vi "MC_8_28_12a_JW.vi"() -> ()   [LabVIEW 2011]
uses:
  <vilib>/Utility/file.llb/Read From Spreadsheet File (string).vi
  <vilib>/Utility/inputDevices.llb/keyboardAcquire.vi
  <vilib>/Utility/file.llb/Write To Spreadsheet File (DBL).vi
  <vilib>/Utility/file.llb/Write To Spreadsheet File (string).vi
  <vilib>/regexp/Match Regular Expression.xnode
panel:
  out "Vg Column":dbl[](array[numeric])
  out "Data Length":dbl
  in  "default (0 dbl) 6":ext format="%.2e"
  in  "default (0 dbl) 5":ext format="%.2e"
  in  "default (0 dbl) 4":ext format="%.2e"
  in  "default (0 dbl) 3":ext format="%.2e"
  in  "default (0 dbl)":ext format="%.2e"
  out "X Axis Display Type":string
  out "Opj X Axis":string
  in  "Room Temp":dbl=294.0
  out "No Image 2":path=path "\\\\acad1\\physics/Jurchescu-group/JW-PD/Image Not Found.png"
  out "Save1 Array":string[][](array[string])
  out "Lin Vd":dbl
  out "Lin-Vg Array-Used":dbl[](array[numeric])
  out "Lin Id-Used":dbl[](array[numeric])
  out "Rec: Comments":string
  out "Folder Index":dbl caption="Length"
  out "Current \nRecord":string[](array[string])
  out "Transformer \nHeaders":string[](array[string])
  out "Current Device ID":string
  out "Column":string
  out "Row":string
  out "Rec: Concentration":dbl
  out "Rec: Solvent":string
  out "Rec: Method":string
  in  "?":T1(tab)
  in  "Transport File":path
  out "Transport Folder":path
  out "Rec: Material":string
  out "Accel (RPM/s):":dbl
  in  "Transfer File":path
  out "Transfer Folder":path
  in  "Image Folder":path
  out "Image File":path=path "D:/UserData/Desktop/Jeremy/WFU/Research/Programs/VI mods/Image Not Found.png"
  in  "Manual Comments":bool
  in  "Comments:":string
  out "Calc: On/Off":dbl caption="On/Off-Sat" format="%#.2e"
  out "Calc: Off I-Sat":dbl caption="Off I-Sat" format="%#.2e"
  in  "Manuel-Dielectric":bool
  in  "Manuel-Length":bool
  out "Calc: VT-Lin":dbl
  out "New: VT-Lin":dbl
  out "Rec: VT-Lin":dbl caption="VT-Lin" format="%#_3g"
  out "Calc: Trap Density-STS":dbl format="%#.2e"
  out "New: Trap Density-STS":dbl format="%#.2e"
  out "Rec: Trap Density-STS":dbl caption="N-Sat (STS)" format="%#.2e"
  out "Calc: Trap Density-VT":dbl format="%#.2e"
  out "New: Trap Density-VT":dbl format="%#.2e"
  out "Rec: Trap Density-VT":dbl caption="N-Sat (VT)" format="%#.2e"
  out "Calc: Mobility-Lin":dbl format="%#.2e"
  out "New: Mobility-Lin":dbl format="%#_4e"
  out "Rec: Mobility-Lin":dbl caption="Mobility-Lin" format="%#_3e"
  out "Calc: Mobility-Sat":dbl format="%#.2e"
  out "Rec: Length":dbl caption="Length" format="%#_3g"
  out "Rec: Width":dbl caption="Width" format="%#_4g"
  out "Rec: Dielectric (d)":dbl caption="Dielectric (d)" format="%#_3g"
  in  "Cancel Button":bool
  in  "Up Button":bool
  in  "Down Button":bool
  out "Data Name:":string
  in  "Save Changes?":bool
  in  "New: Dielectric":dbl
  in  "New: Length":dbl
  in  "New: Width":dbl
  out "New: Mobility-Sat":dbl format="%#.2e"
  in  "Blank Button":bool
  in  "Zoom":i16(slide)=-3 scale=-5.0..5.0
  out "Image Out 2":T2(plugin-control)
  out "Image Out":T2(plugin-control)
  in  "Magnification":u16(ring) items=["5x", "10x", "20x", "50x", "80x"]
  out "Total Width":dbl
  out "Distances":dbl[](array[numeric])
  in  "Undo Button":bool
  in  "Remove Button":bool
  out "Rec: Mobility-Sat":dbl caption="Mobility-Sat" format="%#.2e"
  in  "Export":bool
  out "Calc: VT-Sat":dbl format="%#.2g"
  out "New: VT-Sat":dbl format="%#.2g"
  in  "Manual-Width":bool caption="Manual"
  out "Calc: STS":dbl format="%#.2g"
  out "New: STS":dbl format="%#.2g"
  out "Rec: VT-Sat":dbl caption="VT-Sat" format="%#.2g"
  out "Rec: STS":dbl caption="STS-Sat" format="%#.2g"
  out "Rec: On/Off":dbl caption="On/Off-Sat" format="%#.2e"
  in  "Save Changes? 2":bool
  in  "Save Changes? 3":bool
  out "Rec: Temp":dbl caption="Sample Temp" format="%.1f"
  in  "New: Temp":dbl format="%.1f"
  out "Rec: Off I-Sat":dbl caption="Off I-Sat" format="%#.2e"
  in  "Independant Variable":string(combo)="Length (um):"
  in  "Transfer Plots":T3(tab)=enum."Saturation"
  in  "Lin-Trans Slider":dbl(slide) step=1.0 scale=-22.0..89.0 scale format="%#_1p"
  out "Sqrt-Lin":cluster{dbl[], dbl[]}[](graph)
  in  "Next Sqrt Lin":bool
  in  "Previous Sqrt Lin":bool
  in  "Sat-Trans Slider":dbl(slide) step=1.0 scale=-40.0..40.0 scale format="%#_1p"
  out "Sqrt-Sat":cluster{dbl[], dbl[]}[](graph)
  in  "Previous Sqrt Sat":bool
  in  "Next Sqrt Sat":bool
  out "Raw- Lin":cluster{dbl[], dbl[]}[](graph)
  out "Raw- Sat":cluster{dbl[], dbl[]}[](graph)
  in  "Log Plots":enum32{"Linear", "Saturation", "Transport"}(tab)=enum."Saturation"
  in  "Lin-Log Slider":dbl(slide) step=1.0 scale=-1.0..82.0 scale format="%#_1p"
  in  "Previous Log Lin":bool
  in  "Next Log Lin":bool
  out "Log-Lin":cluster{dbl[], dbl[]}[](graph)
  in  "Sat-Log Slider":dbl(slide) step=1.0 scale=-1.0..82.0 scale format="%#_1p"
  in  "Previous Log Sat":bool
  in  "Next Log Sat":bool
  out "Sat-Log":cluster{dbl[], dbl[]}[](graph)
  out "Transport":cluster{dbl[], dbl[]}[](graph)
  in  "Manual-Temp":bool caption="Manual"
  out "Date Created":string caption="Fabricated"
  out "Date Recorded":string="Date Recorded" caption="Measured"
  out "Image Name":string
  out "Index":string
  in  "Num Pts":dbl=5.0
  in  "NumPoints Log":dbl=5.0 caption="Num Pts"
  in  "Ring":u16(ring) items=["Extra Small", "Small", "Medium", "Large", "Extra Large"]
  in  "Transport Line Color":u32(colorbox)
  in  "Origin Project File":path=path "\\\\acad1\\physics/Jurchescu-group/JW-PD/Group Library/Origin Project Files/DeviceData_8_10_12a_JW.opj"
  in  "No Image File":path=path "\\\\acad1\\physics/Jurchescu-group/JW-PD/Mega Awesome/Image Not Found.png"
  in  "Ramp (s):":dbl=3.0
  in  "Fabricator:":string="NaN"
  in  "Sample #:":dbl=1.0
  in  "Wait Time (s):":dbl=nan
  in  "RPM:":dbl=nan
  in  "Time (s):":dbl=nan
  in  "Room Temp (F):":dbl=nan
  in  "Relative Humidity (%):":dbl=nan
  in  "Solution Temp (C):":dbl=nan
  in  "# Drops*:":dbl=inf
  in  "Surface Treatment:":string="NaN"
  in  "Treatment Concentration (mM):":dbl=nan
  out "String":string
  out "Index 2":dbl
  out "Sat Id-Log-Used":dbl[](array[numeric])
  out "Vg Array-Log-Used":dbl[](array[numeric])
  out "ROI Descriptor out":T4 {"Contours"."Type" items=["No Selection", "Point", "Line", "Rectangle", "Oval", "Polygon", "Freehand Region", "Annulus", "Unused2", "Unused3", "Broken Line", "Freehand Line", "Rotated Rectangle"]}
  out "ROI Descriptor":T4 {"Contours"."Type" items=["No Selection", "Point", "Line", "Rectangle", "Oval", "Polygon", "Freehand Region", "Annulus", "Unused2", "Unused3", "Broken Line", "Freehand Line", "Rotated Rectangle"]}
  out "Numeric 3":dbl
  out "Array 6":dbl[][](array[numeric])
  out "Cluster":T5
  out "Array 5":dbl[](array[numeric])
  out "Array 4":dbl[](array[numeric])
  out "Array 3":dbl[](array[numeric])
  out "Numeric 2":dbl
  out "Numeric":dbl
  out "Sat Id-Used":dbl[](array[numeric])
  out "Sat Vg Array-Used":dbl[](array[numeric])
  out "MobVi Index":dbl
  in  "Row Start":dbl=20.0
  # "Data Locations"
  # "Transfer Location"
  # "Image Location"
  # "Recorded"
  # "Calculated"
  # "Re-Calculated"
  # "Manual"
  # "Used points display at y=0"
  # "Slider\nDoesn't\nWork"
  # "Slider\nDoesn't\nWork"
  # "No new points displayed"
  # "Sample Properties"
  # "*     Inf = Full coverage\n   NaN = Unknown or Not Applicable"
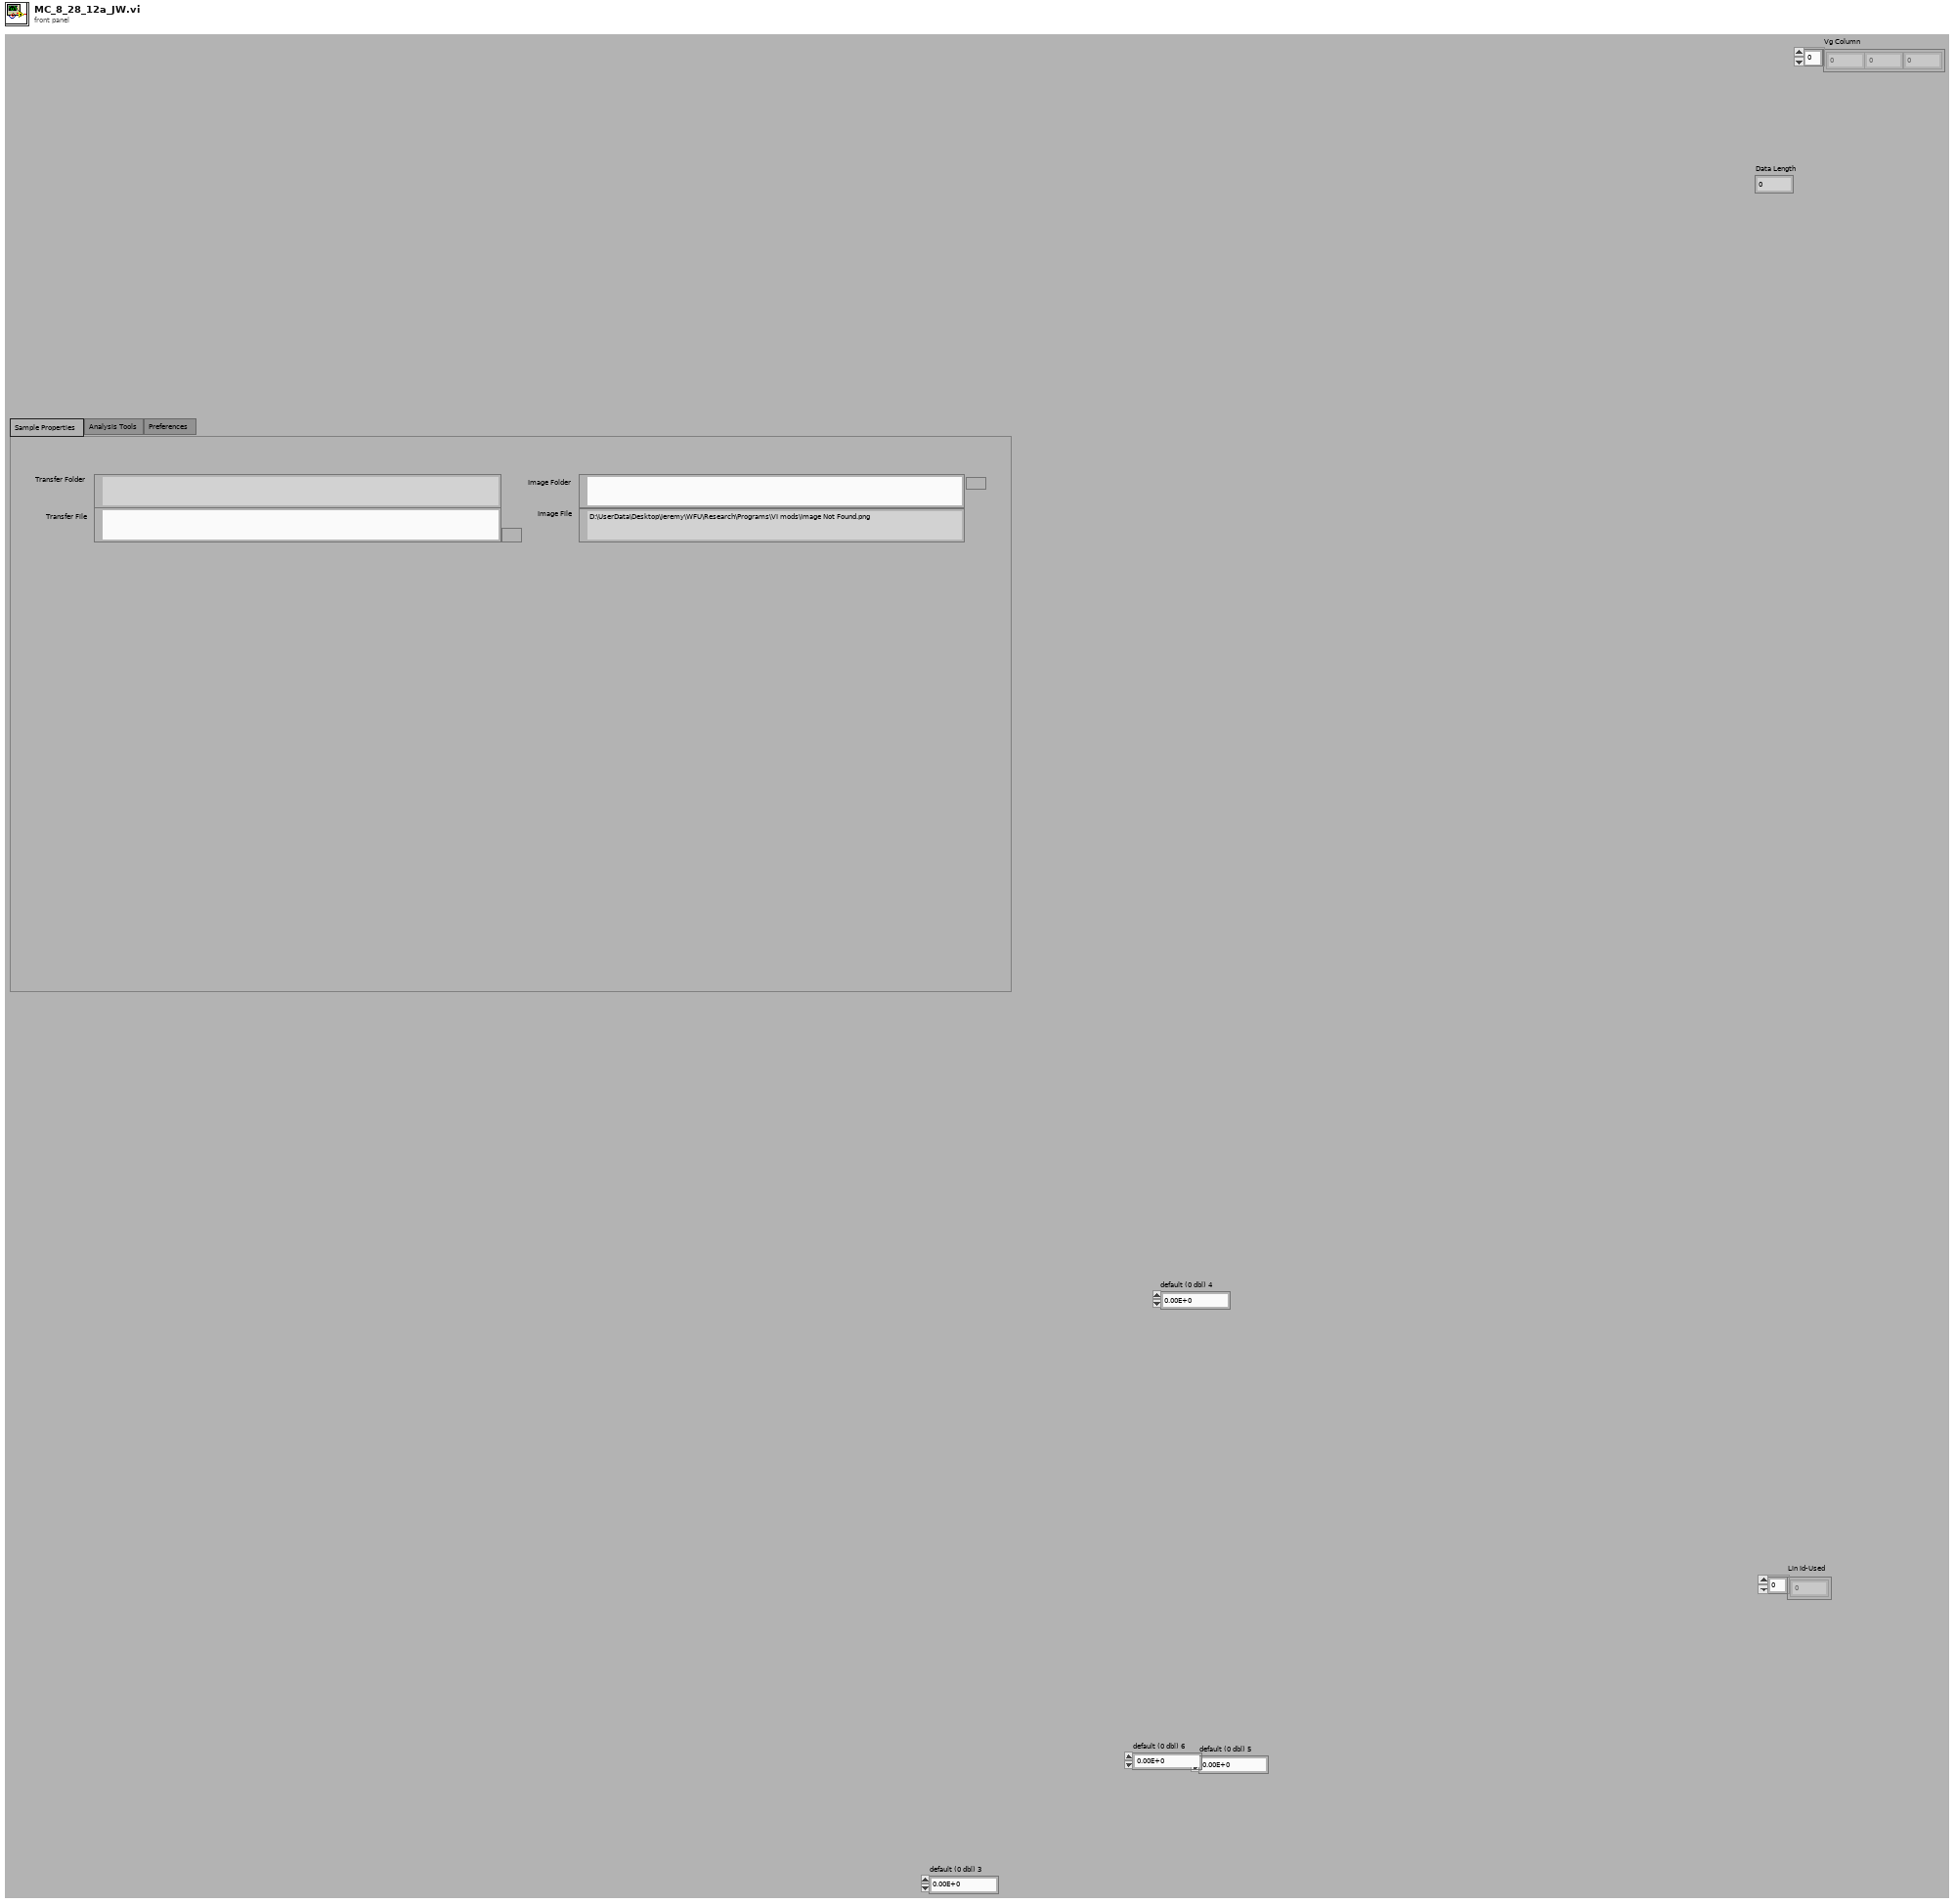
[diagram p1: front panel]
types:
  T1 = enum32{"Sample Properties", "Analysis Tools", "Preferences", "Current Database"}
  T2 = typedef "IMAQ Image.ctl" = refnum<image>
  T3 = enum32{"Linear", "Saturation", "Raw-Linear", "Raw-Saturation"}
  T4 = typedef "ROI Descriptor" = cluster{"Global Rectangle":i32[], "Contours":cluster{"ID":enum32{"External", "Internal"}, "Type":u32, "Coordinates":i32[]}[]}
  T5 = cluster{"Numeric":dbl, "Numeric 2":dbl, "Numeric 3":dbl, "Numeric 4":dbl}
  T6 = cluster{"Mobility-Sat":dbl, "Moblitity-Lin":dbl, "On/Off":dbl, "Off Current":dbl, "Vt-Sat":dbl, "STS":dbl, "Trap Density-VT":dbl, "Trap Density-STS":dbl}
  T7 = cluster{"Date Recorded":string, "Index":string, "Length":dbl, "Width":dbl, "Sample Temp":dbl}
  T8 = cluster{"Date Created":string, "Material":string, "Solvent":string, "Concentration":dbl, "Method":string, "Dielectric (nm)":dbl, "Treatment":string, "Comments":string}
  T9 = cluster{"Sat Vg Used":dbl[], "Sat Log(Id) Used":dbl[], "Lin Vg Used":dbl[], "Lin Log(Id) Used":dbl[], "STS Index-Sat":dbl, "STS Index-Lin":dbl}
  T10 = cluster{"Sat Vg Used":dbl[], "Sat Sqrt(Id) Used ":dbl[], "Lin Vg Used":dbl[], "Lin Sqrt(Id) Used":dbl[], "Index-Lin":dbl, "Index-Sat":dbl}
  T11 = cluster{"Raw Sat":cluster{dbl[], dbl[]}[], "Sqrt Sat":cluster{dbl[], dbl[]}[], "Log Sat":cluster{dbl[], dbl[]}[], "Raw Lin":cluster{dbl[], dbl[]}[], "Sqrt Lin":cluster{dbl[], dbl[]}[], "Log Lin":cluster{dbl[], dbl[]}[]}
  T12 = cluster{"Mobility-Sat":dbl, "Vt-Sat":dbl, "Mobility-Lin":dbl, "Vt-Lin":dbl, "Off I-Sat":dbl, "On/Off I-Sat":dbl}
  T13 = cluster{"[0]":cluster{dbl[], dbl[]}, "[1]":cluster{dbl[], dbl[]}, "[2]":cluster{dbl[], dbl[]}, "[3]":cluster{dbl[], dbl[]}, "[4]":cluster{dbl[], dbl[]}, "[5]":cluster{dbl[], dbl[]}, "[6]":cluster{dbl[], dbl[]}, "[7]":cluster{dbl[], dbl[]}, "[8]":cluster{dbl[], dbl[]}}
  T14 = cluster{"Global Rectangle":i32[], "Contours":cluster{"Contour Type":u32, "ROI Type":u32, "Points":i32[]}[]}
  T15 = typedef "LVBoundsTypeDef.ctl" = cluster{"Width":u32, "Height":u32}
  T16 = enum16{"0", "1", "2", "3", "4", "5", "6", "7", "8", "9", "A", "B", "C", "D", "E", "F", "G", "H", "I", "J", "K", "L", "M", "N", "O", "P", "Q", "R", "S", "T", "U", "V", "W", "X", "Y", "Z", "F1", "F2", "F3", "F4", "F5", "F6", "F7", "F8", "F9", "F10", "F11", "F12", "F13", "F14", "F15", "ADD", "BACK", "BACKSLASH", "CAPITAL", "COMMA", "DECIMAL", "DELETE", "DIVIDE", "DOWN", "END", "EQUALS", "ESCAPE", "GRAVE (`)", "HOME", "INSERT", "LBRACKET", "LCONTROL", "LEFT", "L ALT", "LSHIFT", "LWIN", "MINUS", "MULTIPLY", "NEXT", "NUMLOCK", "NUMPAD_0", "NUMPAD_1", "NUMPAD_2", "NUMPAD_3", "NUMPAD_4", "NUMPAD_5", "NUMPAD_6", "NUMPAD_7", "NUMPAD_8", "NUMPAD_9", "PAUSE", "PERIOD", "PRIOR (PG UP)", "RBRACKET", "RCONTROL", "RETURN", "RIGHT", "R ALT", "RSHIFT", "RWIN", "SCROLL", "SEMICOLON", "SLASH", "SPACE", "SUBTRACT", "TAB", "UP", "ENTER (num pad)", "' (quote)"}[]
  T17 = enum16{"0", "1", "2", "3", "4", "5", "6", "7", "8", "9", "A", "B", "C", "D", "E", "F", "G", "H", "I", "J", "K", "L", "M", "N", "O", "P", "Q", "R", "S", "T", "U", "V", "W", "X", "Y", "Z", "F1", "F2", "F3", "F4", "F5", "F6", "F7", "F8", "F9", "F10", "F11", "F12", "F13", "F14", "F15", "ADD", "BACK", "BACKSLASH", "CAPITAL", "COMMA", "DECIMAL", "DELETE", "DIVIDE", "DOWN", "END", "EQUALS", "ESCAPE", "GRAVE (`)", "HOME", "INSERT", "LBRACKET", "LCONTROL", "LEFT", "L ALT", "LSHIFT", "LWIN", "MINUS", "MULTIPLY", "NEXT", "NUMLOCK", "NUMPAD_0", "NUMPAD_1", "NUMPAD_2", "NUMPAD_3", "NUMPAD_4", "NUMPAD_5", "NUMPAD_6", "NUMPAD_7", "NUMPAD_8", "NUMPAD_9", "PAUSE", "PERIOD", "PRIOR (PG UP)", "RBRACKET", "RCONTROL", "RETURN", "RIGHT", "R ALT", "RSHIFT", "RWIN", "SCROLL", "SEMICOLON", "SLASH", "SPACE", "SUBTRACT", "TAB", "UP", "ENTER (num pad)", "' (quote)"}
  T18 = cluster{"Contour Type":u32, "ROI Type":u32, "Points":i32[]}[]
  T19 = cluster{i32[], cluster{"Contour Type":u32, "ROI Type":u32, "Points":i32[]}[]}
  T20 = cluster{"Independant  Variable Indicator":string, "Parameter String Indicator":string}
  T21 = cluster{string, sgl, bool, bool, bool, bool, bool, bool, i32}
  T22 = cluster{i32, cluster{string, sgl, bool, bool, bool, bool, bool, bool, i32}, i32, i32}
  T23 = cluster{"Contour Type":u32, "ROI Type":u32, "Points":i32[]}
  T24 = cluster{"Points[0]":i32, "Points[1]":i32, "Points[2]":i32, "Points[3]":i32, "Points[4]":i32, "Points[5]":i32, "Points[6]":i32, "Points[7]":i32, "Points[8]":i32}
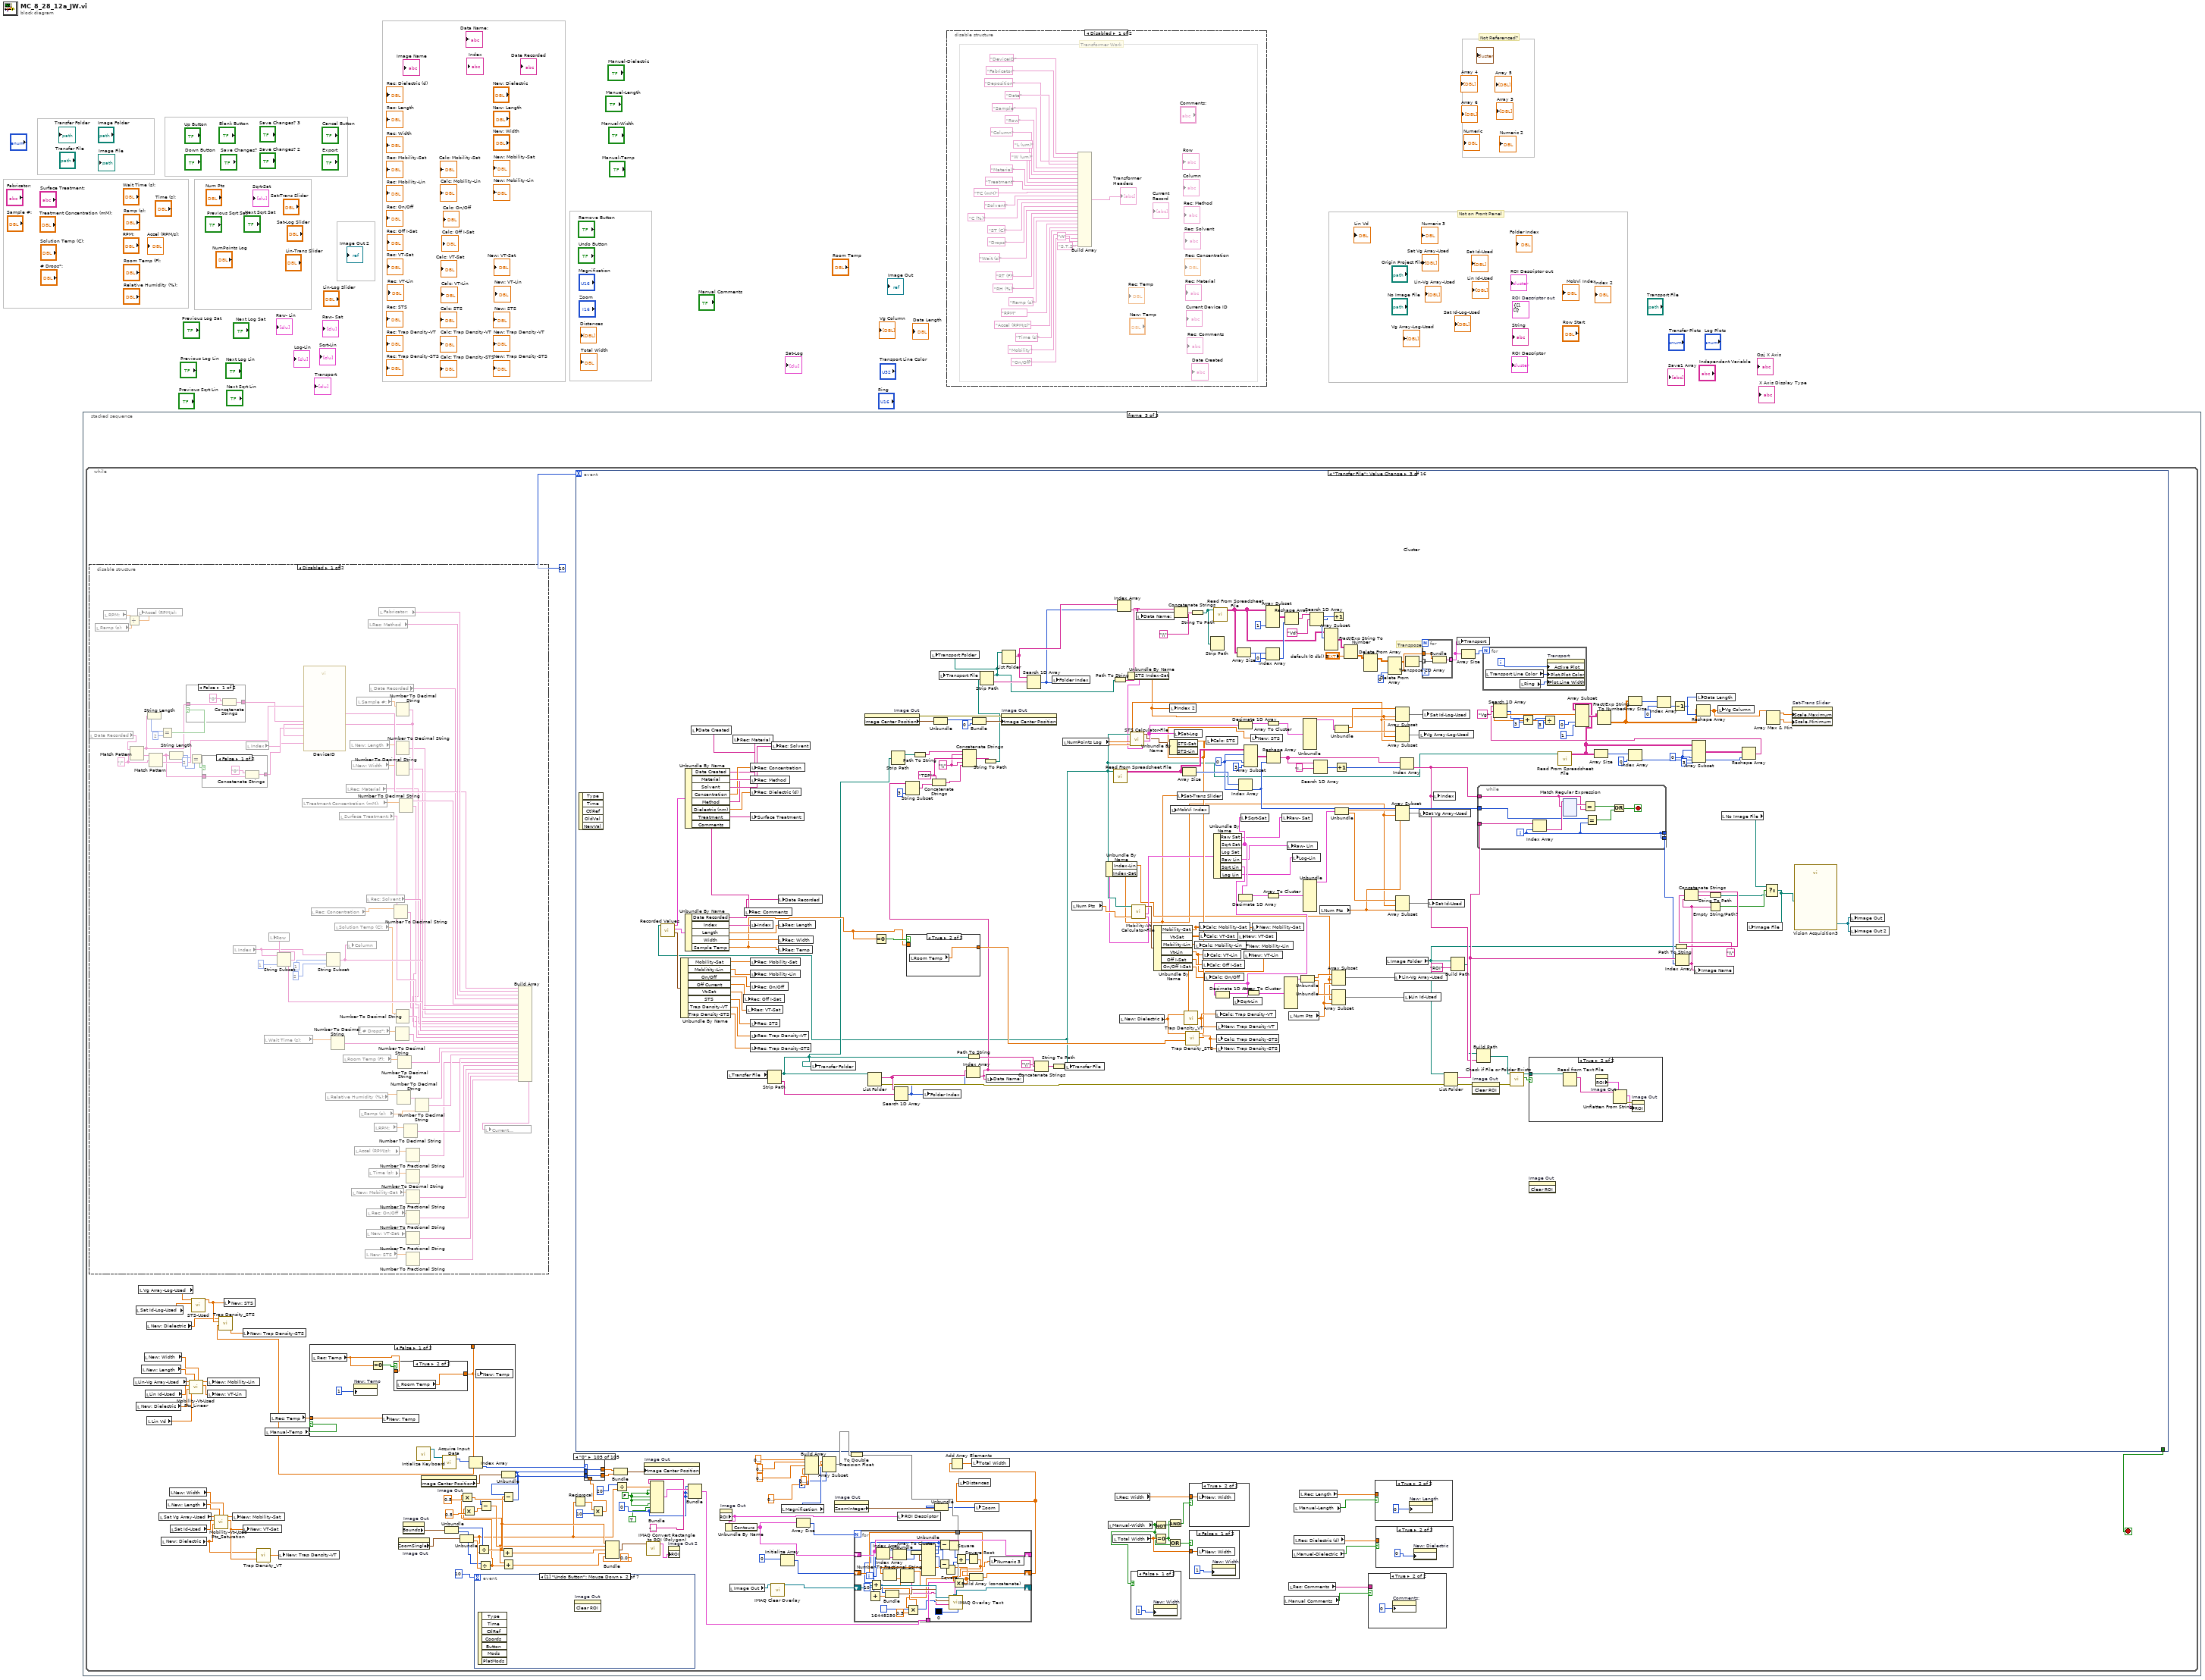
[diagram p0: block diagram]
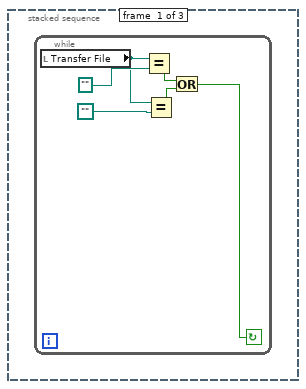
[diagram p3: hidden frame]
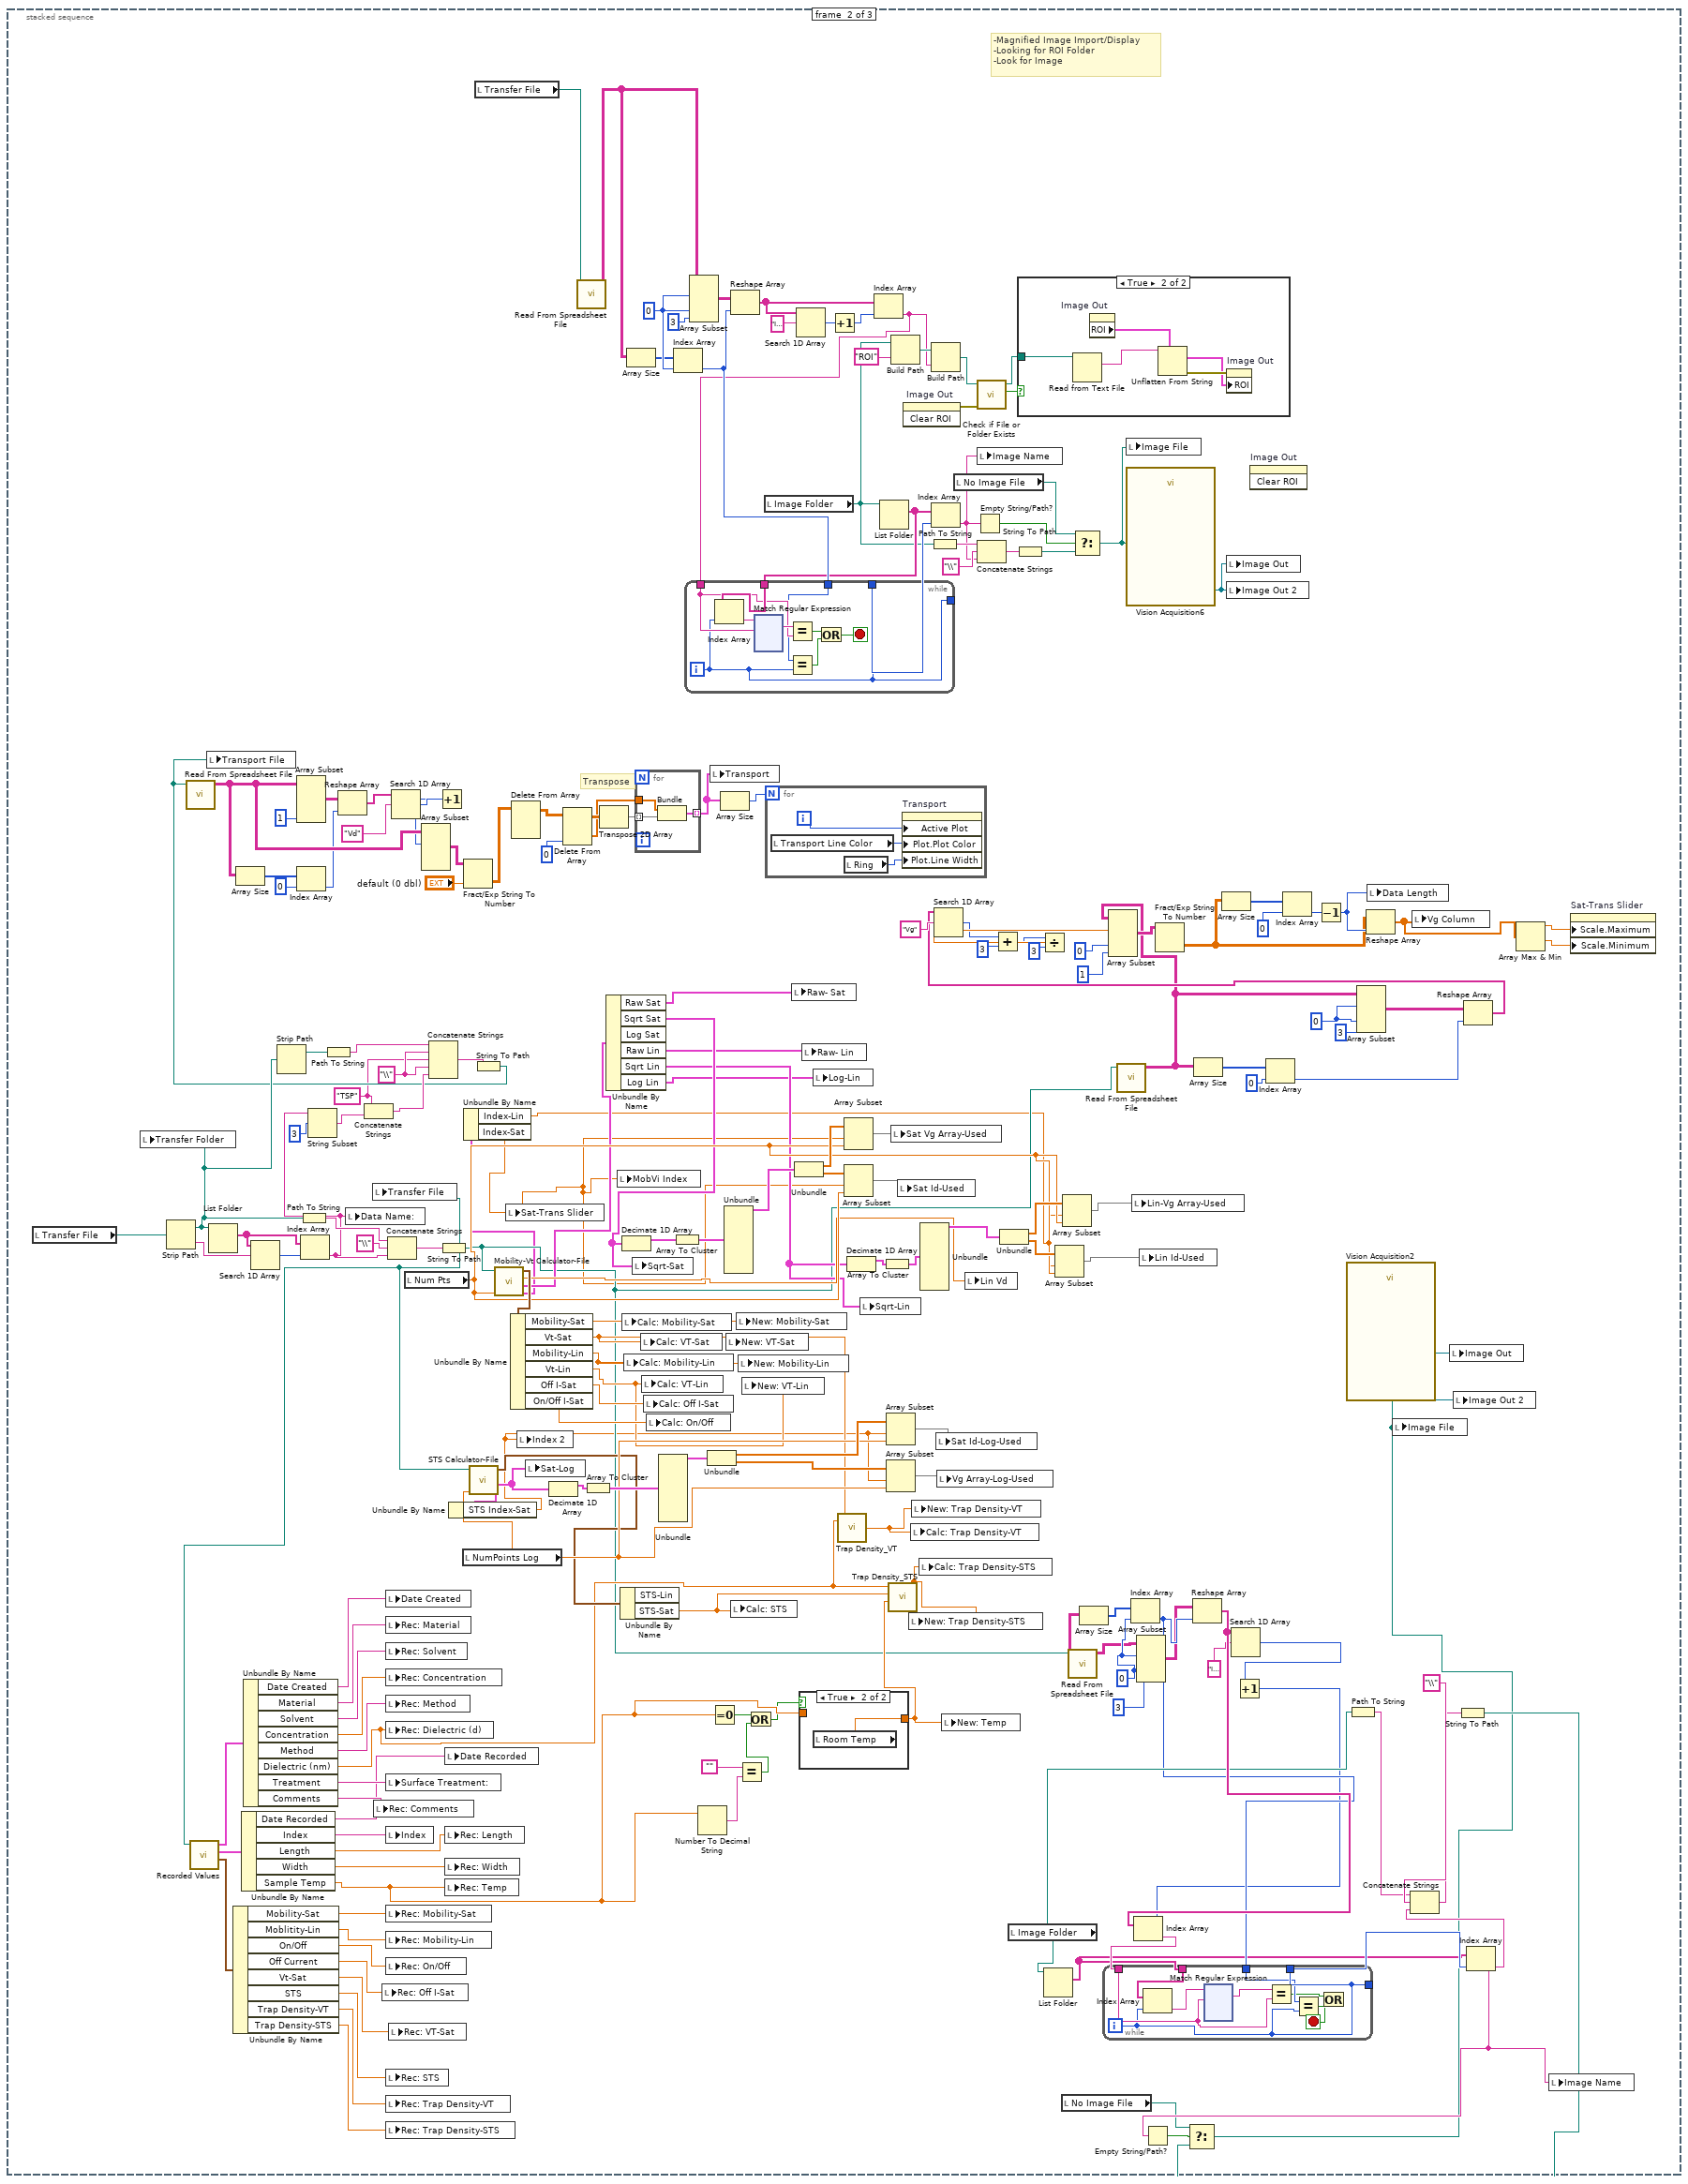
[diagram p4: hidden frame]
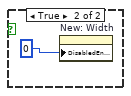
[diagram p10: hidden frame]
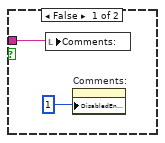
[diagram p11: hidden frame]
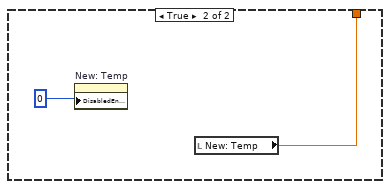
[diagram p13: hidden frame]
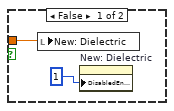
[diagram p14: hidden frame]
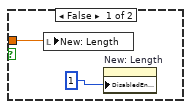
[diagram p15: hidden frame]
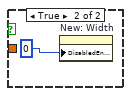
[diagram p17: hidden frame]
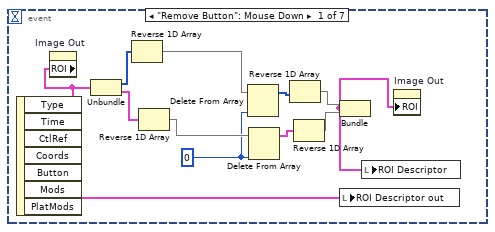
[diagram p18: hidden frame]
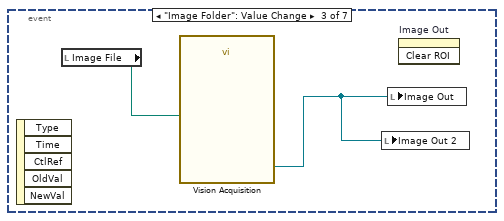
[diagram p19: hidden frame]
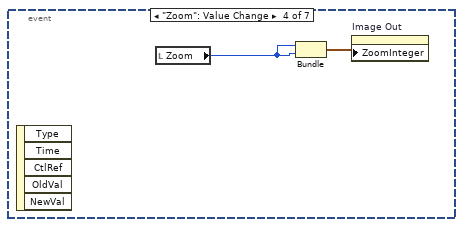
[diagram p20: hidden frame]
diagram:
  (unwired) T4 {"Global Rectangle"=[], "Contours"=[]}  # ROI Descriptor out
  # "Not Referenced?"
  # "Not on Front Panel"
  n1 = stacked-sequence {
    frame #0 {
      n2 = while {
        stop <- w1 continue-if-true
        n3 = local read "Transfer File"() -> (w3:path)
        n4 = Equal?(x=w3, y=path "") -> (x = y?=w5:bool)
        n5 = Equal?(x=w3, y=path "") -> (x = y?=w4:bool)
        n6 = Or(x=w5, y=w4) -> (x .or. y?=w1:bool)
      }
    }
    frame #1 {
      w34 = 0
      w40 = "\\"
      w39 = "TSP"
      w166 = 0
      w189 = 0
      # "Transpose"
      # "-Magnified Image Import/Display\n-Looking for ROI Folder\n-Look for Image"
      n7 = local read "Transfer File"() -> (w170:path)
      n8 = Strip Path(path=w170) -> (stripped path=w49:path, name=w157:string)
      n9 = local write "Transfer Folder"(w49) -> ()
      n10 = List Folder(path=w49) -> (filenames=w161:string[])  [unwired: 3 in, 3 out]
      n11 = Search 1D Array(1D array=w161, element=w157) -> (index of element=w160:i32)  [unwired: 1 in]
      n12 = Strip Path(path=w49) -> (stripped path=w45:path)  [unwired: 1 out]
      n13 = Path To String(path=w49) -> (string=w156:string)
      n14 = Index Array(array=w161, index=w160) -> (element=w48:string)
      n15 = String Subset(string=w48, offset (0)=3) -> (substring=w46:string)  [unwired: 1 in]
      n16 = Path To String(path=w45) -> (string=w41:string)
      n17 = local write "Data Name:"(w48) -> ()
      n18 = Concatenate Strings(w39, w46) -> (w44:string)
      n19 = Concatenate Strings(w156, "\\", w48) -> (w158:string)
      n20 = local read "Num Pts"() -> (w97:dbl)
      n21 = Concatenate Strings(w41, w40, w39, w40, w44) -> (w43:string)
      n22 = String To Path(string=w158) -> (path=w12:path)
      n23 = call "Recorded Values.vi"("Path"=w12) -> ("Recorded Char"=w125:T6, "Recorded Prop"=w124:T7, "Fabrication Prop"=w126:T8)  [unwired: 8 in]
      n24 = Unbundle By Name(w125) -> ("Mobility-Sat"=w113:dbl, "Moblitity-Lin"=w112:dbl, "On/Off"=w111:dbl, "Off Current"=w110:dbl, "Vt-Sat"=w79:dbl, "STS"=w109:dbl, "Trap Density-VT"=w108:dbl, "Trap Density-STS"=w107:dbl)
      n25 = Unbundle By Name(w124) -> ("Date Recorded"=w117:string, "Index"=w116:string, "Length"=w115:dbl, "Width"=w114:dbl, "Sample Temp"=w85:dbl)
      n26 = Unbundle By Name(w126) -> ("Date Created"=w106:string, "Material"=w123:string, "Solvent"=w122:string, "Concentration"=w121:dbl, "Method"=w120:string, "Dielectric (nm)"=w89:dbl, "Treatment"=w119:string, "Comments"=w118:string)
      n27 = local write "Transfer File"(w12) -> ()
      n28 = local write "Rec: Comments"(w118) -> ()
      n29 = local write "Rec: Off I-Sat"(w110) -> ()
      n30 = local write "Date Created"(w106) -> ()
      n31 = local write "Rec: Material"(w123) -> ()
      n32 = local write "Rec: Solvent"(w122) -> ()
      n33 = local write "Rec: Concentration"(w121) -> ()
      n34 = local write "Rec: Method"(w120) -> ()
      n35 = local write "Rec: Dielectric (d)"(w89) -> ()
      n36 = local write "Surface Treatment:"(w119) -> ()
      n37 = local write "Index"(w116) -> ()
      n38 = local write "Rec: Mobility-Sat"(w113) -> ()
      n39 = local write "Rec: Mobility-Lin"(w112) -> ()
      n40 = local write "Rec: On/Off"(w111) -> ()
      n41 = local write "Rec: STS"(w109) -> ()
      n42 = local write "Rec: Trap Density-VT"(w108) -> ()
      n43 = local write "Rec: Trap Density-STS"(w107) -> ()
      n44 = local write "Rec: VT-Sat"(w79) -> ()
      n45 = local write "Date Recorded"(w117) -> ()
      n46 = local write "Rec: Length"(w115) -> ()
      n47 = local write "Rec: Width"(w114) -> ()
      n48 = local write "Rec: Temp"(w85) -> ()
      n49 = local read "NumPoints Log"() -> (w104:dbl)
      n50 = call "STS Calculator-File.vi"("NumPts"=w104, "Path"=w12) -> ("Used Points"=w8:T9, "XY Graph-Sat"=w38:cluster{dbl[], dbl[]}[], "Ouput"=w103:cluster{"STS-Sat":dbl, "STS-Lin":dbl})  [unwired: 6 in, 1 out]
      n51 = Unbundle By Name(w8) -> ("STS Index-Sat"=w7:dbl)
      n52 = String To Path(string=w43) -> (path=w42:path)
      n53 = call-poly <vilib>:"Read From Spreadsheet File.vi"("file path (dialog if empty)"=w42) -> ("all rows"=w63:string[][])  [unwired: 6 in, 4 out]
      n54 = local write "Transport File"(w42) -> ()
      n55 = Array Size(array=w63) -> (size(s)=w69:i32[])
      n56 = Array Subset(array=w63, length (col)=1) -> (w65:string[][])  [unwired: 3 in]
      n57 = Index Array(array=w69, index=0) -> (element=w58:i32)
      n58 = Reshape Array(w65, w58) -> (w64:string[])
      n59 = Search 1D Array(1D array=w64, element="Vd") -> (index of element=w62:i32)  [unwired: 1 in]
      n60 = Increment(x=w62) -> (x+1=w61:i32)
      n61 = Array Subset(array=w63, index (row)=w61) -> (w59:string[][])  [unwired: 3 in]
      n62 = Fract/Exp String To Number(string=w59, default (0 dbl)="default (0 dbl)") -> (number=w51:ext[][])  [unwired: 2 in, 1 out]
      n63 = local read "Transfer File"() -> (w184:path)
      n64 = call "Mobility-Vt Calculator-File.vi"("NumPts"=w97, "Path"=w12) -> ("Used Points"=w11:T10, "Graph Cluster"=w70:T11, "Lin Vd"=w94:dbl, "Output"=w105:T12)  [unwired: 6 in]
      n65 = Unbundle By Name(w11) -> ("Index-Lin"=w9:dbl, "Index-Sat"=w10:dbl)
      n66 = local write "Sat-Trans Slider"(w10) -> ()
      n67 = Unbundle By Name(w105) -> ("Mobility-Sat"=w88:dbl, "Vt-Sat"=w87:dbl, "Mobility-Lin"=w78:dbl, "Vt-Lin"=w76:dbl, "Off I-Sat"=w93:dbl, "On/Off I-Sat"=w77:dbl)
      n68 = Delete From Array(array=w51) -> (array with subset deleted=w50:ext[][])  [unwired: 3 in, 1 out]
      n69 = local write "Index 2"(w7) -> ()
      n70 = local write "Sat-Log"(w38) -> ()
      n71 = Decimate 1D Array(w38) -> (w148:cluster{dbl[], dbl[]}[])  [unwired: 1 out]
      n72 = Delete From Array(array=w50, index (col)=0 ("Deaktivierter Index (Spalte)")) -> (deleted portion=w55:ext[], array with subset deleted=w56:ext[][])  [unwired: 2 in]
      n73 = call-poly <vilib>:"Read From Spreadsheet File.vi"("file path (dialog if empty)"=w184) -> ("all rows"=w187:string[][])  [unwired: 6 in, 4 out]
      n74 = Array To Cluster(array=w148) -> (cluster=w150:T13)
      n75 = Transpose 2D Array(2D array=w56) -> (transposed array=w57:ext[][])
      n76 = Unbundle By Name(w70) -> ("Raw Sat"=w73:cluster{dbl[], dbl[]}[], "Sqrt Sat"=w75:cluster{dbl[], dbl[]}[], "Raw Lin"=w72:cluster{dbl[], dbl[]}[], "Sqrt Lin"=w74:cluster{dbl[], dbl[]}[], "Log Lin"=w71:cluster{dbl[], dbl[]}[])  [unwired: 1 out]
      n77 = local write "MobVi Index"(w10) -> ()
      n78 = Unbundle By Name(w103) -> ("STS-Sat"=w92:dbl)  [unwired: 1 out]
      n79 = Decimate 1D Array(w75) -> (w183:cluster{dbl[], dbl[]}[])  [unwired: 1 out]
      n80 = local write "Calc: Mobility-Sat"(w88) -> ()
      n81 = local write "Calc: Mobility-Lin"(w78) -> ()
      n82 = Array Size(array=w187) -> (size(s)=w188:i32[])
      n83 = local write "Sqrt-Sat"(w75) -> ()
      n84 = for {
        tunnel: w55 -> [w205]
        tunnel: w57 -> [w206] mode=indexing
        tunnel: [w204] -> w53 mode=indexing
        n85 = Bundle(w205, w206) -> (w204:cluster{ext[], ext[]})  [unwired: 1 in]
      }
      n86 = local write "Calc: VT-Sat"(w87) -> ()
      n87 = local write "Calc: VT-Lin"(w76) -> ()
      n88 = local write "Calc: Off I-Sat"(w93) -> ()
      n89 = local write "Calc: On/Off"(w77) -> ()
      n90 = Unbundle(w150) -> ("[0]"=w149:cluster{dbl[], dbl[]})  [unwired: 8 out]
      n91 = Array To Cluster(array=w183) -> (cluster=w181:T13)
      n92 = Index Array(array=w188, index=w189) -> (element=w195:i32)
      n93 = Array Subset(array=w187, index (row)=w189, index (col)=w189, length (col)=3) -> (w186:string[][])  [unwired: 1 in]
      n94 = Number To Decimal String(number=w85) -> (decimal integer string=w83:string)  [unwired: 1 in]
      n95 = Unbundle(w149) -> (w146:dbl[], w145:dbl[])
      n96 = local write "Transport"(w53) -> ()
      n97 = Equal To 0?(x=w85) -> (x = 0?=w84:bool)
      n98 = Array Size(array=w53) -> (size(s)=w52:i32)
      n99 = Unbundle(w181) -> ("[0]"=w182:cluster{dbl[], dbl[]})  [unwired: 8 out]
      n100 = local write "New: VT-Sat"(w87) -> ()
      n101 = Reshape Array(w186, w195) -> (w200:string[])
      n102 = local write "Calc: STS"(w92) -> ()
      n103 = local write "New: Mobility-Sat"(w88) -> ()
      n104 = Equal?(x="", y=w83) -> (x = y?=w81:bool)
      n105 = local write "New: Mobility-Lin"(w78) -> ()
      n106 = local write "New: VT-Lin"(w76) -> ()
      n107 = Or(x=w84, y=w81) -> (x .or. y?=w80:bool)
      n108 = local read "Image Folder"() -> (w127:path)
      n109 = for {
        N: w52 -> [_]
        i -> [w203]
        n110 = local read "Transport Line Color"() -> (w202:u32)
        n111 = local read "Ring"() -> (w201:u16)
        n112 = property on="Transport" class="XYGraph (strict)"("Active Plot"=w203, "Plot.Plot Color"=w202, "Plot.Line Width"=w201) -> ()  [unwired: 2 in, 2 out]
      }
      n113 = local write "Raw- Sat"(w73) -> ()
      n114 = Unbundle(w182) -> (w147:dbl[], w151:dbl[])
      n115 = Search 1D Array(1D array=w200, element="Index:") -> (index of element=w192:i32)  [unwired: 1 in]
      n116 = case shown="True" w80 {
        tunnel: [w207 w208] -> w91
        tunnel: w85 -> [w207 _]
        frame False {
        }
        frame True {
          n117 = local read "Room Temp"() -> (w208:dbl)
        }
      }
      n118 = local write "Raw- Lin"(w72) -> ()
      n119 = local write "Log-Lin"(w71) -> ()
      n120 = Increment(x=w192) -> (x+1=w191:i32)
      n121 = call "Trap Density_VT.vi"("VT"=w87, "Dielectric"=w89) -> ("Trap Density-VT"=w86:dbl)
      n122 = Array Subset(array=w147, index=w10, length=w97) -> (w154:dbl[])
      n123 = Array Subset(array=w151, index=w10, length=w97) -> (w155:dbl[])
      n124 = Decimate 1D Array(w74) -> (w102:cluster{dbl[], dbl[]}[])  [unwired: 1 out]
      n125 = local write "Sqrt-Lin"(w74) -> ()
      n126 = Index Array(array=w200, index=w191) -> (element=w128:string)
      n127 = List Folder(path=w127) -> (filenames=w193:string[])  [unwired: 3 in, 3 out]
      n128 = while {
        tunnel: w193 -> [w341]
        tunnel: w128 -> [w339]
        tunnel: [w338] -> _
        tunnel: [w338] -> w194
        tunnel: w195 -> [w337]
        i -> [w338]
        stop <- w334 stop-if-true
        n129 = Index Array(array=w341, index=w338) -> (element=w342:string)
        n130 = xnode "Match Regular Expression"("input string"=w342, "regular expression"=w339) -> ("whole match"=w340:string)  [unwired: 4 in, 4 out]
        n131 = Equal?(x=w340, y=w339) -> (x = y?=w336:bool)
        n132 = Equal?(x=w337, y=w338) -> (x = y?=w335:bool)
        n133 = Or(x=w336, y=w335) -> (x .or. y?=w334:bool)
      }
      n134 = Array To Cluster(array=w102) -> (cluster=w101:T13)
      n135 = Array Subset(array=w146, index=w7, length=w104) -> (w153:dbl[])
      n136 = Array Subset(array=w145, index=w7, length=w104) -> (w152:dbl[])
      n137 = call "Trap Density_STS.vi"("Temp (T) [K]"=w91, "S.T.S. (S)"=w92, "Dielectric"=w89) -> ("Trap Density (N)"=w90:dbl)  [unwired: 8 in]
      n138 = Build Path(base path=w127, name or relative path="ROI") -> (appended path=w130:path)
      n139 = local write "Sat Vg Array-Used"(w154) -> ()
      n140 = local write "Sat Id-Used"(w155) -> ()
      n141 = invoke on="Image Out" class="ImageControl" method="Clear ROI"() -> (error out=w134:errorcluster)  [unwired: 3 in, 2 out]
      n142 = local write "New: Trap Density-STS"(w90) -> ()
      n143 = local write "Calc: Trap Density-VT"(w86) -> ()
      n144 = local write "New: Trap Density-VT"(w86) -> ()
      n145 = local write "Calc: Trap Density-STS"(w90) -> ()
      n146 = Unbundle(w101) -> ("[0]"=w100:cluster{dbl[], dbl[]})  [unwired: 8 out]
      n147 = Path To String(path=w127) -> (string=w197:string)
      n148 = Build Path(base path=w130, name or relative path=w128) -> (appended path=w129:path)
      n149 = Index Array(array=w193, index=w194) -> (element=w144:string)
      n150 = local write "Sat Id-Log-Used"(w153) -> ()
      n151 = local write "Vg Array-Log-Used"(w152) -> ()
      n152 = local write "New: Temp"(w91) -> ()
      n153 = local read "No Image File"() -> (w135:path)
      n154 = local write "Lin Vd"(w94) -> ()
      n155 = Empty String/Path?(string/path=w144) -> (empty?=w143:bool)
      n156 = call <vilib>:"Check if File or Folder Exists.vi"("error in (no error)"=w134, "path"=w129) -> ("file or folder exists?"=w132:bool, "dup path"=w133:path)  [unwired: 7 in, 1 out]
      n157 = local write "Image Name"(w144) -> ()
      n158 = Concatenate Strings(w197, "\\", w144) -> (w198:string)
      n159 = Unbundle(w100) -> (w99:dbl[], w98:dbl[])
      n160 = local read "Image Folder"() -> (w176:path)
      n161 = String To Path(string=w198) -> (path=w142:path)
      n162 = case shown="True" w132 {
        tunnel: w133 -> [_ w209]
        frame False {
        }
        frame True {
          n163 = Read from Text File(file (use dialog)=w209) -> (text=w213:string)  [unwired: 3 in, 3 out]
          n164 = property on="Image Out" class="ImageControl"() -> ("ROI"=w210:T14)  [unwired: 2 in, 2 out]
          n165 = Unflatten From String(type=w210, binary string=w213) -> (value=w211:T14, error out=w212:errorcluster)  [unwired: 3 in, 1 out]
          n166 = property on="Image Out" class="ImageControl"(error in=w212, "ROI"=w211) -> ()  [unwired: 1 in, 2 out]
        }
      }
      n167 = List Folder(path=w176) -> (filenames=w172:string[])  [unwired: 3 in, 3 out]
      n168 = Array Subset(array=w98, index=w9, length=w97) -> (w95:dbl[])
      n169 = local read "No Image File"() -> (w136:path)
      n170 = Array Subset(array=w99, index=w9, length=w97) -> (w96:dbl[])
      n171 = call-poly <vilib>:"Read From Spreadsheet File.vi"("file path (dialog if empty)"=w12) -> ("all rows"=w164:string[][])  [unwired: 6 in, 4 out]
      n172 = Select(t=w135, s=w143, f=w142) -> (s? t:f=w141:path)
      n173 = Array Size(array=w164) -> (size(s)=w165:i32[])
      n174 = call-poly <vilib>:"Read From Spreadsheet File.vi"("file path (dialog if empty)"=w12) -> ("all rows"=w16:string[][])  [unwired: 6 in, 4 out]
      n175 = local write "Image File"(w141) -> ()
      n176 = call "Vision Acquisition6"("Image Path"=w141) -> ("Image Out"=w196:T2)  [unwired: 25 in, 1 out]
      n177 = Index Array(array=w165, index=w166) -> (element=w175:i32)
      n178 = local write "Lin-Vg Array-Used"(w96) -> ()
      n179 = Array Subset(array=w164, index (row)=w166, index (col)=w166, length (col)=3) -> (w163:string[][])  [unwired: 1 in]
      n180 = local write "Lin Id-Used"(w95) -> ()
      n181 = Reshape Array(w163, w175) -> (w180:string[])
      n182 = Array Size(array=w16) -> (size(s)=w35:i32[])
      n183 = local write "Image Out"(w196) -> ()
      n184 = local write "Image Out 2"(w196) -> ()
      n185 = Search 1D Array(1D array=w180, element="Index:") -> (index of element=w169:i32)  [unwired: 1 in]
      n186 = Increment(x=w169) -> (x+1=w168:i32)
      n187 = Index Array(array=w180, index=w168) -> (element=w173:string)
      n188 = while {
        tunnel: w172 -> [w221]
        tunnel: w173 -> [w219]
        tunnel: [w218] -> _
        tunnel: [w218] -> w174
        tunnel: w175 -> [w217]
        i -> [w218]
        stop <- w214 stop-if-true
        n189 = Index Array(array=w221, index=w218) -> (element=w222:string)
        n190 = xnode "Match Regular Expression"("input string"=w222, "regular expression"=w219) -> ("whole match"=w220:string)  [unwired: 4 in, 4 out]
        n191 = Equal?(x=w220, y=w219) -> (x = y?=w216:bool)
        n192 = Equal?(x=w217, y=w218) -> (x = y?=w215:bool)
        n193 = Or(x=w216, y=w215) -> (x .or. y?=w214:bool)
      }
      n194 = invoke on="Image Out" class="ImageControl" method="Clear ROI"() -> ()  [unwired: 3 in, 3 out]
      n195 = Index Array(array=w35, index=0) -> (element=w33:i32)
      n196 = Path To String(path=w176) -> (string=w177:string)
      n197 = Array Subset(array=w16, index (row)=w34, index (col)=w34, length (col)=3) -> (w36:string[][])  [unwired: 1 in]
      n198 = Reshape Array(w36, w33) -> (w18:string[])
      n199 = Search 1D Array(1D array=w18, element="Vg") -> (index of element=w22:i32)  [unwired: 1 in]
      n200 = Add(x=w22, y=3) -> (x+y=w20:i32)
      n201 = Divide(x=w20, y=3) -> (x/y=w27:dbl)
      n202 = Array Subset(array=w16, index (row)=w27, index (col)=0, length (col)=1) -> (w26:string[][])  [unwired: 1 in]
      n203 = Fract/Exp String To Number(string=w26) -> (number=w30:dbl[][])  [unwired: 3 in, 1 out]
      n204 = Array Size(array=w30) -> (size(s)=w17:i32[])
      n205 = Index Array(array=w17, index=0) -> (element=w28:i32)
      n206 = Decrement(x=w28) -> (x-1=w31:i32)
      n207 = Reshape Array(w30, w31) -> (w15:dbl[])
      n208 = local write "Data Length"(w31) -> ()
      n209 = local write "Vg Column"(w15) -> ()
      n210 = Index Array(array=w172, index=w174) -> (element=w139:string)
      n211 = Empty String/Path?(string/path=w139) -> (empty?=w140:bool)
      n212 = Concatenate Strings(w177, "\\", w139) -> (w178:string)
      n213 = String To Path(string=w178) -> (path=w138:path)
      n214 = Select(t=w136, s=w140, f=w138) -> (s? t:f=w137:path)
      n215 = call "Vision Acquisition2"("Image Path"=w137) -> ("Image Out"=w171:T2)  [unwired: 25 in, 1 out]
      n216 = local write "Image File"(w137) -> ()
      n217 = local write "Image Out"(w171) -> ()
      n218 = local write "Image Out 2"(w171) -> ()
      n219 = Array Max & Min(array=w15) -> (max value=w14:dbl, min value=w13:dbl)  [unwired: 2 out]
      n220 = local write "Image Name"(w139) -> ()
      n221 = property on="Sat-Trans Slider" class="Slide (strict)"("Scale.Maximum"=w14, "Scale.Minimum"=w13) -> ()  [unwired: 2 in, 2 out]
    }
    frame #2 {
      n222 = while {
        stop <- w553 stop-if-true
        w503 = FALSE
        w501 = 0
        n223 = disable-structure shown="Disabled" {
          frame Disabled {
            w587 = "/"
            n224 = local read "Date Recorded"() -> (w590:string)
            n225 = local read "Ramp (s):"() -> (w557:dbl)
            n226 = local read "RPM:"() -> (w558:dbl)
            n227 = Divide(x=w558, y=w557) -> (x/y=w556:dbl)
            n228 = Match Pattern(string=w590, regular expression=w587) -> (before substring=w581:string, after substring=w588:string)  [unwired: 1 in, 2 out]
            n229 = local write "Accel (RPM/s):"(w556) -> ()
            n230 = String Length(string=w581) -> (length=w584:i32)
            n231 = Match Pattern(string=w588, regular expression=w587) -> (before substring=w575:string, after substring=w586:string)  [unwired: 1 in, 2 out]
            n232 = Equal?(x=w584, y=2) -> (x = y?=w582:bool)
            n233 = String Length(string=w575) -> (length=w577:i32)
            n234 = case shown="False" w582 {
              tunnel: w581 -> [w627 w629]
              tunnel: [w626 w629] -> w580
              frame False {
                n235 = Concatenate Strings("0", w627) -> (w626:string)
              }
              frame True {
              }
            }
            n236 = Equal?(x=w577, y=2) -> (x = y?=w579:bool)
            n237 = case shown="False" w579 {
              tunnel: w575 -> [w623 w625]
              tunnel: [w622 w625] -> w576
              frame False {
                n238 = Concatenate Strings("0", w623) -> (w622:string)
              }
              frame True {
              }
            }
            n239 = local read "Index"() -> (w560:string)
            n240 = local read "Index"() -> (w574:string)
            n241 = local read "Wait Time (s):"() -> (w620:dbl)
            n242 = String Subset(string=w560, length (rest)=1) -> (substring=w615:string)  [unwired: 1 in]
            n243 = local write "Row"(w615) -> ()
            n244 = local read "Treatment Concentration (mM):"() -> (w568:dbl)
            n245 = local read "Rec: Concentration"() -> (w555:dbl)
            n246 = local read "Relative Humidity (%):"() -> (w565:dbl)
            n247 = String Subset(string=w560, offset (0)=1, length (rest)=2) -> (substring=w616:string)
            n248 = Number To Decimal String(number=w620) -> (decimal integer string=w621:string)  [unwired: 1 in]
            n249 = local read "Solution Temp (C):"() -> (w609:dbl)
            n250 = local read "Surface Treatment:"() -> (w567:string)
            n251 = local read "Room Temp (F):"() -> (w613:dbl)
            n252 = local read "Rec: Material"() -> (w563:string)
            n253 = local write "Column"(w616) -> ()
            n254 = local read "New: Length"() -> (w573:dbl)
            n255 = local read "New: Width"() -> (w572:dbl)
            n256 = local read "New: Mobility-Sat"() -> (w602:dbl)
            n257 = local read "Accel (RPM/s):"() -> (w600:dbl)
            n258 = local read "Sample #:"() -> (w592:dbl)
            n259 = local read "# Drops*:"() -> (w610:dbl)
            n260 = local read "Ramp (s):"() -> (w618:dbl)
            n261 = local read "New: STS"() -> (w594:dbl)
            n262 = local read "Rec: Solvent"() -> (w569:string)
            n263 = local read "New: VT-Sat"() -> (w596:dbl)
            n264 = local read "Rec: On/Off"() -> (w598:dbl)
            n265 = local read "Rec: Method"() -> (w593:string)
            n266 = local read "Time (s):"() -> (w605:dbl)
            n267 = local read "Date Recorded"() -> (w589:string)
            n268 = local read "RPM:"() -> (w606:dbl)
            n269 = local read "Fabricator:"() -> (w614:string)
            n270 = Number To Decimal String(number=w555) -> (decimal integer string=w554:string)  [unwired: 1 in]
            n271 = Number To Decimal String(number=w610) -> (decimal integer string=w611:string)  [unwired: 1 in]
            n272 = Number To Decimal String(number=w592) -> (decimal integer string=w585:string)  [unwired: 1 in]
            n273 = call "DeviceID"("Sample"=w585, "Year"=w586, "Month"=w580, "Day"=w576, "Index"=w574) -> ("Result"=w591:string)  [unwired: 9 in, 1 out]
            n274 = Number To Decimal String(number=w573) -> (decimal integer string=w571:string)  [unwired: 1 in]
            n275 = Number To Decimal String(number=w572) -> (decimal integer string=w570:string)  [unwired: 1 in]
            n276 = Number To Decimal String(number=w609) -> (decimal integer string=w608:string)  [unwired: 1 in]
            n277 = Number To Decimal String(number=w565) -> (decimal integer string=w564:string)  [unwired: 1 in]
            n278 = Number To Decimal String(number=w613) -> (decimal integer string=w612:string)  [unwired: 1 in]
            n279 = Number To Decimal String(number=w568) -> (decimal integer string=w566:string)  [unwired: 1 in]
            n280 = Number To Decimal String(number=w606) -> (decimal integer string=w607:string)  [unwired: 1 in]
            n281 = Number To Fractional String(number=w600) -> (F-format string=w601:string)  [unwired: 3 in]
            n282 = Number To Decimal String(number=w605) -> (decimal integer string=w604:string)  [unwired: 1 in]
            n283 = Number To Fractional String(number=w602) -> (F-format string=w603:string)  [unwired: 3 in]
            n284 = Number To Fractional String(number=w598) -> (F-format string=w599:string)  [unwired: 3 in]
            n285 = Number To Fractional String(number=w596) -> (F-format string=w597:string)  [unwired: 3 in]
            n286 = Number To Fractional String(number=w594) -> (F-format string=w595:string)  [unwired: 3 in]
            n287 = Number To Decimal String(number=w618) -> (decimal integer string=w619:string)  [unwired: 1 in]
            n288 = Build Array(w591, w614, w593, w589, w585, w615, w616, w571, w570, w563, w567, w566, w569, w554, w608, w611, w621, w612, w564, w619, w607, w601, w604, w603, w599, w597, w595) -> (w617:string[])
            n289 = local write "Current \nRecord"(w617) -> ()
          }
          frame Enabled {
          }
        }
        n290 = local read "Lin-Vg Array-Used"() -> (w471:dbl[])
        n291 = local read "Sat Id-Log-Used"() -> (w475:dbl[])
        n292 = local read "New: Dielectric"() -> (w468:dbl)
        n293 = local read "Vg Array-Log-Used"() -> (w474:dbl[])
        n294 = local read "New: Length"() -> (w470:dbl)
        n295 = local read "New: Width"() -> (w467:dbl)
        n296 = local read "Lin Id-Used"() -> (w472:dbl[])
        n297 = local read "New: Dielectric"() -> (w464:dbl)
        n298 = local read "Lin Vd"() -> (w466:dbl)
        n299 = local read "Sat Vg Array-Used"() -> (w477:dbl[])
        n300 = local read "New: Dielectric"() -> (w462:dbl)
        n301 = local read "New: Length"() -> (w478:dbl)
        n302 = local read "New: Width"() -> (w480:dbl)
        n303 = local read "Sat Id-Used"() -> (w476:dbl[])
        n304 = call "Mobility-Vt-Used Pts_Linear.vi"("Width"=w467, "Length"=w470, "Vd"=w466, "Dielectric (d)"=w468, "Id Used"=w472, "Vg Used"=w471) -> ("Vt"=w473:dbl, "Mobility"=w469:dbl)  [unwired: 3 in, 1 out]
        n305 = call "STS-Used.vi"("Id Used"=w475, "Vg-Used"=w474) -> ("STS"=w465:dbl)  [unwired: 9 in]
        n306 = local write "New: Mobility-Lin"(w469) -> ()
        n307 = local write "New: VT-Lin"(w473) -> ()
        n308 = call "Mobility-Vt-Used Pts_Saturation.vi"("Width"=w480, "Length"=w478, "Dielectric (d)"=w462, "Sat Id Used"=w476, "Vg Used"=w477) -> ("Vt"=w463:dbl, "Mobility"=w479:dbl)  [unwired: 4 in, 1 out]
        n309 = local write "New: STS"(w465) -> ()
        n310 = local write "New: Mobility-Sat"(w479) -> ()
        n311 = local write "New: VT-Sat"(w463) -> ()
        n312 = call "Trap Density_VT.vi"("VT"=w463, "Dielectric"=w462) -> ("Trap Density-VT"=w461:dbl)
        n313 = local read "Manual-Temp"() -> (w458:bool)
        n314 = local read "Rec: Temp"() -> (w459:dbl)
        n315 = local write "New: Trap Density-VT"(w461) -> ()
        n316 = case shown="False" w458 {
          tunnel: w459 -> [w639 _]
          tunnel: [w636 w643] -> w457
          frame False {
            n317 = local read "Rec: Temp"() -> (w637:dbl)
            n318 = property on="New: Temp" class="DigNum (strict)"("DisabledEnum"=1) -> ()  [unwired: 2 in, 2 out]
            n319 = Equal To 0?(x=w637) -> (x = 0?=w638:bool)
            n320 = local write "New: Temp"(w639) -> ()
            n321 = case shown="True" w638 {
              tunnel: [w640 w641] -> w636
              tunnel: w637 -> [w640 _]
              frame False {
              }
              frame True {
                n322 = local read "Room Temp"() -> (w641:dbl)
              }
            }
            n323 = local write "New: Temp"(w636) -> ()
          }
          frame True {
            n324 = property on="New: Temp" class="DigNum (strict)"("DisabledEnum"=0) -> ()  [unwired: 2 in, 2 out]
            n325 = local read "New: Temp"() -> (w643:dbl)
          }
        }
        n326 = call "Trap Density_STS.vi"("Temp (T) [K]"=w457, "S.T.S. (S)"=w465, "Dielectric"=w464) -> ("Trap Density (N)"=w460:dbl)  [unwired: 8 in]
        n327 = local write "New: Trap Density-STS"(w460) -> ()
        n328 = property on="Image Out" class="ImageControl"() -> ("ZoomSingle"=w521:cluster{"X":sgl, "Y":sgl})  [unwired: 2 in, 2 out]
        n329 = property on="Image Out" class="ImageControl"() -> ("Bounds"=w522:T15)  [unwired: 2 in, 2 out]
        n330 = call <vilib>:"Intialize Keyboard.vi"() -> ("device ID"=w533:refnum<k1>)  [unwired: 10 in, 1 out]
        n331 = property on="Image Out" class="ImageControl"() -> ("Image Center Position"=w528:cluster{"X":u32, "Y":u32})  [unwired: 2 in, 2 out]
        n332 = call-poly <vilib>:"Acquire Input Data.vi"("device ID"=w533) -> ("keys pressed"=w532:T16)  [unwired: 16 in, 2 out]
        n333 = Unbundle(w522) -> ("Width"=w519:u32, "Height"=w518:u32)
        n334 = Unbundle(w521) -> ("X"=w496:sgl, "Y"=w520:sgl)
        n335 = Index Array(array=w532) -> (element=w536:T17)  [unwired: 1 in]
        n336 = event shown="[1] \"Undo Button\": Mouse Down" {
          selector: _ -> [_ _ _ _ _ _ _]
          dyn-events: _ -> [_ _ _ _ _ _ _]
          timeout: 10 -> [_ _ _ _ _ _ _]
          event "Remove Button": Mouse Down {
            w656 = 0
            n337 = event-data() -> ()  [unwired: 1 in, 7 out]
            n338 = property on="Image Out" class="ImageControl"() -> ("ROI"=w654:T14)  [unwired: 2 in, 2 out]
            n339 = Unbundle(w654) -> ("Global Rectangle"=w657:i32[], "Contours"=w659:T18)
            n340 = Reverse 1D Array(array=w657) -> (reversed array=w658:i32[])
            n341 = Reverse 1D Array(array=w659) -> (reversed array=w660:T18)
            n342 = Delete From Array(array=w658, index=w656) -> (array with subset deleted=w661:i32[])  [unwired: 1 in, 1 out]
            n343 = Delete From Array(array=w660, index=w656) -> (array with subset deleted=w662:T18)  [unwired: 1 in, 1 out]
            n344 = Reverse 1D Array(array=w661) -> (reversed array=w663:i32[])
            n345 = Reverse 1D Array(array=w662) -> (reversed array=w664:T18)
            n346 = Bundle(w663, w664) -> (w655:T19)  [unwired: 1 in]
            n347 = local write "ROI Descriptor out"(w654) -> ()
            n348 = local write "ROI Descriptor"(w655) -> ()
            n349 = property on="Image Out" class="ImageControl"("ROI"=w655) -> ()  [unwired: 2 in, 2 out]
          }
          event "Undo Button": Mouse Down {
            n350 = event-data() -> ()  [unwired: 1 in, 7 out]
            n351 = invoke on="Image Out" class="ImageControl" method="Clear ROI"() -> ()  [unwired: 3 in, 3 out]
          }
          event "Image Folder": Value Change {
            n352 = event-data() -> ()  [unwired: 1 in, 5 out]
            n353 = local read "Image File"() -> (w666:path)
            n354 = call "Vision Acquisition"("Image Path"=w666) -> ("Image Out"=w665:T2)  [unwired: 25 in, 1 out]
            n355 = local write "Image Out 2"(w665) -> ()
            n356 = local write "Image Out"(w665) -> ()
            n357 = invoke on="Image Out" class="ImageControl" method="Clear ROI"() -> ()  [unwired: 3 in, 3 out]
          }
          event "Zoom": Value Change {
            n358 = event-data() -> ()  [unwired: 1 in, 5 out]
            n359 = local read "Zoom"() -> (w667:i16)
            n360 = Bundle("Zoom"=w667, "Zoom"=w667) -> (w668:cluster{"Zoom":i16, "Zoom":i16})  [unwired: 1 in]
            n361 = property on="Image Out" class="ImageControl"("ZoomInteger"=w668) -> ()  [unwired: 2 in, 2 out]
          }
          event Timeout {
            n362 = event-data() -> ()  [unwired: 1 in, 2 out]
          }
          event "Image Out": Mouse Enter {
            (unwired) 6
            n363 = event-data() -> ()  [unwired: 1 in, 3 out]
            n364 = call "Simulate_Keyboard.vi"("Action"=0, "Virtual Key"=162) -> ()  [unwired: 7 in, 1 out]
          }
          event "Image Out": Mouse Leave {
            n365 = event-data() -> ()  [unwired: 1 in, 3 out]
            n366 = flat-sequence {
              frame #0 {
                n367 = Wait (ms)(milliseconds to wait=10) -> ()  [unwired: 1 out]
              }
              frame #1 {
                (unwired) 6
                n368 = call "Simulate_Keyboard.vi"("Action"=2, "Virtual Key"=162) -> ()  [unwired: 7 in, 1 out]
              }
            }
          }
        }
        n369 = Divide(x=w519, y=w496) -> (x/y=w509:sgl)
        n370 = Multiply(x=w509, y=0.5) -> (x*y=w515:dbl)
        n371 = Divide(x=w518, y=w520) -> (x/y=w508:sgl)
        n372 = Multiply(x=w508, y=0.5) -> (x*y=w514:dbl)
        n373 = Unbundle(w528) -> ("X"=w510:u32, "Y"=w511:u32)
        n374 = Subtract(x=w511, y=w514) -> (x-y=w512:dbl)
        n375 = Subtract(x=w510, y=w515) -> (x-y=w513:dbl)
        n376 = Add(x=w513, y=w509) -> (x+y=w527:dbl)
        n377 = Add(x=w512, y=w508) -> (x+y=w526:dbl)
        n378 = Reciprocal(x=w496) -> (1/x=w495:sgl)
        n379 = event shown="[2] \" Transfer File\": Value Change" {
          selector: _ -> [_ _ _ _ _ _ _ _ _ _ _ _ _ _ _ _]
          dyn-events: _ -> [_ _ _ _ _ _ _ _ _ _ _ _ _ _ _ _]
          timeout: 10 -> [_ _ _ _ _ _ _ _ _ _ _ _ _ _ _ _]
          tunnel: [_ _ _ _ _ _ _ _ _ _ _ _ _ TRUE _ TRUE] -> w553
          event Timeout {
            n380 = event-data() -> ()  [unwired: 1 in, 2 out]
          }
          event "Down Button": Mouse Down {
            w958 = "\\"
            w959 = "TSP"
            w1076 = 0
            # "Transpose"
            n381 = event-data() -> ()  [unwired: 1 in, 7 out]
            n382 = local read "Transfer File"() -> (w1080:path)
            n383 = Strip Path(path=w1080) -> (stripped path=w949:path, name=w1088:string)
            n384 = local write "Transfer Folder"(w949) -> ()
            n385 = property on="Image Out" class="ImageControl"() -> (error out=w1033:errorcluster, "Image Center Position"=w1037:cluster{"X":u32, "Y":u32})  [unwired: 2 in, 1 out]
            n386 = Strip Path(path=w949) -> (stripped path=w954:path)  [unwired: 1 out]
            n387 = List Folder(path=w949) -> (filenames=w1085:string[], error out=w1030:errorcluster)  [unwired: 3 in, 2 out]
            n388 = Path To String(path=w954) -> (string=w957:string)
            n389 = invoke on="Image Out" class="ImageControl" method="Clear ROI"() -> ()  [unwired: 3 in, 3 out]
            n390 = local read "Folder Index"() -> (w1032:dbl)
            n391 = Array Size(array=w1085) -> (size(s)=w1081:i32)
            n392 = Search 1D Array(1D array=w1085, element=w1088) -> (index of element=w1082:i32)  [unwired: 1 in]
            n393 = Unbundle(w1037) -> ("X"=w1035:u32)  [unwired: 1 out]
            n394 = Decrement(x=w1081) -> (x-1=w1083:i32)
            n395 = Equal?(x=w1082, y=w1083) -> (x = y?=w1084:bool)
            n396 = local read "Folder Index"() -> (w972:dbl)
            n397 = case shown="False" w1084 {
              tunnel: w1032 -> [w1252 _]
              tunnel: [w1251 0] -> w1031
              tunnel: w1030 -> [w1250 w1253]
              tunnel: [w1250 w1253] -> w1029
              frame False {
                n398 = Increment(x=w1252) -> (x+1=w1251:dbl)
              }
              frame True {
              }
            }
            n399 = local write "Folder Index"(w1031) -> ()
            n400 = Bundle("X"=w1035, 0) -> (w1036:cluster{"X":u32, i32})  [unwired: 1 in]
            n401 = property on="Image Out" class="ImageControl"(error in=w1033, "Image Center Position"=w1036) -> ()  [unwired: 1 in, 2 out]
            n402 = Path To String(path=w949) -> (string=w1089:string)
            n403 = Index Array(array=w1085, index=w1031) -> (element=w950:string)
            n404 = String Subset(string=w950, offset (0)=3) -> (substring=w953:string)  [unwired: 1 in]
            n405 = Concatenate Strings(w959, w953) -> (w955:string)
            n406 = Concatenate Strings(w957, w958, w959, w958, w955) -> (w956:string)
            n407 = String To Path(string=w956) -> (path=w951:path)
            n408 = local write "Transport File"(w951) -> ()
            n409 = Strip Path(path=w951) -> (stripped path=w971:path, name=w962:string)
            n410 = local write "Transport Folder"(w971) -> ()
            n411 = List Folder(path=w971) -> (filenames=w966:string[], error out=w974:errorcluster)  [unwired: 3 in, 2 out]
            n412 = Array Size(array=w966) -> (size(s)=w970:i32)
            n413 = Search 1D Array(1D array=w966, element=w962) -> (index of element=w969:i32)  [unwired: 1 in]
            n414 = Decrement(x=w970) -> (x-1=w968:i32)
            n415 = Equal?(x=w969, y=w968) -> (x = y?=w967:bool)
            n416 = case shown="False" w967 {
              tunnel: w972 -> [w1114 _]
              tunnel: [w1113 0] -> w973
              tunnel: w974 -> [w1112 w1115]
              tunnel: [w1112 w1115] -> _
              frame False {
                n417 = Increment(x=w1114) -> (x+1=w1113:dbl)
              }
              frame True {
              }
            }
            n418 = local write "Folder Index"(w973) -> ()
            n419 = local write "Data Name:"(w950) -> ()
            n420 = Path To String(path=w971) -> (string=w961:string)
            n421 = Index Array(array=w966, index=w973) -> (element=w965:string)
            n422 = local write "Data Name:"(w965) -> ()
            n423 = Concatenate Strings(w1089, "\\", w950) -> (w1087:string)
            n424 = Concatenate Strings(w961, "\\", w965) -> (w963:string)
            n425 = String To Path(string=w1087) -> (path=w1007:path)
            n426 = call "Recorded Values.vi"("Path"=w1007) -> ("Recorded Char"=w1091:T6, "Recorded Prop"=w1092:T7, "Fabrication Prop"=w1090:T8)  [unwired: 8 in]
            n427 = Unbundle By Name(w1091) -> ("Mobility-Sat"=w1104:dbl, "Moblitity-Lin"=w1105:dbl, "On/Off"=w1106:dbl, "Off Current"=w1107:dbl, "Vt-Sat"=w1002:dbl, "STS"=w1108:dbl, "Trap Density-VT"=w1109:dbl, "Trap Density-STS"=w1110:dbl)
            n428 = Unbundle By Name(w1090) -> ("Date Created"=w1111:string, "Material"=w1093:string, "Solvent"=w1094:string, "Concentration"=w1095:dbl, "Method"=w1096:string, "Dielectric (nm)"=w1097:dbl, "Treatment"=w1098:string, "Comments"=w1099:string)
            n429 = Unbundle By Name(w1092) -> ("Date Recorded"=w1100:string, "Index"=w1101:string, "Length"=w1102:dbl, "Width"=w1103:dbl, "Sample Temp"=w1004:dbl)
            n430 = local write "Date Created"(w1111) -> ()
            n431 = local write "Rec: Off I-Sat"(w1107) -> ()
            n432 = local write "Rec: Comments"(w1099) -> ()
            n433 = local write "Rec: Material"(w1093) -> ()
            n434 = local write "Rec: VT-Sat"(w1002) -> ()
            n435 = local write "Rec: Concentration"(w1095) -> ()
            n436 = local write "Rec: Method"(w1096) -> ()
            n437 = local write "Rec: Dielectric (d)"(w1097) -> ()
            n438 = local write "Surface Treatment:"(w1098) -> ()
            n439 = local write "Index"(w1101) -> ()
            n440 = local write "Rec: Mobility-Sat"(w1104) -> ()
            n441 = local write "Rec: Mobility-Lin"(w1105) -> ()
            n442 = local write "Rec: On/Off"(w1106) -> ()
            n443 = local write "Rec: STS"(w1108) -> ()
            n444 = local write "Rec: Trap Density-VT"(w1109) -> ()
            n445 = local write "Rec: Trap Density-STS"(w1110) -> ()
            n446 = local write "Rec: Solvent"(w1094) -> ()
            n447 = local write "Date Recorded"(w1100) -> ()
            n448 = local write "Rec: Length"(w1102) -> ()
            n449 = local write "Rec: Width"(w1103) -> ()
            n450 = local write "Rec: Temp"(w1004) -> ()
            n451 = Equal To 0?(x=w1004) -> (x = 0?=w1005:bool)
            n452 = case shown="True" w1005 {
              tunnel: [w1123 w1124] -> w1003
              tunnel: w1004 -> [w1123 _]
              frame False {
              }
              frame True {
                n453 = local read "Room Temp"() -> (w1124:dbl)
              }
            }
            n454 = String To Path(string=w963) -> (path=w960:path)
            n455 = local read "NumPoints Log"() -> (w1026:dbl)
            n456 = local write "Transfer File"(w1007) -> ()
            n457 = local read "Num Pts"() -> (w1028:dbl)
            n458 = Strip Path(path=w960) -> ()  [unwired: 2 out]
            n459 = call-poly <vilib>:"Read From Spreadsheet File.vi"("file path (dialog if empty)"=w960) -> ("all rows"=w988:string[][])  [unwired: 6 in, 4 out]
            n460 = Array Size(array=w988) -> (size(s)=w994:i32[])
            n461 = call-poly <vilib>:"Read From Spreadsheet File.vi"("file path (dialog if empty)"=w1007) -> ("all rows"=w932:string[][])  [unwired: 6 in, 4 out]
            n462 = call "Mobility-Vt Calculator-File.vi"("NumPts"=w1028, "Path"=w1007) -> ("Used Points"=w928:T10, "Graph Cluster"=w1000:T11, "Output"=w1027:T12)  [unwired: 6 in, 1 out]
            n463 = Unbundle By Name(w928) -> ("Index-Lin"=w926:dbl, "Index-Sat"=w927:dbl)
            n464 = local read "New: Dielectric"() -> (w1012:dbl)
            n465 = call "STS Calculator-File.vi"("NumPts"=w1026, "Path"=w1007) -> ("Used Points"=w925:T9, "XY Graph-Sat"=w1025:cluster{dbl[], dbl[]}[], "Ouput"=w1024:cluster{"STS-Sat":dbl, "STS-Lin":dbl})  [unwired: 6 in, 1 out]
            n466 = Unbundle By Name(w925) -> ("STS Index-Sat"=w924:dbl)
            n467 = local write "Index 2"(w924) -> ()
            n468 = Array Subset(array=w988, length (col)=1) -> (w990:string[][])  [unwired: 3 in]
            n469 = Index Array(array=w994, index=0) -> (element=w983:i32)
            n470 = local write "Sat-Trans Slider"(w927) -> ()
            n471 = Array Size(array=w932) -> (size(s)=w1077:i32[])
            n472 = Unbundle By Name(w1027) -> ("Mobility-Sat"=w1023:dbl, "Vt-Sat"=w1011:dbl, "Mobility-Lin"=w1022:dbl, "Vt-Lin"=w1021:dbl, "Off I-Sat"=w1008:dbl, "On/Off I-Sat"=w1001:dbl)
            n473 = Unbundle By Name(w1024) -> ("STS-Sat"=w1006:dbl)  [unwired: 1 out]
            n474 = Reshape Array(w990, w983) -> (w989:string[])
            n475 = local write "MobVi Index"(w927) -> ()
            n476 = local write "Sat-Log"(w1025) -> ()
            n477 = Search 1D Array(1D array=w989, element="Vd") -> (index of element=w987:i32)  [unwired: 1 in]
            n478 = Unbundle By Name(w1000) -> ("Raw Sat"=w997:cluster{dbl[], dbl[]}[], "Sqrt Sat"=w999:cluster{dbl[], dbl[]}[], "Raw Lin"=w996:cluster{dbl[], dbl[]}[], "Sqrt Lin"=w998:cluster{dbl[], dbl[]}[], "Log Lin"=w995:cluster{dbl[], dbl[]}[])  [unwired: 1 out]
            n479 = local write "Sqrt-Sat"(w999) -> ()
            n480 = call "Trap Density_VT.vi"("VT"=w1011, "Dielectric"=w1012) -> ("Trap Density-VT"=w1010:dbl)
            n481 = Index Array(array=w1077, index=0) -> (element=w1061:i32)
            n482 = call "Trap Density_STS.vi"("Temp (T) [K]"=w1003, "S.T.S. (S)"=w1006, "Dielectric"=w1012) -> ("Trap Density (N)"=w1009:dbl)  [unwired: 8 in]
            n483 = local write "New: STS"(w1006) -> ()
            n484 = local write "Calc: STS"(w1006) -> ()
            n485 = Increment(x=w987) -> (x+1=w986:i32)
            n486 = Array Subset(array=w988, index (row)=w986) -> (w984:string[][])  [unwired: 3 in]
            n487 = Fract/Exp String To Number(string=w984, default (0 dbl)="default (0 dbl) 3") -> (number=w976:ext[][])  [unwired: 2 in, 1 out]
            n488 = local write "Calc: Mobility-Sat"(w1023) -> ()
            n489 = local write "Calc: Off I-Sat"(w1021) -> ()
            n490 = local write "Calc: Mobility-Lin"(w1022) -> ()
            n491 = Decimate 1D Array(w1025) -> (w1056:cluster{dbl[], dbl[]}[])  [unwired: 1 out]
            n492 = Decimate 1D Array(w999) -> (w1064:cluster{dbl[], dbl[]}[])  [unwired: 1 out]
            n493 = local write "Calc: Off I-Sat"(w1008) -> ()
            n494 = local write "Calc: On/Off"(w1001) -> ()
            n495 = Decimate 1D Array(w998) -> (w1020:cluster{dbl[], dbl[]}[])  [unwired: 1 out]
            n496 = local write "Calc: VT-Sat"(w1011) -> ()
            n497 = Array Subset(array=w932, index (row)=w1076, index (col)=w1076, length (col)=3) -> (w1078:string[][])  [unwired: 1 in]
            n498 = Delete From Array(array=w976) -> (array with subset deleted=w975:ext[][])  [unwired: 3 in, 1 out]
            n499 = local write "Calc: Trap Density-VT"(w1010) -> ()
            n500 = local write "Calc: Trap Density-STS"(w1009) -> ()
            n501 = local write "New: Trap Density-STS"(w1009) -> ()
            n502 = local write "New: Trap Density-VT"(w1010) -> ()
            n503 = Array To Cluster(array=w1056) -> (cluster=w1054:T13)
            n504 = Array To Cluster(array=w1064) -> (cluster=w1066:T13)
            n505 = local write "Raw- Sat"(w997) -> ()
            n506 = local write "Sqrt-Lin"(w998) -> ()
            n507 = Delete From Array(array=w975, index (col)=0 ("Deaktivierter Index (Spalte)")) -> (deleted portion=w980:ext[], array with subset deleted=w981:ext[][])  [unwired: 2 in]
            n508 = local write "Raw- Lin"(w996) -> ()
            n509 = local write "New: VT-Lin"(w1021) -> ()
            n510 = local write "Log-Lin"(w995) -> ()
            n511 = local write "New: VT-Sat"(w1011) -> ()
            n512 = local write "New: Mobility-Sat"(w1023) -> ()
            n513 = Transpose 2D Array(2D array=w981) -> (transposed array=w982:ext[][])
            n514 = local write "New: Mobility-Lin"(w1022) -> ()
            n515 = Reshape Array(w1078, w1061) -> (w934:string[])
            n516 = Search 1D Array(1D array=w934, element="Vg") -> (index of element=w938:i32)  [unwired: 1 in]
            n517 = Add(x=w938, y=3) -> (x+y=w936:i32)
            n518 = Divide(x=w936, y=3) -> (x/y=w943:dbl)
            n519 = Array Subset(array=w932, index (row)=w943, index (col)=0, length (col)=1) -> (w942:string[][])  [unwired: 1 in]
            n520 = Fract/Exp String To Number(string=w942) -> (number=w946:dbl[][])  [unwired: 3 in, 1 out]
            n521 = Array Size(array=w946) -> (size(s)=w933:i32[])
            n522 = Index Array(array=w933, index=0) -> (element=w944:i32)
            n523 = Decrement(x=w944) -> (x-1=w947:i32)
            n524 = Reshape Array(w946, w947) -> (w931:dbl[])
            n525 = local write "Data Length"(w947) -> ()
            n526 = local write "Vg Column"(w931) -> ()
            n527 = Array To Cluster(array=w1020) -> (cluster=w1019:T13)
            n528 = for {
              tunnel: w980 -> [w1121]
              tunnel: w982 -> [w1122] mode=indexing
              tunnel: [w1120] -> w978 mode=indexing
              n529 = Bundle(w1121, w1122) -> (w1120:cluster{ext[], ext[]})  [unwired: 1 in]
            }
            n530 = Array Max & Min(array=w931) -> (max value=w930:dbl, min value=w929:dbl)  [unwired: 2 out]
            n531 = Unbundle(w1054) -> ("[0]"=w1055:cluster{dbl[], dbl[]})  [unwired: 8 out]
            n532 = Unbundle(w1066) -> ("[0]"=w1065:cluster{dbl[], dbl[]})  [unwired: 8 out]
            n533 = Unbundle(w1019) -> ("[0]"=w1016:cluster{dbl[], dbl[]})  [unwired: 8 out]
            n534 = Search 1D Array(1D array=w934, element="Index:") -> (index of element=w1073:i32)  [unwired: 1 in]
            n535 = local write "Transport"(w978) -> ()
            n536 = property on="Sat-Trans Slider" class="Slide (strict)"("Scale.Maximum"=w930, "Scale.Minimum"=w929) -> ()  [unwired: 2 in, 2 out]
            n537 = Array Size(array=w978) -> (size(s)=w977:i32)
            n538 = local read "Num Pts"() -> (w1015:dbl)
            n539 = Unbundle(w1016) -> (w1018:dbl[], w1017:dbl[])
            n540 = for {
              N: w977 -> [_]
              i -> [w1119]
              n541 = local read "Transport Line Color"() -> (w1118:u32)
              n542 = local read "Ring"() -> (w1117:u16)
              n543 = property on="Transport" class="XYGraph (strict)"("Active Plot"=w1119, "Plot.Plot Color"=w1118, "Plot.Line Width"=w1117) -> ()  [unwired: 2 in, 2 out]
            }
            n544 = Increment(x=w1073) -> (x+1=w1074:i32)
            n545 = Unbundle(w1055) -> (w1053:dbl[], w1052:dbl[])
            n546 = Unbundle(w1065) -> (w1058:dbl[], w1057:dbl[])
            n547 = Array Subset(array=w1018, index=w926, length=w1015) -> (w1014:dbl[])
            n548 = Array Subset(array=w1017, index=w926, length=w1015) -> (w1013:dbl[])
            n549 = Array Subset(array=w1053, index=w924, length=w1026) -> (w1060:dbl[])
            n550 = Array Subset(array=w1052, index=w924, length=w1026) -> (w1059:dbl[])
            n551 = Array Subset(array=w1058, index=w927, length=w1028) -> (w1063:dbl[])
            n552 = Array Subset(array=w1057, index=w927, length=w1028) -> (w1062:dbl[])
            n553 = Index Array(array=w934, index=w1074) -> (element=w1041:string)
            n554 = local write "Lin-Vg Array-Used"(w1014) -> ()
            n555 = local write "Sat Vg Array-Used"(w1063) -> ()
            n556 = local write "Vg Array-Log-Used"(w1059) -> ()
            n557 = local write "Lin Id-Used"(w1013) -> ()
            n558 = local read "Image Folder"() -> (w1039:path)
            n559 = local write "Sat Id-Used"(w1062) -> ()
            n560 = local write "Sat Id-Log-Used"(w1060) -> ()
            n561 = List Folder(path=w1039, error in=w1029) -> (filenames=w1072:string[], error out=w1042:errorcluster)  [unwired: 2 in, 2 out]
            n562 = while {
              tunnel: w1072 -> [w1137]
              tunnel: w1041 -> [w1135]
              tunnel: [w1134] -> _
              tunnel: [w1134] -> w1071
              tunnel: w1061 -> [w1133]
              i -> [w1134]
              stop <- w1130 stop-if-true
              n563 = Index Array(array=w1137, index=w1134) -> (element=w1138:string)
              n564 = xnode "Match Regular Expression"("input string"=w1138, "regular expression"=w1135) -> ("whole match"=w1136:string)  [unwired: 4 in, 4 out]
              n565 = Equal?(x=w1136, y=w1135) -> (x = y?=w1132:bool)
              n566 = Equal?(x=w1133, y=w1134) -> (x = y?=w1131:bool)
              n567 = Or(x=w1132, y=w1131) -> (x .or. y?=w1130:bool)
            }
            n568 = Build Path(base path=w1039, name or relative path="ROI") -> (appended path=w1038:path)
            n569 = Path To String(path=w1039) -> (string=w1069:string)
            n570 = Index Array(array=w1072, index=w1071) -> (element=w1050:string)
            n571 = invoke on="Image Out" class="ImageControl" method="Clear ROI"(error in=w1042) -> (error out=w1045:errorcluster)  [unwired: 2 in, 2 out]
            n572 = local write "Image Name"(w1050) -> ()
            n573 = Build Path(base path=w1038, name or relative path=w1041) -> (appended path=w1046:path)
            n574 = call <vilib>:"Check if File or Folder Exists.vi"("error in (no error)"=w1045, "path"=w1046) -> ("file or folder exists?"=w1043:bool, "dup path"=w1044:path)  [unwired: 7 in, 1 out]
            n575 = Concatenate Strings(w1069, "\\", w1050) -> (w1068:string)
            n576 = case shown="False" w1043 {
              tunnel: w1044 -> [_ w1125]
              frame False {
              }
              frame True {
                n577 = Read from Text File(file (use dialog)=w1125) -> (text=w1129:string)  [unwired: 3 in, 3 out]
                n578 = property on="Image Out" class="ImageControl"() -> ("ROI"=w1126:T14)  [unwired: 2 in, 2 out]
                n579 = Unflatten From String(type=w1126, binary string=w1129) -> (value=w1127:T14, error out=w1128:errorcluster)  [unwired: 3 in, 1 out]
                n580 = property on="Image Out" class="ImageControl"(error in=w1128, "ROI"=w1127) -> ()  [unwired: 1 in, 2 out]
              }
            }
            n581 = String To Path(string=w1068) -> (path=w1049:path)
            n582 = Empty String/Path?(string/path=w1050) -> (empty?=w1051:bool)
            n583 = local read "No Image File"() -> (w1047:path)
            n584 = Select(t=w1047, s=w1051, f=w1049) -> (s? t:f=w1048:path)
            n585 = local write "Image File"(w1048) -> ()
            n586 = call "Vision Acquisition4"("Image Path"=w1048) -> ("Image Out"=w1070:T2)  [unwired: 25 in, 1 out]
            n587 = local write "Image Out"(w1070) -> ()
            n588 = local write "Image Out 2"(w1070) -> ()
          }
          event "Transfer File": Value Change {
            w1282 = 0
            w1296 = "\\"
            w1297 = "TSP"
            w1429 = 0
            # "Transpose"
            n589 = event-data() -> ()  [unwired: 1 in, 5 out]
            n590 = local read "Transfer File"() -> (w1425:path)
            n591 = Strip Path(path=w1425) -> (stripped path=w1287:path, name=w1437:string)
            n592 = local write "Transfer Folder"(w1287) -> ()
            n593 = property on="Image Out" class="ImageControl"() -> (error out=w1383:errorcluster, "Image Center Position"=w1387:cluster{"X":u32, "Y":u32})  [unwired: 2 in, 1 out]
            n594 = List Folder(path=w1287) -> (filenames=w1434:string[], error out=w1393:errorcluster)  [unwired: 3 in, 2 out]
            n595 = Strip Path(path=w1287) -> (stripped path=w1292:path)  [unwired: 1 out]
            n596 = Search 1D Array(1D array=w1434, element=w1437) -> (index of element=w1382:i32)  [unwired: 1 in]
            n597 = Path To String(path=w1292) -> (string=w1295:string)
            n598 = local write "Folder Index"(w1382) -> ()
            n599 = Unbundle(w1387) -> ("X"=w1385:u32)  [unwired: 1 out]
            n600 = Path To String(path=w1287) -> (string=w1438:string)
            n601 = Index Array(array=w1434, index=w1382) -> (element=w1288:string)
            n602 = String Subset(string=w1288, offset (0)=3) -> (substring=w1291:string)  [unwired: 1 in]
            n603 = Concatenate Strings(w1297, w1291) -> (w1293:string)
            n604 = Concatenate Strings(w1295, w1296, w1297, w1296, w1293) -> (w1294:string)
            n605 = Bundle("X"=w1385, 0) -> (w1386:cluster{"X":u32, i32})  [unwired: 1 in]
            n606 = String To Path(string=w1294) -> (path=w1289:path)
            n607 = local write "Transport File"(w1289) -> ()
            n608 = Strip Path(path=w1289) -> (stripped path=w1318:path, name=w1323:string)
            n609 = local write "Transport Folder"(w1318) -> ()
            n610 = local write "Data Name:"(w1288) -> ()
            n611 = property on="Image Out" class="ImageControl"(error in=w1383, "Image Center Position"=w1386) -> ()  [unwired: 1 in, 2 out]
            n612 = List Folder(path=w1318) -> (filenames=w1319:string[])  [unwired: 3 in, 3 out]
            n613 = Search 1D Array(1D array=w1319, element=w1323) -> (index of element=w1286:i32)  [unwired: 1 in]
            n614 = Concatenate Strings(w1438, "\\", w1288) -> (w1436:string)
            n615 = String To Path(string=w1436) -> (path=w1260:path)
            n616 = call "Recorded Values.vi"("Path"=w1260) -> ("Recorded Char"=w1380:T6, "Recorded Prop"=w1379:T7, "Fabrication Prop"=w1381:T8)  [unwired: 8 in]
            n617 = Unbundle By Name(w1380) -> ("Mobility-Sat"=w1367:dbl, "Moblitity-Lin"=w1366:dbl, "On/Off"=w1365:dbl, "Off Current"=w1364:dbl, "Vt-Sat"=w1334:dbl, "STS"=w1363:dbl, "Trap Density-VT"=w1362:dbl, "Trap Density-STS"=w1361:dbl)
            n618 = Unbundle By Name(w1381) -> ("Date Created"=w1360:string, "Material"=w1378:string, "Solvent"=w1377:string, "Concentration"=w1376:dbl, "Method"=w1375:string, "Dielectric (nm)"=w1374:dbl, "Treatment"=w1373:string, "Comments"=w1372:string)
            n619 = Unbundle By Name(w1379) -> ("Date Recorded"=w1371:string, "Index"=w1370:string, "Length"=w1369:dbl, "Width"=w1368:dbl, "Sample Temp"=w1336:dbl)
            n620 = local write "Date Created"(w1360) -> ()
            n621 = local write "Rec: Material"(w1378) -> ()
            n622 = local write "Rec: Off I-Sat"(w1364) -> ()
            n623 = local write "Rec: Comments"(w1372) -> ()
            n624 = local write "Rec: VT-Sat"(w1334) -> ()
            n625 = local write "Rec: Concentration"(w1376) -> ()
            n626 = local write "Rec: Method"(w1375) -> ()
            n627 = local write "Rec: Dielectric (d)"(w1374) -> ()
            n628 = local write "Surface Treatment:"(w1373) -> ()
            n629 = local write "Index"(w1370) -> ()
            n630 = local write "Rec: Mobility-Sat"(w1367) -> ()
            n631 = local write "Rec: Mobility-Lin"(w1366) -> ()
            n632 = local write "Rec: On/Off"(w1365) -> ()
            n633 = local write "Rec: STS"(w1363) -> ()
            n634 = local write "Rec: Trap Density-VT"(w1362) -> ()
            n635 = local write "Rec: Trap Density-STS"(w1361) -> ()
            n636 = local write "Rec: Solvent"(w1377) -> ()
            n637 = local write "Date Recorded"(w1371) -> ()
            n638 = local write "Rec: Length"(w1369) -> ()
            n639 = local write "Rec: Width"(w1368) -> ()
            n640 = local write "Rec: Temp"(w1336) -> ()
            n641 = Equal To 0?(x=w1336) -> (x = 0?=w1337:bool)
            n642 = case shown="True" w1337 {
              tunnel: [w1445 w1446] -> w1335
              tunnel: w1336 -> [w1445 _]
              frame False {
              }
              frame True {
                n643 = local read "Room Temp"() -> (w1446:dbl)
              }
            }
            n644 = local write "Folder Index"(w1286) -> ()
            n645 = local read "NumPoints Log"() -> (w1357:dbl)
            n646 = local write "Transfer File"(w1260) -> ()
            n647 = local read "Num Pts"() -> (w1358:dbl)
            n648 = Path To String(path=w1318) -> (string=w1324:string)
            n649 = call-poly <vilib>:"Read From Spreadsheet File.vi"("file path (dialog if empty)"=w1260) -> ("all rows"=w1431:string[][])  [unwired: 6 in, 4 out]
            n650 = Index Array(array=w1319, index=w1286) -> (element=w1320:string)
            n651 = local read "New: Dielectric"() -> (w1343:dbl)
            n652 = call "STS Calculator-File.vi"("NumPts"=w1357, "Path"=w1260) -> ("Used Points"=w1256:T9, "XY Graph-Sat"=w1356:cluster{dbl[], dbl[]}[], "Ouput"=w1355:cluster{"STS-Sat":dbl, "STS-Lin":dbl})  [unwired: 6 in, 1 out]
            n653 = Unbundle By Name(w1256) -> ("STS Index-Sat"=w1255:dbl)
            n654 = call "Mobility-Vt Calculator-File.vi"("NumPts"=w1358, "Path"=w1260) -> ("Used Points"=w1259:T10, "Graph Cluster"=w1331:T11, "Output"=w1359:T12)  [unwired: 6 in, 1 out]
            n655 = Unbundle By Name(w1259) -> ("Index-Lin"=w1258:dbl, "Index-Sat"=w1257:dbl)
            n656 = local write "Data Name:"(w1320) -> ()
            n657 = Unbundle By Name(w1359) -> ("Mobility-Sat"=w1345:dbl, "Vt-Sat"=w1339:dbl, "Mobility-Lin"=w1344:dbl, "Vt-Lin"=w1332:dbl, "Off I-Sat"=w1338:dbl, "On/Off I-Sat"=w1333:dbl)
            n658 = local write "Index 2"(w1255) -> ()
            n659 = Unbundle By Name(w1355) -> ("STS-Sat"=w1340:dbl)  [unwired: 1 out]
            n660 = local write "MobVi Index"(w1257) -> ()
            n661 = local write "Sat-Log"(w1356) -> ()
            n662 = Concatenate Strings(w1324, "\\", w1320) -> (w1322:string)
            n663 = local write "Sat-Trans Slider"(w1257) -> ()
            n664 = Array Size(array=w1431) -> (size(s)=w1430:i32[])
            n665 = call "Trap Density_VT.vi"("VT"=w1339, "Dielectric"=w1343) -> ("Trap Density-VT"=w1342:dbl)
            n666 = call "Trap Density_STS.vi"("Temp (T) [K]"=w1335, "S.T.S. (S)"=w1340, "Dielectric"=w1343) -> ("Trap Density (N)"=w1341:dbl)  [unwired: 8 in]
            n667 = String To Path(string=w1322) -> (path=w1325:path)
            n668 = local write "Calc: Mobility-Lin"(w1344) -> ()
            n669 = local write "Calc: Mobility-Sat"(w1345) -> ()
            n670 = local write "Calc: VT-Sat"(w1339) -> ()
            n671 = local write "Calc: Off I-Sat"(w1338) -> ()
            n672 = local write "Calc: VT-Lin"(w1332) -> ()
            n673 = local write "Calc: On/Off"(w1333) -> ()
            n674 = local write "Calc: STS"(w1340) -> ()
            n675 = Strip Path(path=w1325) -> ()  [unwired: 2 out]
            n676 = Unbundle By Name(w1331) -> ("Raw Sat"=w1328:cluster{dbl[], dbl[]}[], "Sqrt Sat"=w1329:cluster{dbl[], dbl[]}[], "Raw Lin"=w1327:cluster{dbl[], dbl[]}[], "Sqrt Lin"=w1330:cluster{dbl[], dbl[]}[], "Log Lin"=w1326:cluster{dbl[], dbl[]}[])  [unwired: 1 out]
            n677 = call-poly <vilib>:"Read From Spreadsheet File.vi"("file path (dialog if empty)"=w1325) -> ("all rows"=w1304:string[][])  [unwired: 6 in, 4 out]
            n678 = Decimate 1D Array(w1330) -> (w1354:cluster{dbl[], dbl[]}[])  [unwired: 1 out]
            n679 = local write "Calc: Trap Density-VT"(w1342) -> ()
            n680 = local write "Calc: Trap Density-STS"(w1341) -> ()
            n681 = local write "New: Trap Density-STS"(w1341) -> ()
            n682 = local write "New: Trap Density-VT"(w1342) -> ()
            n683 = local write "Sqrt-Lin"(w1330) -> ()
            n684 = Array Size(array=w1304) -> (size(s)=w1298:i32[])
            n685 = local write "New: VT-Sat"(w1339) -> ()
            n686 = Decimate 1D Array(w1356) -> (w1408:cluster{dbl[], dbl[]}[])  [unwired: 1 out]
            n687 = Index Array(array=w1430, index=w1429) -> (element=w1412:i32)
            n688 = Decimate 1D Array(w1329) -> (w1415:cluster{dbl[], dbl[]}[])  [unwired: 1 out]
            n689 = local write "Sqrt-Sat"(w1329) -> ()
            n690 = local write "New: Mobility-Lin"(w1344) -> ()
            n691 = Array Subset(array=w1431, index (row)=w1429, index (col)=w1429, length (col)=3) -> (w1432:string[][])  [unwired: 1 in]
            n692 = local write "New: VT-Lin"(w1332) -> ()
            n693 = Array To Cluster(array=w1354) -> (cluster=w1353:T13)
            n694 = local write "New: STS"(w1340) -> ()
            n695 = local write "New: Mobility-Sat"(w1345) -> ()
            n696 = Array Subset(array=w1304, length (col)=1) -> (w1302:string[][])  [unwired: 3 in]
            n697 = Index Array(array=w1298, index=0) -> (element=w1309:i32)
            n698 = Array To Cluster(array=w1408) -> (cluster=w1406:T13)
            n699 = Array To Cluster(array=w1415) -> (cluster=w1417:T13)
            n700 = Reshape Array(w1432, w1412) -> (w1418:string[])
            n701 = local write "Raw- Sat"(w1328) -> ()
            n702 = Unbundle(w1353) -> ("[0]"=w1352:cluster{dbl[], dbl[]})  [unwired: 8 out]
            n703 = Reshape Array(w1302, w1309) -> (w1303:string[])
            n704 = local write "Raw- Lin"(w1327) -> ()
            n705 = local read "Num Pts"() -> (w1349:dbl)
            n706 = local write "Log-Lin"(w1326) -> ()
            n707 = Unbundle(w1352) -> (w1351:dbl[], w1350:dbl[])
            n708 = Unbundle(w1406) -> ("[0]"=w1407:cluster{dbl[], dbl[]})  [unwired: 8 out]
            n709 = Unbundle(w1417) -> ("[0]"=w1416:cluster{dbl[], dbl[]})  [unwired: 8 out]
            n710 = Search 1D Array(1D array=w1303, element="Vd") -> (index of element=w1305:i32)  [unwired: 1 in]
            n711 = Search 1D Array(1D array=w1418, element="Index:") -> (index of element=w1426:i32)  [unwired: 1 in]
            n712 = local read "Num Pts"() -> (w1346:dbl)
            n713 = Increment(x=w1305) -> (x+1=w1306:i32)
            n714 = Array Subset(array=w1304, index (row)=w1306) -> (w1308:string[][])  [unwired: 3 in]
            n715 = Array Subset(array=w1351, index=w1258, length=w1349) -> (w1348:dbl[])
            n716 = Array Subset(array=w1350, index=w1258, length=w1349) -> (w1347:dbl[])
            n717 = Increment(x=w1426) -> (x+1=w1427:i32)
            n718 = Unbundle(w1407) -> (w1404:dbl[], w1403:dbl[])
            n719 = Unbundle(w1416) -> (w1405:dbl[], w1409:dbl[])
            n720 = Fract/Exp String To Number(string=w1308, default (0 dbl)="default (0 dbl) 5") -> (number=w1316:ext[][])  [unwired: 2 in, 1 out]
            n721 = Delete From Array(array=w1316) -> (array with subset deleted=w1317:ext[][])  [unwired: 3 in, 1 out]
            n722 = local read "Image Folder"() -> (w1389:path)
            n723 = Delete From Array(array=w1317, index (col)=0 ("Deaktivierter Index (Spalte)")) -> (deleted portion=w1312:ext[], array with subset deleted=w1311:ext[][])  [unwired: 2 in]
            n724 = local write "Lin-Vg Array-Used"(w1348) -> ()
            n725 = Array Subset(array=w1404, index=w1255, length=w1357) -> (w1411:dbl[])
            n726 = Array Subset(array=w1403, index=w1255, length=w1357) -> (w1410:dbl[])
            n727 = Array Subset(array=w1405, index=w1257, length=w1346) -> (w1414:dbl[])
            n728 = Array Subset(array=w1409, index=w1257, length=w1346) -> (w1413:dbl[])
            n729 = Index Array(array=w1418, index=w1427) -> (element=w1391:string)
            n730 = local write "Lin Id-Used"(w1347) -> ()
            n731 = Transpose 2D Array(2D array=w1311) -> (transposed array=w1310:ext[][])
            n732 = local write "Sat Vg Array-Used"(w1414) -> ()
            n733 = local write "Vg Array-Log-Used"(w1410) -> ()
            n734 = for {
              tunnel: w1312 -> [w1443]
              tunnel: w1310 -> [w1444] mode=indexing
              tunnel: [w1442] -> w1314 mode=indexing
              n735 = Bundle(w1443, w1444) -> (w1442:cluster{ext[], ext[]})  [unwired: 1 in]
            }
            n736 = local write "Sat Id-Log-Used"(w1411) -> ()
            n737 = local write "Sat Id-Used"(w1413) -> ()
            n738 = local write "Index"(w1391) -> ()
            n739 = List Folder(path=w1389, error in=w1393) -> (filenames=w1423:string[], error out=w1392:errorcluster)  [unwired: 2 in, 2 out]
            n740 = Build Path(base path=w1389, name or relative path="ROI") -> (appended path=w1388:path)
            n741 = local write "Transport"(w1314) -> ()
            n742 = Array Size(array=w1314) -> (size(s)=w1315:i32)
            n743 = invoke on="Image Out" class="ImageControl" method="Clear ROI"(error in=w1392) -> (error out=w1396:errorcluster)  [unwired: 2 in, 2 out]
            n744 = Build Path(base path=w1388, name or relative path=w1391) -> (appended path=w1397:path)
            n745 = while {
              tunnel: w1423 -> [w1459]
              tunnel: w1391 -> [w1457]
              tunnel: [w1456] -> _
              tunnel: [w1456] -> w1422
              tunnel: w1412 -> [w1455]
              i -> [w1456]
              stop <- w1452 stop-if-true
              n746 = Index Array(array=w1459, index=w1456) -> (element=w1460:string)
              n747 = xnode "Match Regular Expression"("input string"=w1460, "regular expression"=w1457) -> ("whole match"=w1458:string)  [unwired: 4 in, 4 out]
              n748 = Equal?(x=w1458, y=w1457) -> (x = y?=w1454:bool)
              n749 = Equal?(x=w1455, y=w1456) -> (x = y?=w1453:bool)
              n750 = Or(x=w1454, y=w1453) -> (x .or. y?=w1452:bool)
            }
            n751 = for {
              N: w1315 -> [_]
              i -> [w1441]
              n752 = local read "Transport Line Color"() -> (w1440:u32)
              n753 = local read "Ring"() -> (w1439:u16)
              n754 = property on="Transport" class="XYGraph (strict)"("Active Plot"=w1441, "Plot.Plot Color"=w1440, "Plot.Line Width"=w1439) -> ()  [unwired: 2 in, 2 out]
            }
            n755 = call <vilib>:"Check if File or Folder Exists.vi"("error in (no error)"=w1396, "path"=w1397) -> ("file or folder exists?"=w1394:bool, "dup path"=w1395:path)  [unwired: 7 in, 1 out]
            n756 = case shown="True" w1394 {
              tunnel: w1395 -> [_ w1447]
              frame False {
              }
              frame True {
                n757 = Read from Text File(file (use dialog)=w1447) -> (text=w1451:string)  [unwired: 3 in, 3 out]
                n758 = property on="Image Out" class="ImageControl"() -> ("ROI"=w1448:T14)  [unwired: 2 in, 2 out]
                n759 = Unflatten From String(type=w1448, binary string=w1451) -> (value=w1449:T14, error out=w1450:errorcluster)  [unwired: 3 in, 1 out]
                n760 = property on="Image Out" class="ImageControl"(error in=w1450, "ROI"=w1449) -> ()  [unwired: 1 in, 2 out]
              }
            }
            n761 = invoke on="Image Out" class="ImageControl" method="Clear ROI"() -> ()  [unwired: 3 in, 3 out]
            n762 = call-poly <vilib>:"Read From Spreadsheet File.vi"("file path (dialog if empty)"=w1260) -> ("all rows"=w1264:string[][])  [unwired: 6 in, 4 out]
            n763 = Array Size(array=w1264) -> (size(s)=w1283:i32[])
            n764 = Index Array(array=w1283, index=0) -> (element=w1281:i32)
            n765 = Path To String(path=w1389) -> (string=w1421:string)
            n766 = Index Array(array=w1423, index=w1422) -> (element=w1401:string)
            n767 = Concatenate Strings(w1421, "\\", w1401) -> (w1420:string)
            n768 = Array Subset(array=w1264, index (row)=w1282, index (col)=w1282, length (col)=3) -> (w1284:string[][])  [unwired: 1 in]
            n769 = local write "Image Name"(w1401) -> ()
            n770 = String To Path(string=w1420) -> (path=w1400:path)
            n771 = Empty String/Path?(string/path=w1401) -> (empty?=w1402:bool)
            n772 = local read "No Image File"() -> (w1398:path)
            n773 = Reshape Array(w1284, w1281) -> (w1266:string[])
            n774 = Search 1D Array(1D array=w1266, element="Vg") -> (index of element=w1270:i32)  [unwired: 1 in]
            n775 = Add(x=w1270, y=3) -> (x+y=w1268:i32)
            n776 = Divide(x=w1268, y=3) -> (x/y=w1275:dbl)
            n777 = Array Subset(array=w1264, index (row)=w1275, index (col)=0, length (col)=1) -> (w1274:string[][])  [unwired: 1 in]
            n778 = Fract/Exp String To Number(string=w1274) -> (number=w1278:dbl[][])  [unwired: 3 in, 1 out]
            n779 = Array Size(array=w1278) -> (size(s)=w1265:i32[])
            n780 = Index Array(array=w1265, index=0) -> (element=w1276:i32)
            n781 = Decrement(x=w1276) -> (x-1=w1279:i32)
            n782 = Reshape Array(w1278, w1279) -> (w1263:dbl[])
            n783 = local write "Data Length"(w1279) -> ()
            n784 = local write "Vg Column"(w1263) -> ()
            n785 = Select(t=w1398, s=w1402, f=w1400) -> (s? t:f=w1399:path)
            n786 = local write "Image File"(w1399) -> ()
            n787 = Array Max & Min(array=w1263) -> (max value=w1262:dbl, min value=w1261:dbl)  [unwired: 2 out]
            n788 = property on="Sat-Trans Slider" class="Slide (strict)"("Scale.Maximum"=w1262, "Scale.Minimum"=w1261) -> ()  [unwired: 2 in, 2 out]
            n789 = call "Vision Acquisition3"("Image Path"=w1399) -> ("Image Out"=w1424:T2)  [unwired: 25 in, 1 out]
            n790 = local write "Image Out"(w1424) -> ()
            n791 = local write "Image Out 2"(w1424) -> ()
          }
          event "Up Button": Mouse Down {
            w1599 = 0
            w1615 = "\\"
            w1616 = "TSP"
            w1754 = 0
            # "Transpose"
            n792 = event-data() -> ()  [unwired: 1 in, 5 out]
            n793 = local read "Transfer File"() -> (w1750:path)
            n794 = Strip Path(path=w1750) -> (stripped path=w1607:path, name=w1764:string)
            n795 = local write "Transfer Folder"(w1607) -> ()
            n796 = List Folder(path=w1607) -> (filenames=w1759:string[], error out=w1717:errorcluster)  [unwired: 3 in, 2 out]
            n797 = Array Size(array=w1759) -> (size(s)=w1705:i32)
            n798 = Search 1D Array(1D array=w1759, element=w1764) -> (index of element=w1760:i32)  [unwired: 1 in]
            n799 = Equal To 0?(x=w1760) -> (x = 0?=w1761:bool)
            n800 = local read "Folder Index"() -> (w1704:dbl)
            n801 = property on="Image Out" class="ImageControl"() -> (error out=w1707:errorcluster, "Image Center Position"=w1711:cluster{"X":u32, "Y":u32})  [unwired: 2 in, 1 out]
            n802 = Strip Path(path=w1607) -> (stripped path=w1611:path)  [unwired: 1 out]
            n803 = Path To String(path=w1611) -> (string=w1614:string)
            n804 = case shown="True" w1761 {
              tunnel: w1704 -> [w1905 _]
              tunnel: [w1904 w1906] -> w1703
              tunnel: w1705 -> [_ w1907]
              frame False {
                n805 = Decrement(x=w1905) -> (x-1=w1904:dbl)
              }
              frame True {
                n806 = Decrement(x=w1907) -> (x-1=w1906:i32)
              }
            }
            n807 = Unbundle(w1711) -> ("X"=w1709:u32)  [unwired: 1 out]
            n808 = local write "Folder Index"(w1703) -> ()
            n809 = local read "Folder Index"() -> (w1639:dbl)
            n810 = Bundle("X"=w1709, 0) -> (w1710:cluster{"X":u32, i32})  [unwired: 1 in]
            n811 = Path To String(path=w1607) -> (string=w1765:string)
            n812 = Index Array(array=w1759, index=w1703) -> (element=w1608:string)
            n813 = String Subset(string=w1608, offset (0)=3) -> (substring=w1610:string)  [unwired: 1 in]
            n814 = Concatenate Strings(w1616, w1610) -> (w1612:string)
            n815 = Concatenate Strings(w1614, w1615, w1616, w1615, w1612) -> (w1613:string)
            n816 = String To Path(string=w1613) -> (path=w1606:path)
            n817 = local write "Transport File"(w1606) -> ()
            n818 = Strip Path(path=w1606) -> (stripped path=w1640:path, name=w1645:string)
            n819 = local write "Transport Folder"(w1640) -> ()
            n820 = List Folder(path=w1640) -> (filenames=w1641:string[], error out=w1637:errorcluster)  [unwired: 3 in, 2 out]
            n821 = Array Size(array=w1641) -> (size(s)=w1603:i32)
            n822 = Search 1D Array(1D array=w1641, element=w1645) -> (index of element=w1605:i32)  [unwired: 1 in]
            n823 = local write "Data Name:"(w1608) -> ()
            n824 = property on="Image Out" class="ImageControl"(error in=w1707, "Image Center Position"=w1710) -> ()  [unwired: 1 in, 2 out]
            n825 = Equal To 0?(x=w1605) -> (x = 0?=w1604:bool)
            n826 = case shown="False" w1604 {
              tunnel: w1639 -> [w1768 _]
              tunnel: [w1767 w1769] -> w1638
              tunnel: w1637 -> [w1766 w1770]
              tunnel: [w1766 w1770] -> _
              tunnel: w1603 -> [_ w1769]
              frame False {
                n827 = Decrement(x=w1768) -> (x-1=w1767:dbl)
              }
              frame True {
              }
            }
            n828 = local write "Folder Index"(w1638) -> ()
            n829 = Concatenate Strings(w1765, "\\", w1608) -> (w1763:string)
            n830 = Path To String(path=w1640) -> (string=w1646:string)
            n831 = Index Array(array=w1641, index=w1638) -> (element=w1642:string)
            n832 = String To Path(string=w1763) -> (path=w1577:path)
            n833 = call "Recorded Values.vi"("Path"=w1577) -> ("Recorded Char"=w1701:T6, "Recorded Prop"=w1700:T7, "Fabrication Prop"=w1702:T8)  [unwired: 8 in]
            n834 = Unbundle By Name(w1701) -> ("Mobility-Sat"=w1688:dbl, "Moblitity-Lin"=w1687:dbl, "On/Off"=w1686:dbl, "Off Current"=w1685:dbl, "Vt-Sat"=w1655:dbl, "STS"=w1684:dbl, "Trap Density-VT"=w1683:dbl, "Trap Density-STS"=w1682:dbl)
            n835 = Unbundle By Name(w1702) -> ("Date Created"=w1681:string, "Material"=w1699:string, "Solvent"=w1698:string, "Concentration"=w1697:dbl, "Method"=w1696:string, "Dielectric (nm)"=w1695:dbl, "Treatment"=w1694:string, "Comments"=w1693:string)
            n836 = Unbundle By Name(w1700) -> ("Date Recorded"=w1692:string, "Index"=w1691:string, "Length"=w1690:dbl, "Width"=w1689:dbl, "Sample Temp"=w1656:dbl)
            n837 = local write "Date Created"(w1681) -> ()
            n838 = local write "Rec: Material"(w1699) -> ()
            n839 = local write "Rec: Off I-Sat"(w1685) -> ()
            n840 = local write "Rec: Comments"(w1693) -> ()
            n841 = local write "Rec: VT-Sat"(w1655) -> ()
            n842 = local write "Rec: Solvent"(w1698) -> ()
            n843 = local write "Rec: Concentration"(w1697) -> ()
            n844 = local write "Rec: Method"(w1696) -> ()
            n845 = local write "Rec: Dielectric (d)"(w1695) -> ()
            n846 = local write "Surface Treatment:"(w1694) -> ()
            n847 = local write "Index"(w1691) -> ()
            n848 = local write "Rec: Mobility-Sat"(w1688) -> ()
            n849 = local write "Rec: Mobility-Lin"(w1687) -> ()
            n850 = local write "Rec: On/Off"(w1686) -> ()
            n851 = local write "Rec: STS"(w1684) -> ()
            n852 = local write "Rec: Trap Density-VT"(w1683) -> ()
            n853 = local write "Rec: Trap Density-STS"(w1682) -> ()
            n854 = local write "Date Recorded"(w1692) -> ()
            n855 = local write "Rec: Length"(w1690) -> ()
            n856 = local write "Rec: Width"(w1689) -> ()
            n857 = local write "Rec: Temp"(w1656) -> ()
            n858 = Equal To 0?(x=w1656) -> (x = 0?=w1658:bool)
            n859 = case shown="False" w1658 {
              tunnel: [w1777 w1778] -> w1657
              tunnel: w1656 -> [w1777 _]
              frame False {
              }
              frame True {
                n860 = local read "Room Temp"() -> (w1778:dbl)
              }
            }
            n861 = local write "Data Name:"(w1642) -> ()
            n862 = local read "NumPoints Log"() -> (w1678:dbl)
            n863 = local write "Transfer File"(w1577) -> ()
            n864 = local read "Num Pts"() -> (w1680:dbl)
            n865 = Concatenate Strings(w1646, "\\", w1642) -> (w1644:string)
            n866 = local read "New: Dielectric"() -> (w1664:dbl)
            n867 = call "Mobility-Vt Calculator-File.vi"("NumPts"=w1680, "Path"=w1577) -> ("Used Points"=w1576:T10, "Graph Cluster"=w1653:T11, "Output"=w1679:T12)  [unwired: 6 in, 1 out]
            n868 = Unbundle By Name(w1576) -> ("Index-Lin"=w1574:dbl, "Index-Sat"=w1575:dbl)
            n869 = call "STS Calculator-File.vi"("NumPts"=w1678, "Path"=w1577) -> ("Used Points"=w1573:T9, "XY Graph-Sat"=w1677:cluster{dbl[], dbl[]}[], "Ouput"=w1676:cluster{"STS-Sat":dbl, "STS-Lin":dbl})  [unwired: 6 in, 1 out]
            n870 = Unbundle By Name(w1573) -> ("STS Index-Sat"=w1572:dbl)
            n871 = call-poly <vilib>:"Read From Spreadsheet File.vi"("file path (dialog if empty)"=w1577) -> ("all rows"=w1756:string[][])  [unwired: 6 in, 4 out]
            n872 = String To Path(string=w1644) -> (path=w1647:path)
            n873 = Unbundle By Name(w1679) -> ("Mobility-Sat"=w1667:dbl, "Vt-Sat"=w1660:dbl, "Mobility-Lin"=w1666:dbl, "Vt-Lin"=w1665:dbl, "Off I-Sat"=w1659:dbl, "On/Off I-Sat"=w1654:dbl)
            n874 = Strip Path(path=w1647) -> ()  [unwired: 2 out]
            n875 = call-poly <vilib>:"Read From Spreadsheet File.vi"("file path (dialog if empty)"=w1647) -> ("all rows"=w1623:string[][])  [unwired: 6 in, 4 out]
            n876 = local write "Sat-Trans Slider"(w1575) -> ()
            n877 = Unbundle By Name(w1676) -> ("STS-Sat"=w1661:dbl)  [unwired: 1 out]
            n878 = local write "Index 2"(w1572) -> ()
            n879 = local write "MobVi Index"(w1575) -> ()
            n880 = local write "Sat-Log"(w1677) -> ()
            n881 = Array Size(array=w1623) -> (size(s)=w1617:i32[])
            n882 = local write "Calc: Mobility-Sat"(w1667) -> ()
            n883 = local write "Calc: VT-Sat"(w1660) -> ()
            n884 = local write "Calc: Mobility-Lin"(w1666) -> ()
            n885 = local write "Calc: Off I-Sat"(w1659) -> ()
            n886 = local write "Calc: On/Off"(w1654) -> ()
            n887 = Array Size(array=w1756) -> (size(s)=w1755:i32[])
            n888 = local write "Calc: VT-Lin"(w1665) -> ()
            n889 = call "Trap Density_VT.vi"("VT"=w1660, "Dielectric"=w1664) -> ("Trap Density-VT"=w1663:dbl)
            n890 = call "Trap Density_STS.vi"("Temp (T) [K]"=w1657, "S.T.S. (S)"=w1661, "Dielectric"=w1664) -> ("Trap Density (N)"=w1662:dbl)  [unwired: 8 in]
            n891 = Unbundle By Name(w1653) -> ("Raw Sat"=w1650:cluster{dbl[], dbl[]}[], "Sqrt Sat"=w1651:cluster{dbl[], dbl[]}[], "Raw Lin"=w1649:cluster{dbl[], dbl[]}[], "Sqrt Lin"=w1652:cluster{dbl[], dbl[]}[], "Log Lin"=w1648:cluster{dbl[], dbl[]}[])  [unwired: 1 out]
            n892 = local write "Sqrt-Sat"(w1651) -> ()
            n893 = local write "Calc: STS"(w1661) -> ()
            n894 = local write "New: STS"(w1661) -> ()
            n895 = Array Subset(array=w1623, length (col)=1) -> (w1621:string[][])  [unwired: 3 in]
            n896 = Index Array(array=w1617, index=0) -> (element=w1628:i32)
            n897 = Decimate 1D Array(w1652) -> (w1675:cluster{dbl[], dbl[]}[])  [unwired: 1 out]
            n898 = local write "Calc: Trap Density-VT"(w1663) -> ()
            n899 = local write "New: VT-Sat"(w1660) -> ()
            n900 = local write "Calc: Trap Density-STS"(w1662) -> ()
            n901 = local write "New: Trap Density-STS"(w1662) -> ()
            n902 = local write "New: Trap Density-VT"(w1663) -> ()
            n903 = Reshape Array(w1621, w1628) -> (w1622:string[])
            n904 = local write "New: VT-Lin"(w1665) -> ()
            n905 = local write "Sqrt-Lin"(w1652) -> ()
            n906 = local write "New: Mobility-Sat"(w1667) -> ()
            n907 = local write "New: Mobility-Lin"(w1666) -> ()
            n908 = Decimate 1D Array(w1677) -> (w1734:cluster{dbl[], dbl[]}[])  [unwired: 1 out]
            n909 = Index Array(array=w1755, index=w1754) -> (element=w1740:i32)
            n910 = Decimate 1D Array(w1651) -> (w1744:cluster{dbl[], dbl[]}[])  [unwired: 1 out]
            n911 = Array To Cluster(array=w1675) -> (cluster=w1674:T13)
            n912 = Array Subset(array=w1756, index (row)=w1754, index (col)=w1754, length (col)=3) -> (w1757:string[][])  [unwired: 1 in]
            n913 = Search 1D Array(1D array=w1622, element="Vd") -> (index of element=w1624:i32)  [unwired: 1 in]
            n914 = local write "Raw- Sat"(w1650) -> ()
            n915 = local write "Raw- Lin"(w1649) -> ()
            n916 = local write "Log-Lin"(w1648) -> ()
            n917 = Array To Cluster(array=w1734) -> (cluster=w1732:T13)
            n918 = Array To Cluster(array=w1744) -> (cluster=w1746:T13)
            n919 = Reshape Array(w1757, w1740) -> (w1747:string[])
            n920 = Increment(x=w1624) -> (x+1=w1625:i32)
            n921 = Array Subset(array=w1623, index (row)=w1625) -> (w1627:string[][])  [unwired: 3 in]
            n922 = Subtract(x=w1740, y=20) -> (x-y=w1739:i32)
            n923 = Unbundle(w1674) -> ("[0]"=w1671:cluster{dbl[], dbl[]})  [unwired: 8 out]
            n924 = Fract/Exp String To Number(string=w1627, default (0 dbl)="default (0 dbl) 6") -> (number=w1635:ext[][])  [unwired: 2 in, 1 out]
            n925 = Delete From Array(array=w1635) -> (array with subset deleted=w1636:ext[][])  [unwired: 3 in, 1 out]
            n926 = property on="Sat-Trans Slider" class="Slide (strict)"("Scale.Maximum"=w1739) -> ()  [unwired: 2 in, 2 out]
            n927 = Delete From Array(array=w1636, index (col)=0 ("Deaktivierter Index (Spalte)")) -> (deleted portion=w1631:ext[], array with subset deleted=w1630:ext[][])  [unwired: 2 in]
            n928 = local read "Num Pts"() -> (w1668:dbl)
            n929 = Unbundle(w1732) -> ("[0]"=w1733:cluster{dbl[], dbl[]})  [unwired: 8 out]
            n930 = Unbundle(w1746) -> ("[0]"=w1745:cluster{dbl[], dbl[]})  [unwired: 8 out]
            n931 = Unbundle(w1671) -> (w1670:dbl[], w1669:dbl[])
            n932 = Search 1D Array(1D array=w1747, element="Index:") -> (index of element=w1751:i32)  [unwired: 1 in]
            n933 = Transpose 2D Array(2D array=w1630) -> (transposed array=w1629:ext[][])
            n934 = Increment(x=w1751) -> (x+1=w1752:i32)
            n935 = Unbundle(w1733) -> (w1731:dbl[], w1730:dbl[])
            n936 = Unbundle(w1745) -> (w1738:dbl[], w1737:dbl[])
            n937 = for {
              tunnel: w1631 -> [w1775]
              tunnel: w1629 -> [w1776] mode=indexing
              tunnel: [w1774] -> w1633 mode=indexing
              n938 = Bundle(w1775, w1776) -> (w1774:cluster{ext[], ext[]})  [unwired: 1 in]
            }
            n939 = Array Subset(array=w1670, index=w1574, length=w1668) -> (w1672:dbl[])
            n940 = Array Subset(array=w1669, index=w1574, length=w1668) -> (w1673:dbl[])
            n941 = local read "Image Folder"() -> (w1706:path)
            n942 = local write "Lin-Vg Array-Used"(w1672) -> ()
            n943 = Array Subset(array=w1731, index=w1572, length=w1678) -> (w1736:dbl[])
            n944 = Array Subset(array=w1730, index=w1572, length=w1678) -> (w1735:dbl[])
            n945 = Array Subset(array=w1738, index=w1575, length=w1680) -> (w1743:dbl[])
            n946 = Array Subset(array=w1737, index=w1575, length=w1680) -> (w1742:dbl[])
            n947 = local write "Lin Id-Used"(w1673) -> ()
            n948 = local write "Transport"(w1633) -> ()
            n949 = Index Array(array=w1747, index=w1752) -> (element=w1713:string)
            n950 = Array Size(array=w1633) -> (size(s)=w1634:i32)
            n951 = for {
              N: w1634 -> [_]
              i -> [w1773]
              n952 = local read "Transport Line Color"() -> (w1772:u32)
              n953 = local read "Ring"() -> (w1771:u16)
              n954 = property on="Transport" class="XYGraph (strict)"("Active Plot"=w1773, "Plot.Plot Color"=w1772, "Plot.Line Width"=w1771) -> ()  [unwired: 2 in, 2 out]
            }
            n955 = local write "Sat Vg Array-Used"(w1743) -> ()
            n956 = local write "Vg Array-Log-Used"(w1735) -> ()
            n957 = local write "Sat Id-Log-Used"(w1736) -> ()
            n958 = local write "Sat Id-Used"(w1742) -> ()
            n959 = local write "Index"(w1713) -> ()
            n960 = List Folder(path=w1706, error in=w1717) -> (filenames=w1749:string[], error out=w1716:errorcluster)  [unwired: 2 in, 2 out]
            n961 = Build Path(base path=w1706, name or relative path="ROI") -> (appended path=w1714:path)
            n962 = invoke on="Image Out" class="ImageControl" method="Clear ROI"(error in=w1716) -> (error out=w1720:errorcluster)  [unwired: 2 in, 2 out]
            n963 = while {
              tunnel: w1749 -> [w1791]
              tunnel: w1713 -> [w1789]
              tunnel: [w1788] -> w1748
              tunnel: w1740 -> [w1787]
              i -> [w1788]
              stop <- w1784 stop-if-true
              n964 = Index Array(array=w1791, index=w1788) -> (element=w1792:string)
              n965 = xnode "Match Regular Expression"("input string"=w1792, "regular expression"=w1789) -> ("whole match"=w1790:string)  [unwired: 4 in, 4 out]
              n966 = Equal?(x=w1790, y=w1789) -> (x = y?=w1786:bool)
              n967 = Equal?(x=w1787, y=w1788) -> (x = y?=w1785:bool)
              n968 = Or(x=w1786, y=w1785) -> (x .or. y?=w1784:bool)
            }
            n969 = Build Path(base path=w1714, name or relative path=w1713) -> (appended path=w1712:path)
            n970 = call <vilib>:"Check if File or Folder Exists.vi"("error in (no error)"=w1720, "path"=w1712) -> ("file or folder exists?"=w1718:bool, "dup path"=w1719:path)  [unwired: 7 in, 1 out]
            n971 = case shown="True" w1718 {
              tunnel: w1719 -> [_ w1779]
              frame False {
              }
              frame True {
                n972 = Read from Text File(file (use dialog)=w1779) -> (text=w1783:string)  [unwired: 3 in, 3 out]
                n973 = property on="Image Out" class="ImageControl"() -> ("ROI"=w1780:T14)  [unwired: 2 in, 2 out]
                n974 = Unflatten From String(type=w1780, binary string=w1783) -> (value=w1781:T14, error out=w1782:errorcluster)  [unwired: 3 in, 1 out]
                n975 = property on="Image Out" class="ImageControl"(error in=w1782, "ROI"=w1781) -> ()  [unwired: 1 in, 2 out]
              }
            }
            n976 = call-poly <vilib>:"Read From Spreadsheet File.vi"("file path (dialog if empty)"=w1577) -> ("all rows"=w1581:string[][])  [unwired: 6 in, 4 out]
            n977 = Array Size(array=w1581) -> (size(s)=w1600:i32[])
            n978 = Index Array(array=w1600, index=0) -> (element=w1598:i32)
            n979 = Index Array(array=w1749, index=w1748) -> (element=w1722:string)
            n980 = local write "Image Name"(w1722) -> ()
            n981 = Array Subset(array=w1581, index (row)=w1599, index (col)=w1599, length (col)=3) -> (w1601:string[][])  [unwired: 1 in]
            n982 = Empty String/Path?(string/path=w1722) -> (empty?=w1729:bool)
            n983 = Build Path(base path=w1706, name or relative path=w1722) -> (appended path=w1721:path)
            n984 = local read "No Image File"() -> (w1728:path)
            n985 = Reshape Array(w1601, w1598) -> (w1583:string[])
            n986 = Search 1D Array(1D array=w1583, element="Vg") -> (index of element=w1587:i32)  [unwired: 1 in]
            n987 = Add(x=w1587, y=3) -> (x+y=w1585:i32)
            n988 = Divide(x=w1585, y=3) -> (x/y=w1592:dbl)
            n989 = Array Subset(array=w1581, index (row)=w1592, index (col)=0, length (col)=1) -> (w1591:string[][])  [unwired: 1 in]
            n990 = Fract/Exp String To Number(string=w1591) -> (number=w1595:dbl[][])  [unwired: 3 in, 1 out]
            n991 = Array Size(array=w1595) -> (size(s)=w1582:i32[])
            n992 = Index Array(array=w1582, index=0) -> (element=w1593:i32)
            n993 = Decrement(x=w1593) -> (x-1=w1596:i32)
            n994 = Reshape Array(w1595, w1596) -> (w1580:dbl[])
            n995 = local write "Data Length"(w1596) -> ()
            n996 = local write "Vg Column"(w1580) -> ()
            n997 = Array Max & Min(array=w1580) -> (max value=w1579:dbl, min value=w1578:dbl)  [unwired: 2 out]
            n998 = Select(t=w1728, s=w1729, f=w1721) -> (s? t:f=w1723:path)
            n999 = call <vilib>:"Get File Extension.vi"("file"=w1723) -> ("lowercase file extension"=w1725:string)  [unwired: 7 in, 3 out]
            n1000 = local write "Image File"(w1723) -> ()
            n1001 = local write "String"(w1725) -> ()
            n1002 = property on="Sat-Trans Slider" class="Slide (strict)"("Scale.Maximum"=w1579, "Scale.Minimum"=w1578) -> ()  [unwired: 2 in, 2 out]
            n1003 = Search 1D Array(1D array=string[] ["bmp", "jpeg", "png", "jpg", "gif"], element=w1725) -> (index of element=w1724:i32)  [unwired: 1 in]
            n1004 = call "Vision Acquisition5"("Image Path"=w1723) -> ("Image Out"=w1727:T2)  [unwired: 25 in, 1 out]
            n1005 = Less Than 0?(x=w1724) -> ()  [unwired: 1 out]
            n1006 = local write "Image Out"(w1727) -> ()
            n1007 = local write "Image Out 2"(w1727) -> ()
          }
          event "Save Changes? 3": Mouse Down {
            n1008 = event-data() -> ()  [unwired: 1 in, 7 out]
            n1009 = local read "Image Folder"() -> (w1908:path)
            n1010 = Build Path(base path=w1908, name or relative path="ROI") -> (appended path=w1915:path)
            n1011 = call <vilib>:"Check if File or Folder Exists.vi"("path"=w1915) -> ("file or folder exists?"=w1917:bool, "dup path"=w1914:path)  [unwired: 8 in, 1 out]
            n1012 = case shown="False" w1917 {
              tunnel: w1914 -> [w1919 w1920]
              tunnel: [w1918 w1920] -> w1909
              frame False {
                n1013 = Create Folder(path (use dialog)=w1919) -> (created path=w1918:path)  [unwired: 2 in, 2 out]
              }
              frame True {
              }
            }
            n1014 = local read "Index"() -> (w1911:string)
            n1015 = property on="Image Out" class="ImageControl"() -> ("ROI"=w1913:T14)  [unwired: 2 in, 2 out]
            n1016 = Build Path(base path=w1909, name or relative path=w1911) -> (appended path=w1910:path)
            n1017 = Flatten To String(anything=w1913) -> (data string=w1912:string)  [unwired: 3 in, 2 out]
            n1018 = Write to Text File(file (use dialog)=w1910, text=w1912) -> ()  [unwired: 2 in, 3 out]
          }
          event "Next Sqrt Sat": Mouse Down {
            n1019 = event-data() -> ()  [unwired: 1 in, 5 out]
            n1020 = local read "Sqrt-Sat"() -> (w1933:cluster{dbl[], dbl[]}[])
            n1021 = Decimate 1D Array(w1933) -> (w1929:cluster{dbl[], dbl[]}[], w1928:cluster{dbl[], dbl[]}[])
            n1022 = Array To Cluster(array=w1929) -> (cluster=w1939:T13)
            n1023 = Unbundle(w1939) -> ("[0]"=w1938:cluster{dbl[], dbl[]})  [unwired: 8 out]
            n1024 = local read "MobVi Index"() -> (w1935:dbl)
            n1025 = local read "Num Pts"() -> (w1934:dbl)
            n1026 = Unbundle(w1938) -> (w1937:dbl[], w1936:dbl[])
            n1027 = Increment(x=w1935) -> (x+1=w1930:dbl)
            n1028 = local read "New: Dielectric"() -> (w1924:dbl)
            n1029 = local read "New: Length"() -> (w1923:dbl)
            n1030 = local read "New: Width"() -> (w1922:dbl)
            n1031 = local write "MobVi Index"(w1930) -> ()
            n1032 = Array Subset(array=w1937, index=w1930, length=w1934) -> (w1926:dbl[])
            n1033 = Array Subset(array=w1936, index=w1930, length=w1934) -> (w1925:dbl[])
            n1034 = local write "Sat Vg Array-Used"(w1926) -> ()
            n1035 = local write "Sat Id-Used"(w1925) -> ()
            n1036 = call "Mobility-Vt-Used Pts_Saturation.vi"("Width"=w1922, "Length"=w1923, "Dielectric (d)"=w1924, "Sat Id Used"=w1925, "Vg Used"=w1926) -> ("Vt"=w1921:dbl, "Mobility"=w1927:dbl)  [unwired: 4 in, 1 out]
            n1037 = Bundle(w1926, w1925) -> (w1932:cluster{dbl[], dbl[]})  [unwired: 1 in]
            n1038 = Build Array (concatenate)(w1929, w1928, w1932) -> (w1931:cluster{dbl[], dbl[]}[])
            n1039 = local write "New: Mobility-Sat"(w1927) -> ()
            n1040 = local write "New: VT-Sat"(w1921) -> ()
            n1041 = local write "Sqrt-Sat"(w1931) -> ()
          }
          event "Next Log Sat": Mouse Down {
            n1042 = event-data() -> ()  [unwired: 1 in, 7 out]
            n1043 = local read "Sat-Log"() -> (w1948:cluster{dbl[], dbl[]}[])
            n1044 = Decimate 1D Array(w1948) -> (w1944:cluster{dbl[], dbl[]}[], w1943:cluster{dbl[], dbl[]}[])
            n1045 = Array To Cluster(array=w1944) -> (cluster=w1954:T13)
            n1046 = local read "Index 2"() -> (w1950:dbl)
            n1047 = local read "NumPoints Log"() -> (w1949:dbl)
            n1048 = Unbundle(w1954) -> ("[0]"=w1953:cluster{dbl[], dbl[]})  [unwired: 8 out]
            n1049 = Unbundle(w1953) -> (w1952:dbl[], w1951:dbl[])
            n1050 = Increment(x=w1950) -> (x+1=w1945:dbl)
            n1051 = local write "Index 2"(w1945) -> ()
            n1052 = Array Subset(array=w1951, index=w1945, length=w1949) -> (w1940:dbl[])
            n1053 = Array Subset(array=w1952, index=w1945, length=w1949) -> (w1941:dbl[])
            n1054 = call "STS-Used.vi"("Id Used"=w1941, "Vg-Used"=w1940) -> ("STS"=w1942:dbl)  [unwired: 9 in]
            n1055 = Bundle(w1941, w1940) -> (w1947:cluster{dbl[], dbl[]})  [unwired: 1 in]
            n1056 = local write "Vg Array-Log-Used"(w1940) -> ()
            n1057 = local write "Sat Id-Log-Used"(w1941) -> ()
            n1058 = local write "New: STS"(w1942) -> ()
            n1059 = Build Array (concatenate)(w1944, w1943, w1947) -> (w1946:cluster{dbl[], dbl[]}[])
            n1060 = local write "Sat-Log"(w1946) -> ()
          }
          event "Previous Log Sat": Mouse Down {
            n1061 = event-data() -> ()  [unwired: 1 in, 7 out]
            n1062 = local read "Sat-Log"() -> (w1964:cluster{dbl[], dbl[]}[])
            n1063 = Decimate 1D Array(w1964) -> (w1961:cluster{dbl[], dbl[]}[], w1960:cluster{dbl[], dbl[]}[])
            n1064 = Array To Cluster(array=w1961) -> (cluster=w1969:T13)
            n1065 = local read "Index 2"() -> (w1957:dbl)
            n1066 = local read "NumPoints Log"() -> (w1965:dbl)
            n1067 = Unbundle(w1969) -> ("[0]"=w1968:cluster{dbl[], dbl[]})  [unwired: 8 out]
            n1068 = Unbundle(w1968) -> (w1967:dbl[], w1966:dbl[])
            n1069 = Decrement(x=w1957) -> (x-1=w1958:dbl)
            n1070 = local write "Index 2"(w1958) -> ()
            n1071 = Array Subset(array=w1967, index=w1958, length=w1965) -> (w1955:dbl[])
            n1072 = Array Subset(array=w1966, index=w1958, length=w1965) -> (w1956:dbl[])
            n1073 = local write "Sat Id-Log-Used"(w1955) -> ()
            n1074 = Bundle(w1955, w1956) -> (w1963:cluster{dbl[], dbl[]})  [unwired: 1 in]
            n1075 = call "STS-Used.vi"("Id Used"=w1955, "Vg-Used"=w1956) -> ("STS"=w1959:dbl)  [unwired: 9 in]
            n1076 = local write "Vg Array-Log-Used"(w1956) -> ()
            n1077 = Build Array (concatenate)(w1961, w1960, w1963) -> (w1962:cluster{dbl[], dbl[]}[])
            n1078 = local write "New: STS"(w1959) -> ()
            n1079 = local write "Sat-Log"(w1962) -> ()
          }
          event "Previous Sqrt Sat": Mouse Down {
            n1080 = event-data() -> ()  [unwired: 1 in, 5 out]
            n1081 = local read "Sqrt-Sat"() -> (w1983:cluster{dbl[], dbl[]}[])
            n1082 = Decimate 1D Array(w1983) -> (w1980:cluster{dbl[], dbl[]}[], w1979:cluster{dbl[], dbl[]}[])
            n1083 = Array To Cluster(array=w1980) -> (cluster=w1988:T13)
            n1084 = local read "MobVi Index"() -> (w1978:dbl)
            n1085 = Unbundle(w1988) -> ("[0]"=w1987:cluster{dbl[], dbl[]})  [unwired: 8 out]
            n1086 = local read "Num Pts"() -> (w1984:dbl)
            n1087 = Unbundle(w1987) -> (w1986:dbl[], w1985:dbl[])
            n1088 = Decrement(x=w1978) -> (x-1=w1977:dbl)
            n1089 = local read "New: Dielectric"() -> (w1971:dbl)
            n1090 = local read "New: Length"() -> (w1972:dbl)
            n1091 = local read "New: Width"() -> (w1973:dbl)
            n1092 = local write "MobVi Index"(w1977) -> ()
            n1093 = Array Subset(array=w1986, index=w1977, length=w1984) -> (w1976:dbl[])
            n1094 = Array Subset(array=w1985, index=w1977, length=w1984) -> (w1975:dbl[])
            n1095 = local write "Sat Vg Array-Used"(w1976) -> ()
            n1096 = local write "Sat Id-Used"(w1975) -> ()
            n1097 = call "Mobility-Vt-Used Pts_Linear.vi"("Width"=w1973, "Length"=w1972, "Dielectric (d)"=w1971, "Id Used"=w1975, "Vg Used"=w1976) -> ("Vt"=w1970:dbl, "Mobility"=w1974:dbl)  [unwired: 4 in, 1 out]
            n1098 = Bundle(w1976, w1975) -> (w1982:cluster{dbl[], dbl[]})  [unwired: 1 in]
            n1099 = local write "New: VT-Sat"(w1970) -> ()
            n1100 = Build Array (concatenate)(w1980, w1979, w1982) -> (w1981:cluster{dbl[], dbl[]}[])
            n1101 = local write "New: Mobility-Sat"(w1974) -> ()
            n1102 = local write "Sqrt-Sat"(w1981) -> ()
          }
          event "Sat-Trans Slider": Value Change {
            n1103 = event-data() -> ()  [unwired: 1 in, 5 out]
            n1104 = local read "Sqrt-Sat"() -> (w2001:cluster{dbl[], dbl[]}[])
            n1105 = Decimate 1D Array(w2001) -> (w1998:cluster{dbl[], dbl[]}[], w1997:cluster{dbl[], dbl[]}[])
            n1106 = Array To Cluster(array=w1998) -> (cluster=w2006:T13)
            n1107 = Unbundle(w2006) -> ("[0]"=w2005:cluster{dbl[], dbl[]})  [unwired: 8 out]
            n1108 = local read "Sat-Trans Slider"() -> (w1990:dbl)
            n1109 = local read "Num Pts"() -> (w2002:dbl)
            n1110 = Unbundle(w2005) -> (w2004:dbl[], w2003:dbl[])
            n1111 = local read "New: Dielectric"() -> (w1991:dbl)
            n1112 = local read "New: Length"() -> (w1992:dbl)
            n1113 = local read "New: Width"() -> (w1993:dbl)
            n1114 = local write "MobVi Index"(w1990) -> ()
            n1115 = Array Subset(array=w2004, index=w1990, length=w2002) -> (w1996:dbl[])
            n1116 = Array Subset(array=w2003, index=w1990, length=w2002) -> (w1995:dbl[])
            n1117 = local write "Sat Vg Array-Used"(w1996) -> ()
            n1118 = local write "Sat Id-Used"(w1995) -> ()
            n1119 = call "Mobility-Vt-Used Pts_Linear.vi"("Width"=w1993, "Length"=w1992, "Dielectric (d)"=w1991, "Id Used"=w1995, "Vg Used"=w1996) -> ("Vt"=w1989:dbl, "Mobility"=w1994:dbl)  [unwired: 4 in, 1 out]
            n1120 = Bundle(w1996, w1995) -> (w2000:cluster{dbl[], dbl[]})  [unwired: 1 in]
            n1121 = local write "New: VT-Sat"(w1989) -> ()
            n1122 = Build Array (concatenate)(w1998, w1997, w2000) -> (w1999:cluster{dbl[], dbl[]}[])
            n1123 = local write "New: Mobility-Sat"(w1994) -> ()
            n1124 = local write "Sqrt-Sat"(w1999) -> ()
          }
          event "Sat-Log Slider": Value Change {
            n1125 = event-data() -> ()  [unwired: 1 in, 5 out]
            n1126 = local read "Sat-Log"() -> (w2015:cluster{dbl[], dbl[]}[])
            n1127 = Decimate 1D Array(w2015) -> (w2012:cluster{dbl[], dbl[]}[], w2011:cluster{dbl[], dbl[]}[])
            n1128 = Array To Cluster(array=w2012) -> (cluster=w2020:T13)
            n1129 = Unbundle(w2020) -> ("[0]"=w2019:cluster{dbl[], dbl[]})  [unwired: 8 out]
            n1130 = local read "NumPoints Log"() -> (w2016:dbl)
            n1131 = local read "Sat-Log Slider"() -> (w2010:dbl)
            n1132 = Unbundle(w2019) -> (w2018:dbl[], w2017:dbl[])
            n1133 = local write "Index 2"(w2010) -> ()
            n1134 = Array Subset(array=w2018, index=w2010, length=w2016) -> (w2008:dbl[])
            n1135 = Array Subset(array=w2017, index=w2010, length=w2016) -> (w2007:dbl[])
            n1136 = local write "Vg Array-Log-Used"(w2007) -> ()
            n1137 = local write "Sat Id-Log-Used"(w2008) -> ()
            n1138 = call "STS-Used.vi"("Id Used"=w2008, "Vg-Used"=w2007) -> ("STS"=w2009:dbl)  [unwired: 9 in]
            n1139 = Bundle(w2008, w2007) -> (w2014:cluster{dbl[], dbl[]})  [unwired: 1 in]
            n1140 = local write "New: STS"(w2009) -> ()
            n1141 = Build Array (concatenate)(w2012, w2011, w2014) -> (w2013:cluster{dbl[], dbl[]}[])
            n1142 = local write "Sat-Log"(w2013) -> ()
          }
          event "Save Changes?": Mouse Down {
            n1143 = event-data() -> ()  [unwired: 1 in, 5 out]
            n1144 = flat-sequence {
              tunnel: [w2027] -> w2025
              tunnel: [w2035] -> w2024
              tunnel: [w2028] -> w2023
              tunnel: w2025 -> [w2567]
              tunnel: w2024 -> [w2564]
              tunnel: [w2565] -> w2022
              tunnel: w2023 -> [w2565]
              tunnel: [w2564] -> w2021
              tunnel: w2022 -> [w2572]
              tunnel: w2021 -> [w2571]
              frame #0 {
                n1145 = Wait (ms)(milliseconds to wait=1) -> ()  [unwired: 1 out]
              }
              frame #1 {
                n1146 = local read "Transfer File"() -> (w2027:path)
                n1147 = local read "New: Temp"() -> (w2029:dbl)
                n1148 = local read "New: Length"() -> (w2033:dbl)
                n1149 = local read "New: Width"() -> (w2031:dbl)
                n1150 = To Single Precision Float(number=w2029) -> (single precision float=w2030:sgl)
                n1151 = Number To Decimal String(number=w2030) -> (decimal integer string=w2038:string)  [unwired: 1 in]
                n1152 = To Single Precision Float(number=w2031) -> (single precision float=w2032:sgl)
                n1153 = To Single Precision Float(number=w2033) -> (single precision float=w2034:sgl)
                n1154 = local read "Index"() -> (w2043:string)
                n1155 = Strip Path(path=w2027) -> (stripped path=w2048:path)  [unwired: 1 out]
                n1156 = Number To Decimal String(number=w2034) -> (decimal integer string=w2041:string)  [unwired: 1 in]
                n1157 = Number To Decimal String(number=w2032) -> (decimal integer string=w2042:string)  [unwired: 1 in]
                n1158 = Concatenate Strings("_", w2038, "K") -> (w2036:string)
                n1159 = call "Build Text"("Temp"=w2036, "Index"=w2043, "Length"=w2041, "Width"=w2042) -> ("Result"=w2044:string)  [unwired: 10 in, 1 out]
                n1160 = flat-sequence {
                  tunnel: [w2521] -> w2040
                  tunnel: w2040 -> [w2538]
                  frame #0 {
                    # "Makes Empty File for Transformer Data"
                    n1161 = local read "Transfer Folder"() -> (w2510:path)
                    n1162 = Build Path(base path=w2510, name or relative path="Stats") -> (appended path=w2512:path)
                    n1163 = call <vilib>:"Check if File or Folder Exists.vi"("path"=w2512) -> ("file or folder exists?"=w2513:bool, "dup path"=w2514:path)  [unwired: 8 in, 1 out]
                    n1164 = case shown="False" w2513 {
                      tunnel: [w2518 w2520] -> w2515
                      tunnel: w2514 -> [w2519 w2520]
                      frame False {
                        n1165 = Create Folder(path (use dialog)=w2519) -> (created path=w2518:path)  [unwired: 2 in, 2 out]
                      }
                      frame True {
                      }
                    }
                    n1166 = Build Path(base path=w2515, name or relative path="Tranformer Data.txt") -> (appended path=w2517:path)
                    n1167 = call-poly <vilib>:"Write To Spreadsheet File.vi"("append to file? (new file:F)"=TRUE, "file path (dialog if empty)"=w2517) -> ()  [unwired: 6 in, 1 out]
                  }
                  frame #1 {
                    # "Adds Headers if they don't exist"
                    n1168 = local read "Transfer Folder"() -> (w2527:path)
                    n1169 = Concatenate Strings("Stats\\", "Tranformer Data.txt") -> (w2528:string)
                    n1170 = Build Path(base path=w2527, name or relative path=w2528) -> (appended path=w2521:path)
                    n1171 = call-poly <vilib>:"Read From Spreadsheet File.vi"("file path (dialog if empty)"=w2521) -> ("first row"=w2526:string[])  [unwired: 6 in, 4 out]
                    n1172 = Search 1D Array(1D array=w2526, element="DeviceID") -> (index of element=w2524:i32)  [unwired: 1 in]
                    n1173 = Equal?(x=w2524, y=0) -> (x = y?=w2522:bool)
                    n1174 = case shown="False" w2522 {
                      tunnel: w2521 -> [w2532 _]
                      frame False {
                        n1175 = local read "Transformer \nHeaders"() -> (w2531:string[])
                        n1176 = call-poly <vilib>:"Write To Spreadsheet File.vi"("1D data"=w2531, "file path (dialog if empty)"=w2532) -> ()  [unwired: 6 in, 1 out]
                      }
                      frame True {
                      }
                    }
                  }
                  frame #2 {
                    # "Adds current device if it doesn't exist"
                    n1177 = local read "Current \nRecord"() -> (w2537:string[])
                    n1178 = Index Array(array=w2537, index=0) -> (element=w2536:string)
                    n1179 = local read "Transfer Folder"() -> (w2540:path)
                    n1180 = Concatenate Strings("Stats\\", "Tranformer Data.txt") -> (w2541:string)
                    n1181 = local write "Current Device ID"(w2536) -> ()
                    n1182 = local read "Current Device ID"() -> (w2546:string)
                    n1183 = Build Path(base path=w2540, name or relative path=w2541) -> (appended path=w2539:path)
                    n1184 = call-poly <vilib>:"Read From Spreadsheet File.vi"("file path (dialog if empty)"=w2539) -> ("all rows"=w2533:string[][])  [unwired: 6 in, 4 out]
                    n1185 = Index Array(array=w2533, index (col)=0) -> (element=w2534:string[])  [unwired: 1 in]
                    n1186 = Search 1D Array(1D array=w2534, element=w2546) -> (index of element=w2535:i32)  [unwired: 1 in]
                    n1187 = Equal?(x=w2535, y=-1) -> (x = y?=w2548:bool)
                    n1188 = case shown="False" w2548 {
                      tunnel: w2538 -> [w2551 w2562]
                      tunnel: w2535 -> [w2554 _]
                      tunnel: w2533 -> [w2555 _]
                      frame False {
                        n1189 = local read "Current \nRecord"() -> (w2553:string[])
                        n1190 = Replace Array Subset(array=w2555, new element=w2553, index (row)=w2554) -> (w2552:string[][])  [unwired: 1 in]
                        n1191 = flat-sequence {
                          tunnel: w2551 -> [w2556]
                          tunnel: w2552 -> [w2557]
                          tunnel: [w2557] -> w2550
                          tunnel: [w2556] -> w2549
                          tunnel: w2550 -> [w2559]
                          tunnel: w2549 -> [w2558]
                          frame #0 {
                            n1192 = Delete(path (use dialog)=w2556) -> ()  [unwired: 4 in, 3 out]
                          }
                          frame #1 {
                            n1193 = call-poly <vilib>:"Write To Spreadsheet File.vi"("append to file? (new file:F)"=TRUE, "2D data"=w2559, "file path (dialog if empty)"=w2558) -> ()  [unwired: 5 in, 1 out]
                          }
                        }
                      }
                      frame True {
                        n1194 = local read "Current \nRecord"() -> (w2561:string[])
                        n1195 = call-poly <vilib>:"Write To Spreadsheet File.vi"("append to file? (new file:F)"=TRUE, "1D data"=w2561, "file path (dialog if empty)"=w2562) -> ()  [unwired: 5 in, 1 out]
                      }
                    }
                  }
                }
                n1196 = Path To String(path=w2048) -> (string=w2046:string)
                n1197 = stacked-sequence {
                  tunnel: [_ _ _ _ _ _ _ _ _ _ _ _ _ w2481] -> w2028
                  tunnel: w2027 -> [w2050 _ _ _ _ _ _ _ _ _ _ _ _ _]
                  frame #0 {
                    n1198 = call-poly <vilib>:"Read From Spreadsheet File.vi"("file path (dialog if empty)"=w2050) -> ("all rows"=w2049:string[][])  [unwired: 6 in, 4 out]
                    n1199 = Array Size(array=w2049) -> (size(s)=w2054:i32[])
                    n1200 = Array Subset(array=w2049, index (row)=0, index (col)=0, length (col)=3) -> (w2058:string[][])  [unwired: 1 in]
                    n1201 = Index Array(array=w2054, index=0) -> (element=w2052:i32)
                    n1202 = Reshape Array(w2058, w2052) -> (w2051:string[])
                    n1203 = Search 1D Array(1D array=w2051, element="Dielectric (nm):") -> (index of element=w2061:i32)  [unwired: 1 in]
                    n1204 = Equal?(x=w2061, y=-1) -> (x = y?=w2060:bool)
                    n1205 = case shown="False" w2060 {
                      tunnel: w2049 -> [w2069 w2073]
                      tunnel: w2061 -> [w2065 _]
                      tunnel: [w2064 w2073] -> w2059
                      frame False {
                        n1206 = local read "New: Dielectric"() -> (w2071:dbl)
                        n1207 = Number To Fractional String(number=w2071) -> (F-format string=w2066:string)  [unwired: 3 in]
                        n1208 = Divide(x=w2065, y=3) -> (x/y=w2068:dbl)
                        n1209 = To Word Integer(number=w2068) -> (16bit integer=w2067:i16)
                        n1210 = Replace Array Subset(array=w2069, new element=w2066, index (row)=w2067, index (col)=1) -> (w2064:string[][])
                      }
                      frame True {
                      }
                    }
                    n1211 = local write "Save1 Array"(w2059) -> ()
                  }
                  frame #1 {
                    n1212 = local read "Save1 Array"() -> (w2075:string[][])
                    n1213 = Array Size(array=w2075) -> (size(s)=w2078:i32[])
                    n1214 = Array Subset(array=w2075, index (row)=0, index (col)=0, length (col)=3) -> (w2082:string[][])  [unwired: 1 in]
                    n1215 = Index Array(array=w2078, index=0) -> (element=w2076:i32)
                    n1216 = Reshape Array(w2082, w2076) -> (w2074:string[])
                    n1217 = Search 1D Array(1D array=w2074, element="Comments:") -> (index of element=w2085:i32)  [unwired: 1 in]
                    n1218 = Equal?(x=w2085, y=-1) -> (x = y?=w2084:bool)
                    n1219 = case shown="False" w2084 {
                      tunnel: w2075 -> [w2093 w2096]
                      tunnel: w2085 -> [w2090 _]
                      tunnel: [w2089 w2096] -> w2083
                      frame False {
                        n1220 = local read "Comments:"() -> (w2088:string)
                        n1221 = Divide(x=w2090, y=3) -> (x/y=w2092:dbl)
                        n1222 = To Word Integer(number=w2092) -> (16bit integer=w2091:i16)
                        n1223 = Replace Array Subset(array=w2093, new element=w2088, index (row)=w2091, index (col)=1) -> (w2089:string[][])
                      }
                      frame True {
                      }
                    }
                    n1224 = local write "Save1 Array"(w2083) -> ()
                  }
                  frame #2 {
                    n1225 = local read "Save1 Array"() -> (w2098:string[][])
                    n1226 = Array Size(array=w2098) -> (size(s)=w2101:i32[])
                    n1227 = Array Subset(array=w2098, index (row)=0, index (col)=0, length (col)=3) -> (w2105:string[][])  [unwired: 1 in]
                    n1228 = Index Array(array=w2101, index=0) -> (element=w2099:i32)
                    n1229 = Reshape Array(w2105, w2099) -> (w2097:string[])
                    n1230 = Search 1D Array(1D array=w2097, element="Length (um):") -> (index of element=w2108:i32)  [unwired: 1 in]
                    n1231 = Equal?(x=w2108, y=-1) -> (x = y?=w2107:bool)
                    n1232 = case shown="False" w2107 {
                      tunnel: w2098 -> [w2118 w2121]
                      tunnel: w2108 -> [w2115 _]
                      tunnel: [w2114 w2121] -> w2106
                      frame False {
                        n1233 = local read "New: Length"() -> (w2111:dbl)
                        n1234 = Divide(x=w2115, y=3) -> (x/y=w2117:dbl)
                        n1235 = Format Value(format string="%#g", value (0)=w2111) -> (output string=w2112:string)  [unwired: 1 in]
                        n1236 = To Word Integer(number=w2117) -> (16bit integer=w2116:i16)
                        n1237 = Replace Array Subset(array=w2118, new element=w2112, index (row)=w2116, index (col)=1) -> (w2114:string[][])
                      }
                      frame True {
                      }
                    }
                    n1238 = local write "Save1 Array"(w2106) -> ()
                  }
                  frame #3 {
                    n1239 = local read "Save1 Array"() -> (w2123:string[][])
                    n1240 = Array Size(array=w2123) -> (size(s)=w2128:i32[])
                    n1241 = Array Subset(array=w2123, index (row)=0, index (col)=0, length (col)=3) -> (w2124:string[][])  [unwired: 1 in]
                    n1242 = Index Array(array=w2128, index=0) -> (element=w2130:i32)
                    n1243 = Reshape Array(w2124, w2130) -> (w2122:string[])
                    n1244 = Search 1D Array(1D array=w2122, element="Width (um):") -> (index of element=w2133:i32)  [unwired: 1 in]
                    n1245 = Equal?(x=w2133, y=-1) -> (x = y?=w2132:bool)
                    n1246 = case shown="False" w2132 {
                      tunnel: w2133 -> [w2141 _]
                      tunnel: w2123 -> [w2140 w2146]
                      tunnel: [w2139 w2146] -> w2131
                      frame False {
                        n1247 = local read "New: Width"() -> (w2136:dbl)
                        n1248 = Divide(x=w2141, y=3) -> (x/y=w2143:dbl)
                        n1249 = To Word Integer(number=w2143) -> (16bit integer=w2142:i16)
                        n1250 = Format Value(format string="%#g", value (0)=w2136) -> (output string=w2137:string)  [unwired: 1 in]
                        n1251 = Replace Array Subset(array=w2140, new element=w2137, index (row)=w2142, index (col)=1) -> (w2139:string[][])
                      }
                      frame True {
                      }
                    }
                    n1252 = local write "Save1 Array"(w2131) -> ()
                  }
                  frame #4 {
                    w2156 = "Sample Temp (K):"
                    n1253 = local read "Save1 Array"() -> (w2148:string[][])
                    n1254 = Array Size(array=w2148) -> (size(s)=w2153:i32[])
                    n1255 = Array Subset(array=w2148, index (row)=0, index (col)=0, length (col)=3) -> (w2149:string[][])  [unwired: 1 in]
                    n1256 = Index Array(array=w2153, index=0) -> (element=w2155:i32)
                    n1257 = Reshape Array(w2149, w2155) -> (w2147:string[])
                    n1258 = Search 1D Array(1D array=w2147, element=w2156) -> (index of element=w2159:i32)  [unwired: 1 in]
                    n1259 = Equal?(x=w2159, y=-1) -> (x = y?=w2158:bool)
                    n1260 = case shown="True" w2158 {
                      tunnel: w2148 -> [w2168 w2182]
                      tunnel: w2159 -> [w2165 _]
                      tunnel: [w2164 w2181] -> w2157
                      tunnel: w2147 -> [_ w2184]
                      tunnel: w2156 -> [_ w2171]
                      frame False {
                        n1261 = local read "New: Temp"() -> (w2162:dbl)
                        n1262 = Divide(x=w2165, y=3) -> (x/y=w2167:dbl)
                        n1263 = Format Value(format string="%#g", value (0)=w2162) -> (output string=w2161:string)  [unwired: 1 in]
                        n1264 = To Word Integer(number=w2167) -> (16bit integer=w2166:i16)
                        n1265 = Replace Array Subset(array=w2168, new element=w2161, index (row)=w2166, index (col)=1) -> (w2164:string[][])
                      }
                      frame True {
                        n1266 = local read "New: Temp"() -> (w2173:dbl)
                        n1267 = Search 1D Array(1D array=w2184, element="Width (um):") -> (index of element=w2178:i32)  [unwired: 1 in]
                        n1268 = Divide(x=w2178, y=3) -> (x/y=w2179:dbl)
                        n1269 = To Word Integer(number=w2179) -> (16bit integer=w2177:i16)
                        n1270 = Format Value(format string="%#g", value (0)=w2173) -> (output string=w2172:string)  [unwired: 1 in]
                        n1271 = Build Array(w2171, w2172) -> (w2175:string[])
                        n1272 = Increment(x=w2177) -> (x+1=w2176:i16)
                        n1273 = Insert Into Array(array=w2182, index (row)=w2176, new element=w2175) -> (w2181:string[][])  [unwired: 1 in]
                      }
                    }
                    n1274 = local write "Save1 Array"(w2157) -> ()
                  }
                  frame #5 {
                    w2194 = "Mobility-Sat (cm^2/Vs):"
                    n1275 = local read "Save1 Array"() -> (w2186:string[][])
                    n1276 = Array Size(array=w2186) -> (size(s)=w2191:i32[])
                    n1277 = Array Subset(array=w2186, index (row)=0, index (col)=0, length (col)=3) -> (w2187:string[][])  [unwired: 1 in]
                    n1278 = Index Array(array=w2191, index=0) -> (element=w2193:i32)
                    n1279 = Reshape Array(w2187, w2193) -> (w2185:string[])
                    n1280 = Search 1D Array(1D array=w2185, element=w2194) -> (index of element=w2197:i32)  [unwired: 1 in]
                    n1281 = Equal?(x=w2197, y=-1) -> (x = y?=w2196:bool)
                    n1282 = case shown="True" w2196 {
                      tunnel: w2186 -> [w2206 w2214]
                      tunnel: w2197 -> [w2203 _]
                      tunnel: [w2202 w2213] -> w2195
                      tunnel: w2185 -> [_ w2211]
                      tunnel: w2194 -> [_ w2209]
                      frame False {
                        n1283 = local read "New: Mobility-Sat"() -> (w2199:dbl)
                        n1284 = Divide(x=w2203, y=3) -> (x/y=w2205:dbl)
                        n1285 = To Word Integer(number=w2205) -> (16bit integer=w2204:i16)
                        n1286 = Format Value(format string="%#g", value (0)=w2199) -> (output string=w2200:string)  [unwired: 1 in]
                        n1287 = Replace Array Subset(array=w2206, new element=w2200, index (row)=w2204, index (col)=1) -> (w2202:string[][])
                      }
                      frame True {
                        n1288 = local read "New: Mobility-Sat"() -> (w2215:dbl)
                        n1289 = Search 1D Array(1D array=w2211, element="Mobility (cm^2/Vs):") -> (index of element=w2218:i32)  [unwired: 1 in]
                        n1290 = Divide(x=w2218, y=3) -> (x/y=w2219:dbl)
                        n1291 = To Word Integer(number=w2219) -> (16bit integer=w2210:i16)
                        n1292 = Format Value(format string="%#g", value (0)=w2215) -> (output string=w2212:string)  [unwired: 1 in]
                        n1293 = Build Array(w2209, w2212) -> (w2217:string[])
                        n1294 = Replace Array Subset(array=w2214, new element=w2217, index (row)=w2210) -> (w2213:string[][])  [unwired: 1 in]
                      }
                    }
                    n1295 = local write "Save1 Array"(w2195) -> ()
                  }
                  frame #6 {
                    w2231 = "Mobility-Lin (cm^2/Vs):"
                    n1296 = local read "Save1 Array"() -> (w2222:string[][])
                    n1297 = Array Size(array=w2222) -> (size(s)=w2228:i32[])
                    n1298 = Array Subset(array=w2222, index (row)=0, index (col)=0, length (col)=3) -> (w2224:string[][])  [unwired: 1 in]
                    n1299 = Index Array(array=w2228, index=0) -> (element=w2230:i32)
                    n1300 = Reshape Array(w2224, w2230) -> (w2223:string[])
                    n1301 = Search 1D Array(1D array=w2223, element=w2231) -> (index of element=w2234:i32)  [unwired: 1 in]
                    n1302 = Equal?(x=w2234, y=-1) -> (x = y?=w2233:bool)
                    n1303 = case shown="True" w2233 {
                      tunnel: w2222 -> [w2243 w2249]
                      tunnel: w2234 -> [w2240 _]
                      tunnel: [w2239 w2248] -> w2232
                      tunnel: w2223 -> [_ w2247]
                      tunnel: w2231 -> [_ w2246]
                      frame False {
                        n1304 = local read "Calc: Mobility-Lin"() -> (w2236:dbl)
                        n1305 = Divide(x=w2240, y=3) -> (x/y=w2242:dbl)
                        n1306 = To Word Integer(number=w2242) -> (16bit integer=w2241:i16)
                        n1307 = Format Value(format string="%#g", value (0)=w2236) -> (output string=w2237:string)  [unwired: 1 in]
                        n1308 = Replace Array Subset(array=w2243, new element=w2237, index (row)=w2241, index (col)=1) -> (w2239:string[][])
                      }
                      frame True {
                        n1309 = local read "Calc: Mobility-Lin"() -> (w2250:dbl)
                        n1310 = Search 1D Array(1D array=w2247, element="Mobility-Sat (cm^2/Vs):") -> (index of element=w2255:i32)  [unwired: 1 in]
                        n1311 = Divide(x=w2255, y=3) -> (x/y=w2256:dbl)
                        n1312 = To Word Integer(number=w2256) -> (16bit integer=w2254:i16)
                        n1313 = Format Value(format string="%#g", value (0)=w2250) -> (output string=w2259:string)  [unwired: 1 in]
                        n1314 = Build Array(w2246, w2259) -> (w2252:string[])
                        n1315 = Increment(x=w2254) -> (x+1=w2253:i16)
                        n1316 = Insert Into Array(array=w2249, index (row)=w2253, new element=w2252) -> (w2248:string[][])  [unwired: 1 in]
                      }
                    }
                    n1317 = local write "Save1 Array"(w2232) -> ()
                  }
                  frame #7 {
                    w2269 = "On/Off I-Sat:"
                    n1318 = local read "Save1 Array"() -> (w2260:string[][])
                    n1319 = Array Size(array=w2260) -> (size(s)=w2266:i32[])
                    n1320 = Array Subset(array=w2260, index (row)=0, index (col)=0, length (col)=3) -> (w2262:string[][])  [unwired: 1 in]
                    n1321 = Index Array(array=w2266, index=0) -> (element=w2268:i32)
                    n1322 = Reshape Array(w2262, w2268) -> (w2261:string[])
                    n1323 = Search 1D Array(1D array=w2261, element=w2269) -> (index of element=w2272:i32)  [unwired: 1 in]
                    n1324 = Equal?(x=w2272, y=-1) -> (x = y?=w2271:bool)
                    n1325 = case shown="True" w2271 {
                      tunnel: w2260 -> [w2281 w2288]
                      tunnel: w2272 -> [w2278 _]
                      tunnel: [w2277 w2289] -> w2270
                      tunnel: w2261 -> [_ w2286]
                      tunnel: w2269 -> [_ w2284]
                      frame False {
                        n1326 = local read "Calc: On/Off"() -> (w2274:dbl)
                        n1327 = Divide(x=w2278, y=3) -> (x/y=w2280:dbl)
                        n1328 = To Word Integer(number=w2280) -> (16bit integer=w2279:i16)
                        n1329 = Format Value(format string="%#g", value (0)=w2274) -> (output string=w2275:string)  [unwired: 1 in]
                        n1330 = Replace Array Subset(array=w2281, new element=w2275, index (row)=w2279, index (col)=1) -> (w2277:string[][])
                      }
                      frame True {
                        n1331 = local read "Calc: On/Off"() -> (w2290:dbl)
                        n1332 = Search 1D Array(1D array=w2286, element="On/Off Current:") -> (index of element=w2293:i32)  [unwired: 1 in]
                        n1333 = Divide(x=w2293, y=3) -> (x/y=w2294:dbl)
                        n1334 = To Word Integer(number=w2294) -> (16bit integer=w2285:i16)
                        n1335 = Format Value(format string="%#g", value (0)=w2290) -> (output string=w2287:string)  [unwired: 1 in]
                        n1336 = Build Array(w2284, w2287) -> (w2292:string[])
                        n1337 = Replace Array Subset(array=w2288, new element=w2292, index (row)=w2285) -> (w2289:string[][])  [unwired: 1 in]
                      }
                    }
                    n1338 = local write "Save1 Array"(w2270) -> ()
                  }
                  frame #8 {
                    w2306 = "Off I-Sat (A):"
                    n1339 = local read "Save1 Array"() -> (w2297:string[][])
                    n1340 = Array Size(array=w2297) -> (size(s)=w2303:i32[])
                    n1341 = Array Subset(array=w2297, index (row)=0, index (col)=0, length (col)=3) -> (w2299:string[][])  [unwired: 1 in]
                    n1342 = Index Array(array=w2303, index=0) -> (element=w2305:i32)
                    n1343 = Reshape Array(w2299, w2305) -> (w2298:string[])
                    n1344 = Search 1D Array(1D array=w2298, element=w2306) -> (index of element=w2309:i32)  [unwired: 1 in]
                    n1345 = Equal?(x=w2309, y=-1) -> (x = y?=w2308:bool)
                    n1346 = case shown="True" w2308 {
                      tunnel: w2297 -> [w2318 w2324]
                      tunnel: w2309 -> [w2315 _]
                      tunnel: [w2314 w2323] -> w2307
                      tunnel: w2298 -> [_ w2322]
                      tunnel: w2306 -> [_ w2321]
                      frame False {
                        n1347 = local read "Calc: Off I-Sat"() -> (w2313:dbl)
                        n1348 = Divide(x=w2315, y=3) -> (x/y=w2317:dbl)
                        n1349 = Format Value(format string="%#g", value (0)=w2313) -> (output string=w2311:string)  [unwired: 1 in]
                        n1350 = To Word Integer(number=w2317) -> (16bit integer=w2316:i16)
                        n1351 = Replace Array Subset(array=w2318, new element=w2311, index (row)=w2316, index (col)=1) -> (w2314:string[][])
                      }
                      frame True {
                        n1352 = local read "Calc: Off I-Sat"() -> (w2325:dbl)
                        n1353 = Search 1D Array(1D array=w2322, element="On/Off I-Sat:") -> (index of element=w2330:i32)  [unwired: 1 in]
                        n1354 = Divide(x=w2330, y=3) -> (x/y=w2331:dbl)
                        n1355 = To Word Integer(number=w2331) -> (16bit integer=w2329:i16)
                        n1356 = Format Value(format string="%#g", value (0)=w2325) -> (output string=w2334:string)  [unwired: 1 in]
                        n1357 = Build Array(w2321, w2334) -> (w2327:string[])
                        n1358 = Increment(x=w2329) -> (x+1=w2328:i16)
                        n1359 = Insert Into Array(array=w2324, index (row)=w2328, new element=w2327) -> (w2323:string[][])  [unwired: 1 in]
                      }
                    }
                    n1360 = local write "Save1 Array"(w2307) -> ()
                  }
                  frame #9 {
                    w2336 = "Vt-Sat (V):"
                    n1361 = local read "Save1 Array"() -> (w2337:string[][])
                    n1362 = Array Size(array=w2337) -> (size(s)=w2342:i32[])
                    n1363 = Array Subset(array=w2337, index (row)=0, index (col)=0, length (col)=3) -> (w2338:string[][])  [unwired: 1 in]
                    n1364 = Index Array(array=w2342, index=0) -> (element=w2344:i32)
                    n1365 = Reshape Array(w2338, w2344) -> (w2335:string[])
                    n1366 = Search 1D Array(1D array=w2335, element=w2336) -> (index of element=w2347:i32)  [unwired: 1 in]
                    n1367 = Equal?(x=w2347, y=-1) -> (x = y?=w2346:bool)
                    n1368 = case shown="True" w2346 {
                      tunnel: w2337 -> [w2354 w2363]
                      tunnel: w2347 -> [w2350 _]
                      tunnel: [w2349 w2362] -> w2345
                      tunnel: w2336 -> [_ w2361]
                      tunnel: w2335 -> [_ w2360]
                      frame False {
                        n1369 = local read "New: VT-Sat"() -> (w2356:dbl)
                        n1370 = Number To Fractional String(number=w2356) -> (F-format string=w2351:string)  [unwired: 3 in]
                        n1371 = Divide(x=w2350, y=3) -> (x/y=w2353:dbl)
                        n1372 = To Word Integer(number=w2353) -> (16bit integer=w2352:i16)
                        n1373 = Replace Array Subset(array=w2354, new element=w2351, index (row)=w2352, index (col)=1) -> (w2349:string[][])
                      }
                      frame True {
                        n1374 = local read "New: VT-Sat"() -> (w2364:dbl)
                        n1375 = Search 1D Array(1D array=w2360, element="Threshold V (V):") -> (index of element=w2359:i32)  [unwired: 1 in]
                        n1376 = Divide(x=w2359, y=3) -> (x/y=w2367:dbl)
                        n1377 = To Word Integer(number=w2367) -> (16bit integer=w2358:i16)
                        n1378 = Format Value(format string="%#g", value (0)=w2364) -> (output string=w2370:string)  [unwired: 1 in]
                        n1379 = Build Array(w2361, w2370) -> (w2366:string[])
                        n1380 = Replace Array Subset(array=w2363, new element=w2366, index (row)=w2358) -> (w2362:string[][])  [unwired: 1 in]
                      }
                    }
                    n1381 = local write "Save1 Array"(w2345) -> ()
                  }
                  frame #10 {
                    n1382 = local read "Save1 Array"() -> (w2371:string[][])
                    n1383 = Array Size(array=w2371) -> (size(s)=w2377:i32[])
                    n1384 = Array Subset(array=w2371, index (row)=0, index (col)=0, length (col)=3) -> (w2373:string[][])  [unwired: 1 in]
                    n1385 = Index Array(array=w2377, index=0) -> (element=w2379:i32)
                    n1386 = Reshape Array(w2373, w2379) -> (w2372:string[])
                    n1387 = Search 1D Array(1D array=w2372, element="VT-Lin (V):") -> (index of element=w2382:i32)  [unwired: 1 in]
                    n1388 = Equal?(x=w2382, y=-1) -> (x = y?=w2381:bool)
                    n1389 = case shown="False" w2381 {
                      tunnel: w2371 -> [w2392 w2395]
                      tunnel: w2382 -> [w2389 _]
                      tunnel: [w2388 w2395] -> w2380
                      frame False {
                        n1390 = local read "New: VT-Lin"() -> (w2386:dbl)
                        n1391 = Divide(x=w2389, y=3) -> (x/y=w2391:dbl)
                        n1392 = Format Value(format string="%#g", value (0)=w2386) -> (output string=w2385:string)  [unwired: 1 in]
                        n1393 = To Word Integer(number=w2391) -> (16bit integer=w2390:i16)
                        n1394 = Replace Array Subset(array=w2392, new element=w2385, index (row)=w2390, index (col)=1) -> (w2388:string[][])
                      }
                      frame True {
                      }
                    }
                    n1395 = local write "Save1 Array"(w2380) -> ()
                  }
                  frame #11 {
                    w2396 = "STS-Sat (V/decade):"
                    n1396 = local read "Save1 Array"() -> (w2398:string[][])
                    n1397 = Array Size(array=w2398) -> (size(s)=w2403:i32[])
                    n1398 = Array Subset(array=w2398, index (row)=0, index (col)=0, length (col)=3) -> (w2399:string[][])  [unwired: 1 in]
                    n1399 = Index Array(array=w2403, index=0) -> (element=w2405:i32)
                    n1400 = Reshape Array(w2399, w2405) -> (w2397:string[])
                    n1401 = Search 1D Array(1D array=w2397, element=w2396) -> (index of element=w2408:i32)  [unwired: 1 in]
                    n1402 = Equal?(x=w2408, y=-1) -> (x = y?=w2407:bool)
                    n1403 = case shown="True" w2407 {
                      tunnel: w2398 -> [w2417 w2423]
                      tunnel: w2408 -> [w2414 _]
                      tunnel: [w2413 w2424] -> w2406
                      tunnel: w2397 -> [_ w2422]
                      tunnel: w2396 -> [_ w2421]
                      frame False {
                        n1404 = local read "New: STS"() -> (w2411:dbl)
                        n1405 = Divide(x=w2414, y=3) -> (x/y=w2416:dbl)
                        n1406 = Format Value(format string="%#g", value (0)=w2411) -> (output string=w2410:string)  [unwired: 1 in]
                        n1407 = To Word Integer(number=w2416) -> (16bit integer=w2415:i16)
                        n1408 = Replace Array Subset(array=w2417, new element=w2410, index (row)=w2415, index (col)=1) -> (w2413:string[][])
                      }
                      frame True {
                        n1409 = local read "New: STS"() -> (w2425:dbl)
                        n1410 = Search 1D Array(1D array=w2422, element="S.T.S. (V/decade):") -> (index of element=w2428:i32)  [unwired: 1 in]
                        n1411 = Divide(x=w2428, y=3) -> (x/y=w2429:dbl)
                        n1412 = To Word Integer(number=w2429) -> (16bit integer=w2420:i16)
                        n1413 = Format Value(format string="%#g", value (0)=w2425) -> (output string=w2432:string)  [unwired: 1 in]
                        n1414 = Build Array(w2421, w2432) -> (w2427:string[])
                        n1415 = Replace Array Subset(array=w2423, new element=w2427, index (row)=w2420) -> (w2424:string[][])  [unwired: 1 in]
                      }
                    }
                    n1416 = local write "Save1 Array"(w2406) -> ()
                  }
                  frame #12 {
                    w2433 = "Trap Density-VT (Traps/Vcm^2):"
                    n1417 = local read "Save1 Array"() -> (w2435:string[][])
                    n1418 = Array Size(array=w2435) -> (size(s)=w2440:i32[])
                    n1419 = Array Subset(array=w2435, index (row)=0, index (col)=0, length (col)=3) -> (w2436:string[][])  [unwired: 1 in]
                    n1420 = Index Array(array=w2440, index=0) -> (element=w2442:i32)
                    n1421 = Reshape Array(w2436, w2442) -> (w2434:string[])
                    n1422 = Search 1D Array(1D array=w2434, element=w2433) -> (index of element=w2445:i32)  [unwired: 1 in]
                    n1423 = Equal?(x=w2445, y=-1) -> (x = y?=w2444:bool)
                    n1424 = case shown="True" w2444 {
                      tunnel: w2435 -> [w2454 w2459]
                      tunnel: w2445 -> [w2450 _]
                      tunnel: [w2449 w2460] -> w2443
                      tunnel: w2434 -> [_ w2458]
                      tunnel: w2433 -> [_ w2457]
                      frame False {
                        n1425 = local read "New: Trap Density-VT"() -> (w2448:dbl)
                        n1426 = Format Value(format string="%#g", value (0)=w2448) -> (output string=w2451:string)  [unwired: 1 in]
                        n1427 = Divide(x=w2450, y=3) -> (x/y=w2453:dbl)
                        n1428 = To Word Integer(number=w2453) -> (16bit integer=w2452:i16)
                        n1429 = Replace Array Subset(array=w2454, new element=w2451, index (row)=w2452, index (col)=1) -> (w2449:string[][])
                      }
                      frame True {
                        n1430 = local read "New: Trap Density-VT"() -> (w2470:dbl)
                        n1431 = Search 1D Array(1D array=w2458, element="STS-Sat (V/decade):") -> (index of element=w2465:i32)  [unwired: 1 in]
                        n1432 = Divide(x=w2465, y=3) -> (x/y=w2464:dbl)
                        n1433 = To Word Integer(number=w2464) -> (16bit integer=w2466:i16)
                        n1434 = Format Value(format string="%#g", value (0)=w2470) -> (output string=w2461:string)  [unwired: 1 in]
                        n1435 = Build Array(w2457, w2461) -> (w2468:string[])
                        n1436 = Increment(x=w2466) -> (x+1=w2467:i16)
                        n1437 = Insert Into Array(array=w2459, index (row)=w2467, new element=w2468) -> (w2460:string[][])  [unwired: 1 in]
                      }
                    }
                    n1438 = local write "Save1 Array"(w2443) -> ()
                  }
                  frame #13 {
                    w2471 = "Trap Density-STS (Traps/Vcm^2):"
                    n1439 = local read "Save1 Array"() -> (w2473:string[][])
                    n1440 = Array Size(array=w2473) -> (size(s)=w2478:i32[])
                    n1441 = Array Subset(array=w2473, index (row)=0, index (col)=0, length (col)=3) -> (w2474:string[][])  [unwired: 1 in]
                    n1442 = Index Array(array=w2478, index=0) -> (element=w2480:i32)
                    n1443 = Reshape Array(w2474, w2480) -> (w2472:string[])
                    n1444 = Search 1D Array(1D array=w2472, element=w2471) -> (index of element=w2483:i32)  [unwired: 1 in]
                    n1445 = Equal?(x=w2483, y=-1) -> (x = y?=w2482:bool)
                    n1446 = case shown="True" w2482 {
                      tunnel: w2473 -> [w2492 w2497]
                      tunnel: w2483 -> [w2489 _]
                      tunnel: [w2488 w2498] -> w2481
                      tunnel: w2472 -> [_ w2496]
                      tunnel: w2471 -> [_ w2495]
                      frame False {
                        n1447 = local read "New: Trap Density-STS"() -> (w2486:dbl)
                        n1448 = Divide(x=w2489, y=3) -> (x/y=w2491:dbl)
                        n1449 = To Word Integer(number=w2491) -> (16bit integer=w2490:i16)
                        n1450 = Format Value(format string="%#g", value (0)=w2486) -> (output string=w2485:string)  [unwired: 1 in]
                        n1451 = Replace Array Subset(array=w2492, new element=w2485, index (row)=w2490, index (col)=1) -> (w2488:string[][])
                      }
                      frame True {
                        n1452 = local read "New: Trap Density-STS"() -> (w2499:dbl)
                        n1453 = Search 1D Array(1D array=w2496, element="Trap Density-VT (Traps/Vcm^2):") -> (index of element=w2504:i32)  [unwired: 1 in]
                        n1454 = Divide(x=w2504, y=3) -> (x/y=w2505:dbl)
                        n1455 = To Word Integer(number=w2505) -> (16bit integer=w2503:i16)
                        n1456 = Format Value(format string="%#g", value (0)=w2499) -> (output string=w2508:string)  [unwired: 1 in]
                        n1457 = Build Array(w2495, w2508) -> (w2501:string[])
                        n1458 = Increment(x=w2503) -> (x+1=w2502:i16)
                        n1459 = Insert Into Array(array=w2497, index (row)=w2502, new element=w2501) -> (w2498:string[][])  [unwired: 1 in]
                      }
                    }
                    n1460 = local write "Save1 Array"(w2481) -> ()
                  }
                }
                n1461 = Concatenate Strings(w2046, "\\", w2044) -> (w2045:string)
                n1462 = String To Path(string=w2045) -> (path=w2035:path)
                n1463 = disable-structure shown="Disabled" {
                  frame Disabled {
                  }
                  frame Enabled {
                  }
                }
              }
              frame #2 {
                n1464 = Equal?(x=w2567, y=w2564) -> (x = y?=w2566:bool)
                n1465 = case shown="False" w2566 {
                  tunnel: w2567 -> [w2570 _]
                  tunnel: w2564 -> [w2569 _]
                  frame False {
                    n1466 = Move(source path=w2570, 9:TRUE, 10:w2569) -> ()  [unwired: 2 in, 3 out]
                  }
                  frame True {
                  }
                }
              }
              frame #3 {
                n1467 = local write "Transfer File"(w2571) -> ()
                n1468 = call-poly <vilib>:"Write To Spreadsheet File.vi"("2D data"=w2572, "file path (dialog if empty)"=w2571) -> ()  [unwired: 6 in, 1 out]
              }
            }
          }
          event "Save Changes? 2": Mouse Down {
            n1469 = event-data() -> ()  [unwired: 1 in, 5 out]
            n1470 = stacked-sequence {
              seq-local: [w2630 _ _ _ _] -> [_ w3113 _ _ _]
              seq-local: [w2629 _ _ _ _] -> [_ w3114 _ _ _]
              seq-local: [w2629 _ _ _ _] -> [_ w3112 _ _ _]
              seq-local: [w2631 _ _ _ _] -> [_ w3110 _ _ _]
              seq-local: [_ w3114 _ _ _] -> [_ _ w3119 _ _]
              seq-local: [_ w3110 _ _ _] -> [_ _ w3118 _ _]
              frame #0 {
                n1471 = local read "Transfer File"() -> (w2630:path)
                n1472 = local read "New: Temp"() -> (w2633:dbl)
                n1473 = local read "New: Length"() -> (w2636:dbl)
                n1474 = local read "New: Width"() -> (w2634:dbl)
                n1475 = To Word Integer(number=w2633) -> (16bit integer=w2632:i16)
                n1476 = Number To Decimal String(number=w2632) -> (decimal integer string=w2640:string)  [unwired: 1 in]
                n1477 = To Single Precision Float(number=w2634) -> (single precision float=w2635:sgl)
                n1478 = To Single Precision Float(number=w2636) -> (single precision float=w2637:sgl)
                n1479 = local read "Index"() -> (w2644:string)
                n1480 = Strip Path(path=w2630) -> (stripped path=w2649:path)  [unwired: 1 out]
                n1481 = Number To Decimal String(number=w2637) -> (decimal integer string=w2642:string)  [unwired: 1 in]
                n1482 = Number To Decimal String(number=w2635) -> (decimal integer string=w2643:string)  [unwired: 1 in]
                n1483 = Concatenate Strings("_", w2640, "K") -> (w2638:string)
                n1484 = call "Build Text2"("Temp"=w2638, "Index"=w2644, "Length"=w2642, "Width"=w2643) -> ("Result"=w2645:string)  [unwired: 10 in, 1 out]
                n1485 = Path To String(path=w2649) -> (string=w2647:string)
                n1486 = Concatenate Strings(w2647, "\\", w2645) -> (w2646:string)
                n1487 = stacked-sequence {
                  tunnel: [_ _ _ _ _ _ _ _ _ _ _ _ _ w3072] -> _
                  tunnel: w2630 -> [w2651 _ _ _ _ _ _ _ _ _ _ _ _ _]
                  tunnel: [_ _ _ _ _ _ _ _ _ _ _ _ _ w3072] -> w2631
                  frame #0 {
                    n1488 = call-poly <vilib>:"Read From Spreadsheet File.vi"("file path (dialog if empty)"=w2651) -> ("all rows"=w2650:string[][])  [unwired: 6 in, 4 out]
                    n1489 = Array Size(array=w2650) -> (size(s)=w2655:i32[])
                    n1490 = Array Subset(array=w2650, index (row)=0, index (col)=0, length (col)=3) -> (w2659:string[][])  [unwired: 1 in]
                    n1491 = Index Array(array=w2655, index=0) -> (element=w2653:i32)
                    n1492 = Reshape Array(w2659, w2653) -> (w2652:string[])
                    n1493 = Search 1D Array(1D array=w2652, element="Dielectric (nm):") -> (index of element=w2662:i32)  [unwired: 1 in]
                    n1494 = Equal?(x=w2662, y=-1) -> (x = y?=w2661:bool)
                    n1495 = case shown="False" w2661 {
                      tunnel: w2650 -> [w2670 w2674]
                      tunnel: w2662 -> [w2666 _]
                      tunnel: [w2665 w2674] -> w2660
                      frame False {
                        n1496 = local read "New: Dielectric"() -> (w2672:dbl)
                        n1497 = Number To Fractional String(number=w2672) -> (F-format string=w2667:string)  [unwired: 3 in]
                        n1498 = Divide(x=w2666, y=3) -> (x/y=w2669:dbl)
                        n1499 = To Word Integer(number=w2669) -> (16bit integer=w2668:i16)
                        n1500 = Replace Array Subset(array=w2670, new element=w2667, index (row)=w2668, index (col)=1) -> (w2665:string[][])
                      }
                      frame True {
                      }
                    }
                    n1501 = local write "Save1 Array"(w2660) -> ()
                  }
                  frame #1 {
                    n1502 = local read "Save1 Array"() -> (w2676:string[][])
                    n1503 = Array Size(array=w2676) -> (size(s)=w2679:i32[])
                    n1504 = Array Subset(array=w2676, index (row)=0, index (col)=0, length (col)=3) -> (w2683:string[][])  [unwired: 1 in]
                    n1505 = Index Array(array=w2679, index=0) -> (element=w2677:i32)
                    n1506 = Reshape Array(w2683, w2677) -> (w2675:string[])
                    n1507 = Search 1D Array(1D array=w2675, element="Comments:") -> (index of element=w2686:i32)  [unwired: 1 in]
                    n1508 = Equal?(x=w2686, y=-1) -> (x = y?=w2685:bool)
                    n1509 = case shown="False" w2685 {
                      tunnel: w2676 -> [w2694 w2697]
                      tunnel: w2686 -> [w2691 _]
                      tunnel: [w2690 w2697] -> w2684
                      frame False {
                        n1510 = local read "Comments:"() -> (w2689:string)
                        n1511 = Divide(x=w2691, y=3) -> (x/y=w2693:dbl)
                        n1512 = To Word Integer(number=w2693) -> (16bit integer=w2692:i16)
                        n1513 = Replace Array Subset(array=w2694, new element=w2689, index (row)=w2692, index (col)=1) -> (w2690:string[][])
                      }
                      frame True {
                      }
                    }
                    n1514 = local write "Save1 Array"(w2684) -> ()
                  }
                  frame #2 {
                    n1515 = local read "Save1 Array"() -> (w2699:string[][])
                    n1516 = Array Size(array=w2699) -> (size(s)=w2702:i32[])
                    n1517 = Array Subset(array=w2699, index (row)=0, index (col)=0, length (col)=3) -> (w2706:string[][])  [unwired: 1 in]
                    n1518 = Index Array(array=w2702, index=0) -> (element=w2700:i32)
                    n1519 = Reshape Array(w2706, w2700) -> (w2698:string[])
                    n1520 = Search 1D Array(1D array=w2698, element="Length (um):") -> (index of element=w2709:i32)  [unwired: 1 in]
                    n1521 = Equal?(x=w2709, y=-1) -> (x = y?=w2708:bool)
                    n1522 = case shown="False" w2708 {
                      tunnel: w2699 -> [w2719 w2722]
                      tunnel: w2709 -> [w2716 _]
                      tunnel: [w2715 w2722] -> w2707
                      frame False {
                        n1523 = local read "New: Length"() -> (w2712:dbl)
                        n1524 = Divide(x=w2716, y=3) -> (x/y=w2718:dbl)
                        n1525 = Format Value(format string="%#g", value (0)=w2712) -> (output string=w2713:string)  [unwired: 1 in]
                        n1526 = To Word Integer(number=w2718) -> (16bit integer=w2717:i16)
                        n1527 = Replace Array Subset(array=w2719, new element=w2713, index (row)=w2717, index (col)=1) -> (w2715:string[][])
                      }
                      frame True {
                      }
                    }
                    n1528 = local write "Save1 Array"(w2707) -> ()
                  }
                  frame #3 {
                    n1529 = local read "Save1 Array"() -> (w2724:string[][])
                    n1530 = Array Size(array=w2724) -> (size(s)=w2729:i32[])
                    n1531 = Array Subset(array=w2724, index (row)=0, index (col)=0, length (col)=3) -> (w2725:string[][])  [unwired: 1 in]
                    n1532 = Index Array(array=w2729, index=0) -> (element=w2731:i32)
                    n1533 = Reshape Array(w2725, w2731) -> (w2723:string[])
                    n1534 = Search 1D Array(1D array=w2723, element="Width (um):") -> (index of element=w2734:i32)  [unwired: 1 in]
                    n1535 = Equal?(x=w2734, y=-1) -> (x = y?=w2733:bool)
                    n1536 = case shown="False" w2733 {
                      tunnel: w2734 -> [w2742 _]
                      tunnel: w2724 -> [w2741 w2747]
                      tunnel: [w2740 w2747] -> w2732
                      frame False {
                        n1537 = local read "New: Width"() -> (w2737:dbl)
                        n1538 = Divide(x=w2742, y=3) -> (x/y=w2744:dbl)
                        n1539 = To Word Integer(number=w2744) -> (16bit integer=w2743:i16)
                        n1540 = Format Value(format string="%#g", value (0)=w2737) -> (output string=w2738:string)  [unwired: 1 in]
                        n1541 = Replace Array Subset(array=w2741, new element=w2738, index (row)=w2743, index (col)=1) -> (w2740:string[][])
                      }
                      frame True {
                      }
                    }
                    n1542 = local write "Save1 Array"(w2732) -> ()
                  }
                  frame #4 {
                    w2757 = "Sample Temp (K):"
                    n1543 = local read "Save1 Array"() -> (w2749:string[][])
                    n1544 = Array Size(array=w2749) -> (size(s)=w2754:i32[])
                    n1545 = Array Subset(array=w2749, index (row)=0, index (col)=0, length (col)=3) -> (w2750:string[][])  [unwired: 1 in]
                    n1546 = Index Array(array=w2754, index=0) -> (element=w2756:i32)
                    n1547 = Reshape Array(w2750, w2756) -> (w2748:string[])
                    n1548 = Search 1D Array(1D array=w2748, element=w2757) -> (index of element=w2760:i32)  [unwired: 1 in]
                    n1549 = Equal?(x=w2760, y=-1) -> (x = y?=w2759:bool)
                    n1550 = case shown="True" w2759 {
                      tunnel: w2749 -> [w2769 w2783]
                      tunnel: w2760 -> [w2766 _]
                      tunnel: [w2765 w2782] -> w2758
                      tunnel: w2748 -> [_ w2785]
                      tunnel: w2757 -> [_ w2772]
                      frame False {
                        n1551 = local read "New: Temp"() -> (w2763:dbl)
                        n1552 = Divide(x=w2766, y=3) -> (x/y=w2768:dbl)
                        n1553 = Format Value(format string="%#g", value (0)=w2763) -> (output string=w2762:string)  [unwired: 1 in]
                        n1554 = To Word Integer(number=w2768) -> (16bit integer=w2767:i16)
                        n1555 = Replace Array Subset(array=w2769, new element=w2762, index (row)=w2767, index (col)=1) -> (w2765:string[][])
                      }
                      frame True {
                        n1556 = local read "New: Temp"() -> (w2774:dbl)
                        n1557 = Search 1D Array(1D array=w2785, element="Width (um):") -> (index of element=w2779:i32)  [unwired: 1 in]
                        n1558 = Divide(x=w2779, y=3) -> (x/y=w2780:dbl)
                        n1559 = To Word Integer(number=w2780) -> (16bit integer=w2778:i16)
                        n1560 = Format Value(format string="%#g", value (0)=w2774) -> (output string=w2773:string)  [unwired: 1 in]
                        n1561 = Build Array(w2772, w2773) -> (w2776:string[])
                        n1562 = Increment(x=w2778) -> (x+1=w2777:i16)
                        n1563 = Insert Into Array(array=w2783, index (row)=w2777, new element=w2776) -> (w2782:string[][])  [unwired: 1 in]
                      }
                    }
                    n1564 = local write "Save1 Array"(w2758) -> ()
                  }
                  frame #5 {
                    w2795 = "Mobility-Sat (cm^2/Vs):"
                    n1565 = local read "Save1 Array"() -> (w2787:string[][])
                    n1566 = Array Size(array=w2787) -> (size(s)=w2792:i32[])
                    n1567 = Array Subset(array=w2787, index (row)=0, index (col)=0, length (col)=3) -> (w2788:string[][])  [unwired: 1 in]
                    n1568 = Index Array(array=w2792, index=0) -> (element=w2794:i32)
                    n1569 = Reshape Array(w2788, w2794) -> (w2786:string[])
                    n1570 = Search 1D Array(1D array=w2786, element=w2795) -> (index of element=w2798:i32)  [unwired: 1 in]
                    n1571 = Equal?(x=w2798, y=-1) -> (x = y?=w2797:bool)
                    n1572 = case shown="True" w2797 {
                      tunnel: w2787 -> [w2807 w2815]
                      tunnel: w2798 -> [w2804 _]
                      tunnel: [w2803 w2814] -> w2796
                      tunnel: w2786 -> [_ w2812]
                      tunnel: w2795 -> [_ w2810]
                      frame False {
                        n1573 = local read "New: Mobility-Sat"() -> (w2800:dbl)
                        n1574 = Divide(x=w2804, y=3) -> (x/y=w2806:dbl)
                        n1575 = To Word Integer(number=w2806) -> (16bit integer=w2805:i16)
                        n1576 = Format Value(format string="%#g", value (0)=w2800) -> (output string=w2801:string)  [unwired: 1 in]
                        n1577 = Replace Array Subset(array=w2807, new element=w2801, index (row)=w2805, index (col)=1) -> (w2803:string[][])
                      }
                      frame True {
                        n1578 = local read "New: Mobility-Sat"() -> (w2816:dbl)
                        n1579 = Search 1D Array(1D array=w2812, element="Mobility (cm^2/Vs):") -> (index of element=w2819:i32)  [unwired: 1 in]
                        n1580 = Divide(x=w2819, y=3) -> (x/y=w2820:dbl)
                        n1581 = To Word Integer(number=w2820) -> (16bit integer=w2811:i16)
                        n1582 = Format Value(format string="%#g", value (0)=w2816) -> (output string=w2813:string)  [unwired: 1 in]
                        n1583 = Build Array(w2810, w2813) -> (w2818:string[])
                        n1584 = Replace Array Subset(array=w2815, new element=w2818, index (row)=w2811) -> (w2814:string[][])  [unwired: 1 in]
                      }
                    }
                    n1585 = local write "Save1 Array"(w2796) -> ()
                  }
                  frame #6 {
                    w2832 = "Mobility-Lin (cm^2/Vs):"
                    n1586 = local read "Save1 Array"() -> (w2823:string[][])
                    n1587 = Array Size(array=w2823) -> (size(s)=w2829:i32[])
                    n1588 = Array Subset(array=w2823, index (row)=0, index (col)=0, length (col)=3) -> (w2825:string[][])  [unwired: 1 in]
                    n1589 = Index Array(array=w2829, index=0) -> (element=w2831:i32)
                    n1590 = Reshape Array(w2825, w2831) -> (w2824:string[])
                    n1591 = Search 1D Array(1D array=w2824, element=w2832) -> (index of element=w2835:i32)  [unwired: 1 in]
                    n1592 = Equal?(x=w2835, y=-1) -> (x = y?=w2834:bool)
                    n1593 = case shown="True" w2834 {
                      tunnel: w2823 -> [w2844 w2850]
                      tunnel: w2835 -> [w2841 _]
                      tunnel: [w2840 w2849] -> w2833
                      tunnel: w2824 -> [_ w2848]
                      tunnel: w2832 -> [_ w2847]
                      frame False {
                        n1594 = local read "Calc: Mobility-Lin"() -> (w2837:dbl)
                        n1595 = Divide(x=w2841, y=3) -> (x/y=w2843:dbl)
                        n1596 = To Word Integer(number=w2843) -> (16bit integer=w2842:i16)
                        n1597 = Format Value(format string="%#g", value (0)=w2837) -> (output string=w2838:string)  [unwired: 1 in]
                        n1598 = Replace Array Subset(array=w2844, new element=w2838, index (row)=w2842, index (col)=1) -> (w2840:string[][])
                      }
                      frame True {
                        n1599 = local read "Calc: Mobility-Lin"() -> (w2851:dbl)
                        n1600 = Search 1D Array(1D array=w2848, element="Mobility-Sat (cm^2/Vs):") -> (index of element=w2856:i32)  [unwired: 1 in]
                        n1601 = Divide(x=w2856, y=3) -> (x/y=w2857:dbl)
                        n1602 = To Word Integer(number=w2857) -> (16bit integer=w2855:i16)
                        n1603 = Format Value(format string="%#g", value (0)=w2851) -> (output string=w2860:string)  [unwired: 1 in]
                        n1604 = Build Array(w2847, w2860) -> (w2853:string[])
                        n1605 = Increment(x=w2855) -> (x+1=w2854:i16)
                        n1606 = Insert Into Array(array=w2850, index (row)=w2854, new element=w2853) -> (w2849:string[][])  [unwired: 1 in]
                      }
                    }
                    n1607 = local write "Save1 Array"(w2833) -> ()
                  }
                  frame #7 {
                    w2870 = "On/Off I-Sat:"
                    n1608 = local read "Save1 Array"() -> (w2861:string[][])
                    n1609 = Array Size(array=w2861) -> (size(s)=w2867:i32[])
                    n1610 = Array Subset(array=w2861, index (row)=0, index (col)=0, length (col)=3) -> (w2863:string[][])  [unwired: 1 in]
                    n1611 = Index Array(array=w2867, index=0) -> (element=w2869:i32)
                    n1612 = Reshape Array(w2863, w2869) -> (w2862:string[])
                    n1613 = Search 1D Array(1D array=w2862, element=w2870) -> (index of element=w2873:i32)  [unwired: 1 in]
                    n1614 = Equal?(x=w2873, y=-1) -> (x = y?=w2872:bool)
                    n1615 = case shown="True" w2872 {
                      tunnel: w2861 -> [w2882 w2889]
                      tunnel: w2873 -> [w2879 _]
                      tunnel: [w2878 w2890] -> w2871
                      tunnel: w2862 -> [_ w2887]
                      tunnel: w2870 -> [_ w2885]
                      frame False {
                        n1616 = local read "Calc: On/Off"() -> (w2875:dbl)
                        n1617 = Divide(x=w2879, y=3) -> (x/y=w2881:dbl)
                        n1618 = To Word Integer(number=w2881) -> (16bit integer=w2880:i16)
                        n1619 = Format Value(format string="%#g", value (0)=w2875) -> (output string=w2876:string)  [unwired: 1 in]
                        n1620 = Replace Array Subset(array=w2882, new element=w2876, index (row)=w2880, index (col)=1) -> (w2878:string[][])
                      }
                      frame True {
                        n1621 = local read "Calc: On/Off"() -> (w2891:dbl)
                        n1622 = Search 1D Array(1D array=w2887, element="On/Off Current:") -> (index of element=w2894:i32)  [unwired: 1 in]
                        n1623 = Divide(x=w2894, y=3) -> (x/y=w2895:dbl)
                        n1624 = To Word Integer(number=w2895) -> (16bit integer=w2886:i16)
                        n1625 = Format Value(format string="%#g", value (0)=w2891) -> (output string=w2888:string)  [unwired: 1 in]
                        n1626 = Build Array(w2885, w2888) -> (w2893:string[])
                        n1627 = Replace Array Subset(array=w2889, new element=w2893, index (row)=w2886) -> (w2890:string[][])  [unwired: 1 in]
                      }
                    }
                    n1628 = local write "Save1 Array"(w2871) -> ()
                  }
                  frame #8 {
                    w2907 = "Off I-Sat (A):"
                    n1629 = local read "Save1 Array"() -> (w2898:string[][])
                    n1630 = Array Size(array=w2898) -> (size(s)=w2904:i32[])
                    n1631 = Array Subset(array=w2898, index (row)=0, index (col)=0, length (col)=3) -> (w2900:string[][])  [unwired: 1 in]
                    n1632 = Index Array(array=w2904, index=0) -> (element=w2906:i32)
                    n1633 = Reshape Array(w2900, w2906) -> (w2899:string[])
                    n1634 = Search 1D Array(1D array=w2899, element=w2907) -> (index of element=w2910:i32)  [unwired: 1 in]
                    n1635 = Equal?(x=w2910, y=-1) -> (x = y?=w2909:bool)
                    n1636 = case shown="True" w2909 {
                      tunnel: w2898 -> [w2919 w2925]
                      tunnel: w2910 -> [w2916 _]
                      tunnel: [w2915 w2924] -> w2908
                      tunnel: w2899 -> [_ w2923]
                      tunnel: w2907 -> [_ w2922]
                      frame False {
                        n1637 = local read "Calc: Off I-Sat"() -> (w2914:dbl)
                        n1638 = Divide(x=w2916, y=3) -> (x/y=w2918:dbl)
                        n1639 = Format Value(format string="%#g", value (0)=w2914) -> (output string=w2912:string)  [unwired: 1 in]
                        n1640 = To Word Integer(number=w2918) -> (16bit integer=w2917:i16)
                        n1641 = Replace Array Subset(array=w2919, new element=w2912, index (row)=w2917, index (col)=1) -> (w2915:string[][])
                      }
                      frame True {
                        n1642 = local read "Calc: Off I-Sat"() -> (w2926:dbl)
                        n1643 = Search 1D Array(1D array=w2923, element="On/Off I-Sat:") -> (index of element=w2931:i32)  [unwired: 1 in]
                        n1644 = Divide(x=w2931, y=3) -> (x/y=w2932:dbl)
                        n1645 = To Word Integer(number=w2932) -> (16bit integer=w2930:i16)
                        n1646 = Format Value(format string="%#g", value (0)=w2926) -> (output string=w2935:string)  [unwired: 1 in]
                        n1647 = Build Array(w2922, w2935) -> (w2928:string[])
                        n1648 = Increment(x=w2930) -> (x+1=w2929:i16)
                        n1649 = Insert Into Array(array=w2925, index (row)=w2929, new element=w2928) -> (w2924:string[][])  [unwired: 1 in]
                      }
                    }
                    n1650 = local write "Save1 Array"(w2908) -> ()
                  }
                  frame #9 {
                    w2937 = "Vt-Sat (V):"
                    n1651 = local read "Save1 Array"() -> (w2938:string[][])
                    n1652 = Array Size(array=w2938) -> (size(s)=w2943:i32[])
                    n1653 = Array Subset(array=w2938, index (row)=0, index (col)=0, length (col)=3) -> (w2939:string[][])  [unwired: 1 in]
                    n1654 = Index Array(array=w2943, index=0) -> (element=w2945:i32)
                    n1655 = Reshape Array(w2939, w2945) -> (w2936:string[])
                    n1656 = Search 1D Array(1D array=w2936, element=w2937) -> (index of element=w2948:i32)  [unwired: 1 in]
                    n1657 = Equal?(x=w2948, y=-1) -> (x = y?=w2947:bool)
                    n1658 = case shown="True" w2947 {
                      tunnel: w2938 -> [w2955 w2964]
                      tunnel: w2948 -> [w2951 _]
                      tunnel: [w2950 w2963] -> w2946
                      tunnel: w2937 -> [_ w2962]
                      tunnel: w2936 -> [_ w2961]
                      frame False {
                        n1659 = local read "New: VT-Sat"() -> (w2957:dbl)
                        n1660 = Number To Fractional String(number=w2957) -> (F-format string=w2952:string)  [unwired: 3 in]
                        n1661 = Divide(x=w2951, y=3) -> (x/y=w2954:dbl)
                        n1662 = To Word Integer(number=w2954) -> (16bit integer=w2953:i16)
                        n1663 = Replace Array Subset(array=w2955, new element=w2952, index (row)=w2953, index (col)=1) -> (w2950:string[][])
                      }
                      frame True {
                        n1664 = local read "New: VT-Sat"() -> (w2965:dbl)
                        n1665 = Search 1D Array(1D array=w2961, element="Threshold V (V):") -> (index of element=w2960:i32)  [unwired: 1 in]
                        n1666 = Divide(x=w2960, y=3) -> (x/y=w2968:dbl)
                        n1667 = To Word Integer(number=w2968) -> (16bit integer=w2959:i16)
                        n1668 = Format Value(format string="%#g", value (0)=w2965) -> (output string=w2971:string)  [unwired: 1 in]
                        n1669 = Build Array(w2962, w2971) -> (w2967:string[])
                        n1670 = Replace Array Subset(array=w2964, new element=w2967, index (row)=w2959) -> (w2963:string[][])  [unwired: 1 in]
                      }
                    }
                    n1671 = local write "Save1 Array"(w2946) -> ()
                  }
                  frame #10 {
                    n1672 = local read "Save1 Array"() -> (w2972:string[][])
                    n1673 = Array Size(array=w2972) -> (size(s)=w2978:i32[])
                    n1674 = Array Subset(array=w2972, index (row)=0, index (col)=0, length (col)=3) -> (w2974:string[][])  [unwired: 1 in]
                    n1675 = Index Array(array=w2978, index=0) -> (element=w2980:i32)
                    n1676 = Reshape Array(w2974, w2980) -> (w2973:string[])
                    n1677 = Search 1D Array(1D array=w2973, element="VT-Lin (V):") -> (index of element=w2983:i32)  [unwired: 1 in]
                    n1678 = Equal?(x=w2983, y=-1) -> (x = y?=w2982:bool)
                    n1679 = case shown="False" w2982 {
                      tunnel: w2972 -> [w2993 w2996]
                      tunnel: w2983 -> [w2990 _]
                      tunnel: [w2989 w2996] -> w2981
                      frame False {
                        n1680 = local read "New: VT-Lin"() -> (w2987:dbl)
                        n1681 = Divide(x=w2990, y=3) -> (x/y=w2992:dbl)
                        n1682 = Format Value(format string="%#g", value (0)=w2987) -> (output string=w2986:string)  [unwired: 1 in]
                        n1683 = To Word Integer(number=w2992) -> (16bit integer=w2991:i16)
                        n1684 = Replace Array Subset(array=w2993, new element=w2986, index (row)=w2991, index (col)=1) -> (w2989:string[][])
                      }
                      frame True {
                      }
                    }
                    n1685 = local write "Save1 Array"(w2981) -> ()
                  }
                  frame #11 {
                    w2997 = "STS-Sat (V/decade):"
                    n1686 = local read "Save1 Array"() -> (w2999:string[][])
                    n1687 = Array Size(array=w2999) -> (size(s)=w3004:i32[])
                    n1688 = Array Subset(array=w2999, index (row)=0, index (col)=0, length (col)=3) -> (w3000:string[][])  [unwired: 1 in]
                    n1689 = Index Array(array=w3004, index=0) -> (element=w3006:i32)
                    n1690 = Reshape Array(w3000, w3006) -> (w2998:string[])
                    n1691 = Search 1D Array(1D array=w2998, element=w2997) -> (index of element=w3009:i32)  [unwired: 1 in]
                    n1692 = Equal?(x=w3009, y=-1) -> (x = y?=w3008:bool)
                    n1693 = case shown="True" w3008 {
                      tunnel: w2999 -> [w3018 w3024]
                      tunnel: w3009 -> [w3015 _]
                      tunnel: [w3014 w3025] -> w3007
                      tunnel: w2998 -> [_ w3023]
                      tunnel: w2997 -> [_ w3022]
                      frame False {
                        n1694 = local read "New: STS"() -> (w3012:dbl)
                        n1695 = Divide(x=w3015, y=3) -> (x/y=w3017:dbl)
                        n1696 = Format Value(format string="%#g", value (0)=w3012) -> (output string=w3011:string)  [unwired: 1 in]
                        n1697 = To Word Integer(number=w3017) -> (16bit integer=w3016:i16)
                        n1698 = Replace Array Subset(array=w3018, new element=w3011, index (row)=w3016, index (col)=1) -> (w3014:string[][])
                      }
                      frame True {
                        n1699 = local read "New: STS"() -> (w3026:dbl)
                        n1700 = Search 1D Array(1D array=w3023, element="S.T.S. (V/decade):") -> (index of element=w3029:i32)  [unwired: 1 in]
                        n1701 = Divide(x=w3029, y=3) -> (x/y=w3030:dbl)
                        n1702 = To Word Integer(number=w3030) -> (16bit integer=w3021:i16)
                        n1703 = Format Value(format string="%#g", value (0)=w3026) -> (output string=w3033:string)  [unwired: 1 in]
                        n1704 = Build Array(w3022, w3033) -> (w3028:string[])
                        n1705 = Replace Array Subset(array=w3024, new element=w3028, index (row)=w3021) -> (w3025:string[][])  [unwired: 1 in]
                      }
                    }
                    n1706 = local write "Save1 Array"(w3007) -> ()
                  }
                  frame #12 {
                    w3034 = "Trap Density-VT (Traps/Vcm^2):"
                    n1707 = local read "Save1 Array"() -> (w3036:string[][])
                    n1708 = Array Size(array=w3036) -> (size(s)=w3041:i32[])
                    n1709 = Array Subset(array=w3036, index (row)=0, index (col)=0, length (col)=3) -> (w3037:string[][])  [unwired: 1 in]
                    n1710 = Index Array(array=w3041, index=0) -> (element=w3043:i32)
                    n1711 = Reshape Array(w3037, w3043) -> (w3035:string[])
                    n1712 = Search 1D Array(1D array=w3035, element=w3034) -> (index of element=w3046:i32)  [unwired: 1 in]
                    n1713 = Equal?(x=w3046, y=-1) -> (x = y?=w3045:bool)
                    n1714 = case shown="True" w3045 {
                      tunnel: w3036 -> [w3055 w3060]
                      tunnel: w3046 -> [w3051 _]
                      tunnel: [w3050 w3061] -> w3044
                      tunnel: w3035 -> [_ w3059]
                      tunnel: w3034 -> [_ w3058]
                      frame False {
                        n1715 = local read "New: Trap Density-VT"() -> (w3049:dbl)
                        n1716 = Format Value(format string="%#g", value (0)=w3049) -> (output string=w3052:string)  [unwired: 1 in]
                        n1717 = Divide(x=w3051, y=3) -> (x/y=w3054:dbl)
                        n1718 = To Word Integer(number=w3054) -> (16bit integer=w3053:i16)
                        n1719 = Replace Array Subset(array=w3055, new element=w3052, index (row)=w3053, index (col)=1) -> (w3050:string[][])
                      }
                      frame True {
                        n1720 = local read "New: Trap Density-VT"() -> (w3071:dbl)
                        n1721 = Search 1D Array(1D array=w3059, element="STS-Sat (V/decade):") -> (index of element=w3066:i32)  [unwired: 1 in]
                        n1722 = Divide(x=w3066, y=3) -> (x/y=w3065:dbl)
                        n1723 = To Word Integer(number=w3065) -> (16bit integer=w3067:i16)
                        n1724 = Format Value(format string="%#g", value (0)=w3071) -> (output string=w3062:string)  [unwired: 1 in]
                        n1725 = Build Array(w3058, w3062) -> (w3069:string[])
                        n1726 = Increment(x=w3067) -> (x+1=w3068:i16)
                        n1727 = Insert Into Array(array=w3060, index (row)=w3068, new element=w3069) -> (w3061:string[][])  [unwired: 1 in]
                      }
                    }
                    n1728 = local write "Save1 Array"(w3044) -> ()
                  }
                  frame #13 {
                    w3073 = "Trap Density-STS (Traps/Vcm^2):"
                    n1729 = local read "Save1 Array"() -> (w3075:string[][])
                    n1730 = Array Size(array=w3075) -> (size(s)=w3080:i32[])
                    n1731 = Array Subset(array=w3075, index (row)=0, index (col)=0, length (col)=3) -> (w3076:string[][])  [unwired: 1 in]
                    n1732 = Index Array(array=w3080, index=0) -> (element=w3082:i32)
                    n1733 = Reshape Array(w3076, w3082) -> (w3074:string[])
                    n1734 = Search 1D Array(1D array=w3074, element=w3073) -> (index of element=w3084:i32)  [unwired: 1 in]
                    n1735 = Equal?(x=w3084, y=-1) -> (x = y?=w3083:bool)
                    n1736 = case shown="True" w3083 {
                      tunnel: w3075 -> [w3093 w3098]
                      tunnel: w3084 -> [w3090 _]
                      tunnel: [w3089 w3099] -> w3072
                      tunnel: w3074 -> [_ w3097]
                      tunnel: w3073 -> [_ w3096]
                      frame False {
                        n1737 = local read "New: Trap Density-STS"() -> (w3087:dbl)
                        n1738 = Divide(x=w3090, y=3) -> (x/y=w3092:dbl)
                        n1739 = To Word Integer(number=w3092) -> (16bit integer=w3091:i16)
                        n1740 = Format Value(format string="%#g", value (0)=w3087) -> (output string=w3086:string)  [unwired: 1 in]
                        n1741 = Replace Array Subset(array=w3093, new element=w3086, index (row)=w3091, index (col)=1) -> (w3089:string[][])
                      }
                      frame True {
                        n1742 = local read "New: Trap Density-STS"() -> (w3100:dbl)
                        n1743 = Search 1D Array(1D array=w3097, element="Trap Density-VT (Traps/Vcm^2):") -> (index of element=w3105:i32)  [unwired: 1 in]
                        n1744 = Divide(x=w3105, y=3) -> (x/y=w3106:dbl)
                        n1745 = To Word Integer(number=w3106) -> (16bit integer=w3104:i16)
                        n1746 = Format Value(format string="%#g", value (0)=w3100) -> (output string=w3109:string)  [unwired: 1 in]
                        n1747 = Build Array(w3096, w3109) -> (w3102:string[])
                        n1748 = Increment(x=w3104) -> (x+1=w3103:i16)
                        n1749 = Insert Into Array(array=w3098, index (row)=w3103, new element=w3102) -> (w3099:string[][])  [unwired: 1 in]
                      }
                    }
                    n1750 = local write "Save1 Array"(w3072) -> ()
                  }
                }
                n1751 = String To Path(string=w2646) -> (path=w2629:path)
                "No Image 2" <- w2629
              }
              frame #1 {
                n1752 = Equal?(x=w3113, y=w3112) -> (x = y?=w3111:bool)
                n1753 = case shown="False" w3111 {
                  tunnel: w3113 -> [w3117 _]
                  tunnel: w3112 -> [w3116 _]
                  frame False {
                    n1754 = Move(source path=w3117, 9:TRUE, 10:w3116) -> ()  [unwired: 2 in, 3 out]
                  }
                  frame True {
                  }
                }
              }
              frame #2 {
                n1755 = local write "Transfer File"(w3119) -> ()
                n1756 = call-poly <vilib>:"Write To Spreadsheet File.vi"("2D data"=w3118, "file path (dialog if empty)"=w3119) -> ()  [unwired: 6 in, 1 out]
              }
              frame #3 {
                w3147 = 0
                w3160 = "\\"
                w3161 = "TSP"
                w3295 = 0
                # "Transpose"
                # "Moves to next file and displays new image/data"
                n1757 = property on="Image Out" class="ImageControl"() -> (error out=w3258:errorcluster, "Image Center Position"=w3262:cluster{"X":u32, "Y":u32})  [unwired: 2 in, 1 out]
                n1758 = local read "Transfer File"() -> (w3300:path)
                n1759 = Strip Path(path=w3300) -> (stripped path=w3153:path, name=w3308:string)
                n1760 = Unbundle(w3262) -> ("X"=w3260:u32)  [unwired: 1 out]
                n1761 = Strip Path(path=w3153) -> (stripped path=w3156:path)  [unwired: 1 out]
                n1762 = local write "Transfer Folder"(w3153) -> ()
                n1763 = Bundle("X"=w3260, 0) -> (w3261:cluster{"X":u32, i32})  [unwired: 1 in]
                n1764 = local read "Folder Index"() -> (w3174:dbl)
                n1765 = Path To String(path=w3156) -> (string=w3159:string)
                n1766 = property on="Image Out" class="ImageControl"(error in=w3258, "Image Center Position"=w3261) -> ()  [unwired: 1 in, 2 out]
                n1767 = List Folder(path=w3153) -> (filenames=w3305:string[])  [unwired: 3 in, 3 out]
                n1768 = Search 1D Array(1D array=w3305, element=w3308) -> (index of element=w3302:i32)  [unwired: 1 in]
                n1769 = Array Size(array=w3305) -> (size(s)=w3301:i32)
                n1770 = Decrement(x=w3301) -> (x-1=w3303:i32)
                n1771 = Equal?(x=w3302, y=w3303) -> (x = y?=w3304:bool)
                n1772 = local read "Folder Index"() -> (w3254:dbl)
                n1773 = case shown="False" w3304 {
                  tunnel: w3254 -> [w3444 _]
                  tunnel: [w3443 0] -> w3253
                  frame False {
                    n1774 = Increment(x=w3444) -> (x+1=w3443:dbl)
                  }
                  frame True {
                  }
                }
                n1775 = invoke on="Image Out" class="ImageControl" method="Clear ROI"() -> ()  [unwired: 3 in, 3 out]
                n1776 = local write "Folder Index"(w3253) -> ()
                n1777 = Path To String(path=w3153) -> (string=w3309:string)
                n1778 = Index Array(array=w3305, index=w3253) -> (element=w3152:string)
                n1779 = String Subset(string=w3152, offset (0)=3) -> (substring=w3155:string)  [unwired: 1 in]
                n1780 = Concatenate Strings(w3161, w3155) -> (w3157:string)
                n1781 = Concatenate Strings(w3159, w3160, w3161, w3160, w3157) -> (w3158:string)
                n1782 = String To Path(string=w3158) -> (path=w3151:path)
                n1783 = local write "Transport File"(w3151) -> ()
                n1784 = Strip Path(path=w3151) -> (stripped path=w3173:path, name=w3164:string)
                n1785 = local write "Transport Folder"(w3173) -> ()
                n1786 = List Folder(path=w3173) -> (filenames=w3168:string[], error out=w3176:errorcluster)  [unwired: 3 in, 2 out]
                n1787 = Array Size(array=w3168) -> (size(s)=w3172:i32)
                n1788 = Search 1D Array(1D array=w3168, element=w3164) -> (index of element=w3171:i32)  [unwired: 1 in]
                n1789 = Decrement(x=w3172) -> (x-1=w3170:i32)
                n1790 = Equal?(x=w3171, y=w3170) -> (x = y?=w3169:bool)
                n1791 = case shown="False" w3169 {
                  tunnel: w3174 -> [w3312 _]
                  tunnel: [w3311 0] -> w3175
                  tunnel: w3176 -> [w3310 w3313]
                  tunnel: [w3310 w3313] -> _
                  frame False {
                    n1792 = Increment(x=w3312) -> (x+1=w3311:dbl)
                  }
                  frame True {
                  }
                }
                n1793 = local write "Folder Index"(w3175) -> ()
                n1794 = Path To String(path=w3173) -> (string=w3163:string)
                n1795 = Index Array(array=w3168, index=w3175) -> (element=w3167:string)
                n1796 = local write "Data Name:"(w3167) -> ()
                n1797 = Concatenate Strings(w3163, "\\", w3167) -> (w3165:string)
                n1798 = String To Path(string=w3165) -> (path=w3162:path)
                n1799 = Strip Path(path=w3162) -> ()  [unwired: 2 out]
                n1800 = call-poly <vilib>:"Read From Spreadsheet File.vi"("file path (dialog if empty)"=w3162) -> ("all rows"=w3190:string[][])  [unwired: 6 in, 4 out]
                n1801 = Array Size(array=w3190) -> (size(s)=w3196:i32[])
                n1802 = Array Subset(array=w3190, length (col)=1) -> (w3192:string[][])  [unwired: 3 in]
                n1803 = Index Array(array=w3196, index=0) -> (element=w3185:i32)
                n1804 = Reshape Array(w3192, w3185) -> (w3191:string[])
                n1805 = Search 1D Array(1D array=w3191, element="Vd") -> (index of element=w3189:i32)  [unwired: 1 in]
                n1806 = Increment(x=w3189) -> (x+1=w3188:i32)
                n1807 = Array Subset(array=w3190, index (row)=w3188) -> (w3186:string[][])  [unwired: 3 in]
                n1808 = local write "Data Name:"(w3152) -> ()
                n1809 = Fract/Exp String To Number(string=w3186, default (0 dbl)="default (0 dbl) 4") -> (number=w3178:ext[][])  [unwired: 2 in, 1 out]
                n1810 = Delete From Array(array=w3178) -> (array with subset deleted=w3177:ext[][])  [unwired: 3 in, 1 out]
                n1811 = Concatenate Strings(w3309, "\\", w3152) -> (w3307:string)
                n1812 = Delete From Array(array=w3177, index (col)=0 ("Deaktivierter Index (Spalte)")) -> (deleted portion=w3182:ext[], array with subset deleted=w3183:ext[][])  [unwired: 2 in]
                n1813 = String To Path(string=w3307) -> (path=w3125:path)
                n1814 = call "Recorded Values.vi"("Path"=w3125) -> ("Recorded Char"=w3212:T6, "Recorded Prop"=w3213:T7, "Fabrication Prop"=w3211:T8)  [unwired: 8 in]
                n1815 = Unbundle By Name(w3212) -> ("Mobility-Sat"=w3225:dbl, "Moblitity-Lin"=w3226:dbl, "On/Off"=w3227:dbl, "Off Current"=w3228:dbl, "Vt-Sat"=w3205:dbl, "STS"=w3229:dbl, "Trap Density-VT"=w3230:dbl, "Trap Density-STS"=w3231:dbl)
                n1816 = Unbundle By Name(w3213) -> ("Date Recorded"=w3221:string, "Index"=w3222:string, "Length"=w3223:dbl, "Width"=w3224:dbl, "Sample Temp"=w3208:dbl)
                n1817 = Unbundle By Name(w3211) -> ("Date Created"=w3232:string, "Material"=w3214:string, "Solvent"=w3215:string, "Concentration"=w3216:dbl, "Method"=w3217:string, "Dielectric (nm)"=w3218:dbl, "Treatment"=w3219:string, "Comments"=w3220:string)
                n1818 = local write "Rec: Off I-Sat"(w3228) -> ()
                n1819 = local write "Rec: Comments"(w3220) -> ()
                n1820 = local write "Rec: VT-Sat"(w3205) -> ()
                n1821 = local write "Date Created"(w3232) -> ()
                n1822 = local write "Rec: Material"(w3214) -> ()
                n1823 = local write "Rec: Solvent"(w3215) -> ()
                n1824 = local write "Rec: Concentration"(w3216) -> ()
                n1825 = local write "Rec: Method"(w3217) -> ()
                n1826 = local write "Rec: Dielectric (d)"(w3218) -> ()
                n1827 = local write "Surface Treatment:"(w3219) -> ()
                n1828 = local write "Index"(w3222) -> ()
                n1829 = local write "Rec: Mobility-Sat"(w3225) -> ()
                n1830 = local write "Rec: Mobility-Lin"(w3226) -> ()
                n1831 = local write "Rec: On/Off"(w3227) -> ()
                n1832 = local write "Rec: STS"(w3229) -> ()
                n1833 = local write "Rec: Trap Density-VT"(w3230) -> ()
                n1834 = local write "Rec: Trap Density-STS"(w3231) -> ()
                n1835 = local write "Date Recorded"(w3221) -> ()
                n1836 = local write "Rec: Length"(w3223) -> ()
                n1837 = local write "Rec: Width"(w3224) -> ()
                n1838 = local write "Rec: Temp"(w3208) -> ()
                n1839 = Equal To 0?(x=w3208) -> (x = 0?=w3209:bool)
                n1840 = case shown="False" w3209 {
                  tunnel: [w3321 w3322] -> w3206
                  tunnel: w3208 -> [w3321 _]
                  frame False {
                  }
                  frame True {
                    n1841 = local read "Room Temp"() -> (w3322:dbl)
                  }
                }
                n1842 = local read "NumPoints Log"() -> (w3250:dbl)
                n1843 = Transpose 2D Array(2D array=w3183) -> (transposed array=w3184:ext[][])
                n1844 = local write "Transfer File"(w3125) -> ()
                n1845 = local read "Num Pts"() -> (w3240:dbl)
                n1846 = local read "Num Pts"() -> (w3251:dbl)
                n1847 = for {
                  tunnel: w3182 -> [w3319]
                  tunnel: w3184 -> [w3320] mode=indexing
                  tunnel: [w3318] -> w3180 mode=indexing
                  n1848 = Bundle(w3319, w3320) -> (w3318:cluster{ext[], ext[]})  [unwired: 1 in]
                }
                n1849 = call-poly <vilib>:"Read From Spreadsheet File.vi"("file path (dialog if empty)"=w3125) -> ("all rows"=w3297:string[][])  [unwired: 6 in, 4 out]
                n1850 = call "Mobility-Vt Calculator-File.vi"("NumPts"=w3251, "Path"=w3125) -> ("Used Points"=w3124:T10, "Graph Cluster"=w3202:T11, "Output"=w3252:T12)  [unwired: 6 in, 1 out]
                n1851 = Unbundle By Name(w3124) -> ("Index-Lin"=w3123:dbl, "Index-Sat"=w3122:dbl)
                n1852 = Unbundle By Name(w3202) -> ("Raw Sat"=w3199:cluster{dbl[], dbl[]}[], "Sqrt Sat"=w3201:cluster{dbl[], dbl[]}[], "Raw Lin"=w3198:cluster{dbl[], dbl[]}[], "Sqrt Lin"=w3200:cluster{dbl[], dbl[]}[], "Log Lin"=w3197:cluster{dbl[], dbl[]}[])  [unwired: 1 out]
                n1853 = Decimate 1D Array(w3200) -> (w3247:cluster{dbl[], dbl[]}[])  [unwired: 1 out]
                n1854 = Array To Cluster(array=w3247) -> (cluster=w3245:T13)
                n1855 = Unbundle(w3245) -> ("[0]"=w3246:cluster{dbl[], dbl[]})  [unwired: 8 out]
                n1856 = Unbundle(w3246) -> (w3244:dbl[], w3243:dbl[])
                n1857 = Array Subset(array=w3243, index=w3123, length=w3240) -> (w3241:dbl[])
                n1858 = Array Subset(array=w3244, index=w3123, length=w3240) -> (w3242:dbl[])
                n1859 = call "STS Calculator-File.vi"("NumPts"=w3250, "Path"=w3125) -> ("Used Points"=w3121:T9, "XY Graph-Sat"=w3249:cluster{dbl[], dbl[]}[], "Ouput"=w3248:cluster{"STS-Sat":dbl, "STS-Lin":dbl})  [unwired: 6 in, 1 out]
                n1860 = Unbundle By Name(w3121) -> ("STS Index-Sat"=w3120:dbl)
                n1861 = local write "Transport"(w3180) -> ()
                n1862 = Array Size(array=w3180) -> (size(s)=w3179:i32)
                n1863 = local read "New: Dielectric"() -> (w3236:dbl)
                n1864 = local write "Sat-Trans Slider"(w3122) -> ()
                n1865 = for {
                  N: w3179 -> [_]
                  i -> [w3317]
                  n1866 = local read "Transport Line Color"() -> (w3316:u32)
                  n1867 = local read "Ring"() -> (w3315:u16)
                  n1868 = property on="Transport" class="XYGraph (strict)"("Active Plot"=w3317, "Plot.Plot Color"=w3316, "Plot.Line Width"=w3315) -> ()  [unwired: 2 in, 2 out]
                }
                n1869 = local write "Lin Id-Used"(w3241) -> ()
                n1870 = local write "Lin-Vg Array-Used"(w3242) -> ()
                n1871 = local write "MobVi Index"(w3122) -> ()
                n1872 = local write "Index 2"(w3120) -> ()
                n1873 = local write "Sqrt-Sat"(w3201) -> ()
                n1874 = local write "Sat-Log"(w3249) -> ()
                n1875 = Unbundle By Name(w3252) -> ("Mobility-Sat"=w3239:dbl, "Vt-Sat"=w3203:dbl, "Mobility-Lin"=w3238:dbl, "Mobility-Lin"=w3237:dbl, "Off I-Sat"=w3233:dbl, "On/Off I-Sat"=w3204:dbl)
                n1876 = local write "Sqrt-Lin"(w3200) -> ()
                n1877 = Array Size(array=w3297) -> (size(s)=w3296:i32[])
                n1878 = local write "Raw- Sat"(w3199) -> ()
                n1879 = local write "New: Temp"(w3206) -> ()
                n1880 = Unbundle By Name(w3248) -> ("STS-Sat"=w3235:dbl)
                n1881 = call "Trap Density_STS.vi"("Temp (T) [K]"=w3206, "S.T.S. (S)"=w3235, "Dielectric"=w3236) -> ("Trap Density (N)"=w3210:dbl)  [unwired: 8 in]
                n1882 = local write "Calc: Mobility-Lin"(w3238) -> ()
                n1883 = local write "Raw- Lin"(w3198) -> ()
                n1884 = local write "Calc: Mobility-Sat"(w3239) -> ()
                n1885 = local write "Log-Lin"(w3197) -> ()
                n1886 = local write "Calc: Off I-Sat"(w3233) -> ()
                n1887 = local write "Calc: VT-Sat"(w3203) -> ()
                n1888 = local write "New: VT-Lin"(w3237) -> ()
                n1889 = local write "New: Trap Density-STS"(w3210) -> ()
                n1890 = local write "Calc: Trap Density-STS"(w3210) -> ()
                n1891 = local read "Image Folder"() -> (w3286:path)
                n1892 = local read "New: Dielectric"() -> (w3234:dbl)
                n1893 = Decimate 1D Array(w3201) -> (w3281:cluster{dbl[], dbl[]}[])  [unwired: 1 out]
                n1894 = Decimate 1D Array(w3249) -> (w3271:cluster{dbl[], dbl[]}[])  [unwired: 1 out]
                n1895 = Index Array(array=w3296, index=w3295) -> (element=w3277:i32)
                n1896 = Array Subset(array=w3297, index (row)=w3295, index (col)=w3295, length (col)=3) -> (w3298:string[][])  [unwired: 1 in]
                n1897 = local write "Calc: STS"(w3235) -> ()
                n1898 = local write "New: VT-Sat"(w3203) -> ()
                n1899 = local write "New: Mobility-Sat"(w3239) -> ()
                n1900 = local write "Calc: On/Off"(w3204) -> ()
                n1901 = local write "New: Mobility-Lin"(w3238) -> ()
                n1902 = List Folder(path=w3286) -> (filenames=w3291:string[])  [unwired: 3 in, 3 out]
                n1903 = local write "New: VT-Lin"(w3237) -> ()
                n1904 = Array To Cluster(array=w3281) -> (cluster=w3283:T13)
                n1905 = Array To Cluster(array=w3271) -> (cluster=w3269:T13)
                n1906 = Reshape Array(w3298, w3277) -> (w3284:string[])
                n1907 = Subtract(x=w3277, y=20) -> (x-y=w3276:i32)
                n1908 = local write "New: STS"(w3235) -> ()
                n1909 = property on="Sat-Trans Slider" class="Slide (strict)"("Scale.Maximum"=w3276) -> ()  [unwired: 2 in, 2 out]
                n1910 = call "Trap Density_VT.vi"("VT"=w3203, "Dielectric"=w3234) -> ("Trap Density-VT"=w3207:dbl)
                n1911 = Unbundle(w3283) -> ("[0]"=w3282:cluster{dbl[], dbl[]})  [unwired: 8 out]
                n1912 = Unbundle(w3269) -> ("[0]"=w3270:cluster{dbl[], dbl[]})  [unwired: 8 out]
                n1913 = Search 1D Array(1D array=w3284, element="Index:") -> (index of element=w3292:i32)  [unwired: 1 in]
                n1914 = local write "New: Trap Density-VT"(w3207) -> ()
                n1915 = local write "Calc: Trap Density-VT"(w3207) -> ()
                n1916 = call-poly <vilib>:"Read From Spreadsheet File.vi"("file path (dialog if empty)"=w3125) -> ("all rows"=w3129:string[][])  [unwired: 6 in, 4 out]
                n1917 = Unbundle(w3282) -> (w3273:dbl[], w3272:dbl[])
                n1918 = Unbundle(w3270) -> (w3268:dbl[], w3267:dbl[])
                n1919 = Increment(x=w3292) -> (x+1=w3293:i32)
                n1920 = Array Size(array=w3129) -> (size(s)=w3148:i32[])
                n1921 = Array Subset(array=w3273, index=w3122, length=w3251) -> (w3280:dbl[])
                n1922 = Array Subset(array=w3272, index=w3122, length=w3251) -> (w3279:dbl[])
                n1923 = Array Subset(array=w3268, index=w3120, length=w3250) -> (w3275:dbl[])
                n1924 = Array Subset(array=w3267, index=w3120, length=w3250) -> (w3274:dbl[])
                n1925 = Index Array(array=w3284, index=w3293) -> (element=w3289:string)
                n1926 = local write "Vg Array-Log-Used"(w3274) -> ()
                n1927 = local write "Sat Id-Log-Used"(w3275) -> ()
                n1928 = local write "Sat Id-Used"(w3279) -> ()
                n1929 = local write "Index"(w3289) -> ()
                n1930 = Index Array(array=w3148, index=0) -> (element=w3146:i32)
                n1931 = local write "Sat Vg Array-Used"(w3280) -> ()
                n1932 = while {
                  tunnel: w3291 -> [w3330]
                  tunnel: w3289 -> [w3328]
                  tunnel: [w3327] -> _
                  tunnel: [w3327] -> w3290
                  tunnel: w3277 -> [w3326]
                  i -> [w3327]
                  stop <- w3323 stop-if-true
                  n1933 = Index Array(array=w3330, index=w3327) -> (element=w3331:string)
                  n1934 = xnode "Match Regular Expression"("input string"=w3331, "regular expression"=w3328) -> ("whole match"=w3329:string)  [unwired: 4 in, 4 out]
                  n1935 = Equal?(x=w3329, y=w3328) -> (x = y?=w3325:bool)
                  n1936 = Equal?(x=w3326, y=w3327) -> (x = y?=w3324:bool)
                  n1937 = Or(x=w3325, y=w3324) -> (x .or. y?=w3323:bool)
                }
                n1938 = Array Subset(array=w3129, index (row)=w3147, index (col)=w3147, length (col)=3) -> (w3149:string[][])  [unwired: 1 in]
                n1939 = Reshape Array(w3149, w3146) -> (w3131:string[])
                n1940 = Search 1D Array(1D array=w3131, element="Vg") -> (index of element=w3135:i32)  [unwired: 1 in]
                n1941 = Add(x=w3135, y=3) -> (x+y=w3133:i32)
                n1942 = Divide(x=w3133, y=3) -> (x/y=w3140:dbl)
                n1943 = Array Subset(array=w3129, index (row)=w3140, index (col)=0, length (col)=1) -> (w3139:string[][])  [unwired: 1 in]
                n1944 = Fract/Exp String To Number(string=w3139) -> (number=w3143:dbl[][])  [unwired: 3 in, 1 out]
                n1945 = Array Size(array=w3143) -> (size(s)=w3130:i32[])
                n1946 = Index Array(array=w3130, index=0) -> (element=w3141:i32)
                n1947 = Decrement(x=w3141) -> (x-1=w3144:i32)
                n1948 = Reshape Array(w3143, w3144) -> (w3128:dbl[])
                n1949 = local write "Data Length"(w3144) -> ()
                n1950 = local write "Vg Column"(w3128) -> ()
                n1951 = Array Max & Min(array=w3128) -> (max value=w3127:dbl, min value=w3126:dbl)  [unwired: 2 out]
                n1952 = Path To String(path=w3286) -> (string=w3288:string)
                n1953 = Index Array(array=w3291, index=w3290) -> (element=w3265:string)
                n1954 = local write "Image Name"(w3265) -> ()
                n1955 = property on="Sat-Trans Slider" class="Slide (strict)"("Scale.Maximum"=w3127, "Scale.Minimum"=w3126) -> ()  [unwired: 2 in, 2 out]
                n1956 = Empty String/Path?(string/path=w3265) -> (empty?=w3266:bool)
                n1957 = Concatenate Strings(w3288, "\\", w3265) -> (w3287:string)
                n1958 = String To Path(string=w3287) -> (path=w3264:path)
                n1959 = local read "No Image File"() -> (w3263:path)
                n1960 = Select(t=w3263, s=w3266, f=w3264) -> (s? t:f=w3257:path)
                n1961 = local write "Image File"(w3257) -> ()
                n1962 = local read "Image Out"() -> (w3255:T2)
                n1963 = call "IMAQ ReadFile"("File Path"=w3257, "Image"=w3255) -> ("Image Out"=w3256:T2)  [unwired: 5 in, 4 out]
                n1964 = local write "Image Out"(w3256) -> ()
                n1965 = local write "Image Out 2"(w3256) -> ()
              }
              frame #4 {
                # "Output ROI data"
                n1966 = local read "Image Folder"() -> (w3446:path)
                n1967 = Build Path(base path=w3446, name or relative path="ROI") -> (appended path=w3448:path)
                n1968 = local read "Index"() -> (w3447:string)
                n1969 = Build Path(base path=w3448, name or relative path=w3447) -> (appended path=w3453:path)
                n1970 = invoke on="Image Out" class="ImageControl" method="Clear ROI"() -> (error out=w3452:errorcluster)  [unwired: 3 in, 2 out]
                n1971 = call <vilib>:"Check if File or Folder Exists.vi"("error in (no error)"=w3452, "path"=w3453) -> ("file or folder exists?"=w3450:bool, "dup path"=w3451:path)  [unwired: 7 in, 1 out]
                n1972 = case shown="True" w3450 {
                  tunnel: w3451 -> [_ w3454]
                  frame False {
                  }
                  frame True {
                    n1973 = Read from Text File(file (use dialog)=w3454) -> (text=w3458:string)  [unwired: 3 in, 3 out]
                    n1974 = property on="Image Out" class="ImageControl"() -> ("ROI"=w3455:T14)  [unwired: 2 in, 2 out]
                    n1975 = Unflatten From String(type=w3455, binary string=w3458) -> (value=w3456:T14, error out=w3457:errorcluster)  [unwired: 3 in, 1 out]
                    n1976 = property on="Image Out" class="ImageControl"(error in=w3457, "ROI"=w3456) -> ()  [unwired: 1 in, 2 out]
                  }
                }
              }
            }
            n1977 = flat-sequence {
              tunnel: [w2586] -> w2573
              tunnel: w2573 -> [w2600]
              frame #0 {
                # "Makes Empty File for Transformer Data"
                n1978 = local read "Transfer Folder"() -> (w2575:path)
                n1979 = Build Path(base path=w2575, name or relative path="Stats") -> (appended path=w2577:path)
                n1980 = call <vilib>:"Check if File or Folder Exists.vi"("path"=w2577) -> ("file or folder exists?"=w2578:bool, "dup path"=w2579:path)  [unwired: 8 in, 1 out]
                n1981 = case shown="False" w2578 {
                  tunnel: [w2583 w2585] -> w2580
                  tunnel: w2579 -> [w2584 w2585]
                  frame False {
                    n1982 = Create Folder(path (use dialog)=w2584) -> (created path=w2583:path)  [unwired: 2 in, 2 out]
                  }
                  frame True {
                  }
                }
                n1983 = Build Path(base path=w2580, name or relative path="Tranformer Data.txt") -> (appended path=w2582:path)
                n1984 = call-poly <vilib>:"Write To Spreadsheet File.vi"("append to file? (new file:F)"=TRUE, "file path (dialog if empty)"=w2582) -> ()  [unwired: 6 in, 1 out]
              }
              frame #1 {
                # "Adds Headers if they don't exist"
                n1985 = local read "Transfer Folder"() -> (w2592:path)
                n1986 = Concatenate Strings("Stats\\", "Tranformer Data.txt") -> (w2593:string)
                n1987 = Build Path(base path=w2592, name or relative path=w2593) -> (appended path=w2586:path)
                n1988 = call-poly <vilib>:"Read From Spreadsheet File.vi"("file path (dialog if empty)"=w2586) -> ("first row"=w2591:string[])  [unwired: 6 in, 4 out]
                n1989 = Search 1D Array(1D array=w2591, element="DeviceID") -> (index of element=w2589:i32)  [unwired: 1 in]
                n1990 = Equal?(x=w2589, y=0) -> (x = y?=w2587:bool)
                n1991 = case shown="False" w2587 {
                  tunnel: w2586 -> [w2597 _]
                  frame False {
                    n1992 = local read "Transformer \nHeaders"() -> (w2596:string[])
                    n1993 = call-poly <vilib>:"Write To Spreadsheet File.vi"("1D data"=w2596, "file path (dialog if empty)"=w2597) -> ()  [unwired: 6 in, 1 out]
                  }
                  frame True {
                  }
                }
              }
              frame #2 {
                # "Adds current device if it doesn't exist"
                n1994 = local read "Current \nRecord"() -> (w2603:string[])
                n1995 = Index Array(array=w2603, index=0) -> (element=w2602:string)
                n1996 = local read "Transfer Folder"() -> (w2605:path)
                n1997 = Concatenate Strings("Stats\\", "Tranformer Data.txt") -> (w2606:string)
                n1998 = local write "Current Device ID"(w2602) -> ()
                n1999 = local read "Current Device ID"() -> (w2612:string)
                n2000 = Build Path(base path=w2605, name or relative path=w2606) -> (appended path=w2604:path)
                n2001 = call-poly <vilib>:"Read From Spreadsheet File.vi"("file path (dialog if empty)"=w2604) -> ("all rows"=w2599:string[][])  [unwired: 6 in, 4 out]
                n2002 = Index Array(array=w2599, index (col)=0) -> (element=w2610:string[])  [unwired: 1 in]
                n2003 = Search 1D Array(1D array=w2610, element=w2612) -> (index of element=w2598:i32)  [unwired: 1 in]
                n2004 = Equal?(x=w2598, y=-1) -> (x = y?=w2601:bool)
                n2005 = case shown="False" w2601 {
                  tunnel: w2600 -> [w2614 w2627]
                  tunnel: w2598 -> [w2619 _]
                  tunnel: w2599 -> [w2620 _]
                  frame False {
                    n2006 = local read "Current \nRecord"() -> (w2618:string[])
                    n2007 = Replace Array Subset(array=w2620, new element=w2618, index (row)=w2619) -> (w2615:string[][])  [unwired: 1 in]
                    n2008 = flat-sequence {
                      tunnel: [w2621] -> _
                      tunnel: [w2622] -> _
                      tunnel: [w2622] -> w2617
                      tunnel: [w2621] -> w2616
                      tunnel: w2615 -> [w2622]
                      tunnel: w2614 -> [w2621]
                      tunnel: w2617 -> [w2624]
                      tunnel: w2616 -> [w2623]
                      frame #0 {
                        n2009 = Delete(path (use dialog)=w2621) -> ()  [unwired: 4 in, 3 out]
                      }
                      frame #1 {
                        n2010 = call-poly <vilib>:"Write To Spreadsheet File.vi"("append to file? (new file:F)"=TRUE, "2D data"=w2624, "file path (dialog if empty)"=w2623) -> ()  [unwired: 5 in, 1 out]
                      }
                    }
                  }
                  frame True {
                    n2011 = local read "Current \nRecord"() -> (w2626:string[])
                    n2012 = call-poly <vilib>:"Write To Spreadsheet File.vi"("append to file? (new file:F)"=TRUE, "1D data"=w2626, "file path (dialog if empty)"=w2627) -> ()  [unwired: 5 in, 1 out]
                  }
                }
              }
            }
          }
          event "Export": Mouse Down {
            n2013 = event-data() -> ()  [unwired: 1 in, 7 out]
            n2014 = flat-sequence {
              frame #0 {
                n2015 = stacked-sequence {
                  frame #0 {
                    n2016 = local read "Independant Variable"() -> (w3460:string)
                    n2017 = Equal?(x=w3460, y="Length (um):") -> (x = y?=w3461:bool)
                    n2018 = case shown="True" w3461 {
                      frame False {
                      }
                      frame True {
                        n2019 = local write "X Axis Display Type"("1") -> ()
                        n2020 = local write "Opj X Axis"("2") -> ()
                      }
                    }
                  }
                  frame #1 {
                    n2021 = local read "Independant Variable"() -> (w3465:string)
                    n2022 = Equal?(x=w3465, y="Sample Temp (K):") -> (x = y?=w3466:bool)
                    n2023 = case shown="True" w3466 {
                      frame False {
                      }
                      frame True {
                        n2024 = local write "X Axis Display Type"("1") -> ()
                        n2025 = local write "Opj X Axis"("1") -> ()
                      }
                    }
                  }
                  frame #2 {
                    n2026 = local read "Independant Variable"() -> (w3470:string)
                    n2027 = Equal?(x=w3470, y="Mobility-Sat (cm^2/Vs):") -> (x = y?=w3471:bool)
                    n2028 = case shown="True" w3471 {
                      frame False {
                      }
                      frame True {
                        n2029 = local write "X Axis Display Type"("2") -> ()
                        n2030 = local write "Opj X Axis"("2") -> ()
                      }
                    }
                  }
                  frame #3 {
                    n2031 = local read "Independant Variable"() -> (w3475:string)
                    n2032 = Equal?(x=w3475, y="Mobility-Lin (cm^2/Vs):") -> (x = y?=w3476:bool)
                    n2033 = case shown="True" w3476 {
                      frame False {
                      }
                      frame True {
                        n2034 = local write "X Axis Display Type"("2") -> ()
                        n2035 = local write "Opj X Axis"("2") -> ()
                      }
                    }
                  }
                  frame #4 {
                    n2036 = local read "Independant Variable"() -> (w3480:string)
                    n2037 = Equal?(x=w3480, y="On/Off I-Sat:") -> (x = y?=w3481:bool)
                    n2038 = case shown="True" w3481 {
                      frame False {
                      }
                      frame True {
                        n2039 = local write "X Axis Display Type"("2") -> ()
                        n2040 = local write "Opj X Axis"("2") -> ()
                      }
                    }
                  }
                  frame #5 {
                    n2041 = local read "Independant Variable"() -> (w3485:string)
                    n2042 = Equal?(x=w3485, y="Off I-Sat (A):") -> (x = y?=w3486:bool)
                    n2043 = case shown="True" w3486 {
                      frame False {
                      }
                      frame True {
                        n2044 = local write "X Axis Display Type"("2") -> ()
                        n2045 = local write "Opj X Axis"("2") -> ()
                      }
                    }
                  }
                  frame #6 {
                    n2046 = local read "Independant Variable"() -> (w3490:string)
                    n2047 = Equal?(x=w3490, y="Vt-Sat (V):") -> (x = y?=w3491:bool)
                    n2048 = case shown="True" w3491 {
                      frame False {
                      }
                      frame True {
                        n2049 = local write "X Axis Display Type"("1") -> ()
                        n2050 = local write "Opj X Axis"("1") -> ()
                      }
                    }
                  }
                  frame #7 {
                    n2051 = local read "Independant Variable"() -> (w3495:string)
                    n2052 = Equal?(x=w3495, y="STS-Sat (V/decade):") -> (x = y?=w3496:bool)
                    n2053 = case shown="True" w3496 {
                      frame False {
                      }
                      frame True {
                        n2054 = local write "X Axis Display Type"("1") -> ()
                        n2055 = local write "Opj X Axis"("1") -> ()
                      }
                    }
                  }
                  frame #8 {
                    n2056 = local read "Independant Variable"() -> (w3500:string)
                    n2057 = Equal?(x=w3500, y="Trap Density-VT (Traps/Vcm^2):") -> (x = y?=w3501:bool)
                    n2058 = case shown="True" w3501 {
                      frame False {
                      }
                      frame True {
                        n2059 = local write "X Axis Display Type"("2") -> ()
                        n2060 = local write "Opj X Axis"("2") -> ()
                      }
                    }
                  }
                  frame #9 {
                    n2061 = local read "Independant Variable"() -> (w3505:string)
                    n2062 = Equal?(x=w3505, y="Trap Density-STS (Traps/Vcm^2):") -> (x = y?=w3506:bool)
                    n2063 = case shown="True" w3506 {
                      frame False {
                      }
                      frame True {
                        n2064 = local write "X Axis Display Type"("2") -> ()
                        n2065 = local write "Opj X Axis"("2") -> ()
                      }
                    }
                  }
                }
              }
              frame #1 {
                n2066 = local read "Transfer Folder"() -> (w3514:path)
                n2067 = Build Path(base path=w3514, name or relative path="Stats") -> (appended path=w3515:path)
                n2068 = local read "Origin Project File"() -> (w3526:path)
                n2069 = call <vilib>:"Check if File or Folder Exists.vi"("path"=w3515) -> ("file or folder exists?"=w3530:bool, "dup path"=w3529:path)  [unwired: 8 in, 1 out]
                n2070 = call <userlib>:"OA_ConnectToOrigin.vi"() -> ("error out"=w3527:errorcluster, "Origin.IOApplication"=w3528:refnum<k7>)  [unwired: 8 in]
                n2071 = case shown="False" w3530 {
                  tunnel: w3529 -> [w3703 w3704]
                  tunnel: [w3702 w3704] -> w3513
                  frame False {
                    n2072 = Create Folder(path (use dialog)=w3703) -> (created path=w3702:path)  [unwired: 2 in, 2 out]
                  }
                  frame True {
                  }
                }
                n2073 = call <userlib>:"OA_Load.vi"("error in (no error)"=w3527, "Path"=w3526, "Origin.IOApplication"=w3528) -> ("error out"=w3524:errorcluster, "Origin.IOApplication"=w3525:refnum<k7>)  [unwired: 1 out]
                n2074 = call "OAExecute.vi"("script"="document -m 3;", "Error IO"=w3524, "Origin.IOApplication"=w3525) -> ("Error IO Out"=w3522:errorcluster, "Origin.IOApplication"=w3523:refnum<k7>)  [unwired: 1 in, 1 out]
                n2075 = call "File Dialog"("start path"=w3515) -> ("selected path"=w3517:path)  [unwired: 11 in, 3 out]
                n2076 = local read "Independant Variable"() -> (w3510:string)
                n2077 = stacked-sequence {
                  tunnel: w3514 -> [w3541 w3571 w3583 w3605 w3625 w3646 w3667 w3690]
                  tunnel: w3513 -> [w3542 w3570 w3584 w3604 w3626 w3647 w3668 w3691]
                  tunnel: w3523 -> [w3544 w3568 w3586 w3607 w3628 w3649 w3670 w3693]
                  tunnel: w3522 -> [w3543 w3569 w3585 w3606 w3627 w3648 w3669 w3692]
                  tunnel: [_ _ _ _ _ _ _ w3688] -> w3512
                  tunnel: [_ _ _ _ _ _ _ w3689] -> w3511
                  tunnel: w3510 -> [w3540 w3561 w3582 w3603 w3624 w3645 w3666 w3687]
                  frame #0 {
                    n2078 = local read "X Axis Display Type"() -> (w3532:string)
                    n2079 = local read "Opj X Axis"() -> (w3537:string)
                    n2080 = Concatenate Strings("window -a MOBLGraph;\nlayer.x.type=", w3537, "; layer.x.label.numFormat = ", w3532, "; Y3 = 1; X3 = 1;", "window -a MOBLTable;\nwindow -s TV;") -> (w3535:string)
                    n2081 = call "Param_Analysis_7_24b_JW.vi"("Independant Variable"=w3540, "error in (no error)"=w3543, "Data Folder"=w3541, "Parameter String"="Mobility-Lin (cm^2/Vs):", "Parameter Name"="Mobility-Lin", "Stats Folder"=w3542) -> ("error out"=w3546:errorcluster, "Output Array"=w3548:string[][], "Variables"=w3539:T20)  [unwired: 2 in, 1 out]
                    n2082 = call "Origin_Export_7_27a_JW.vi"("Input Conditions"=w3539, "Analysis Array"=w3548, "error in (no error)"=w3546, "Parameter Worksheet Name"="[MOBLTable]Mobilities", "Parameter Folder Script"="pe_cd \"Mobility-Lin\";", "Origin.IOApplication"=w3544) -> ("error out"=w3545:errorcluster, "reference out"=w3547:refnum<k7>)  [unwired: 3 in, 1 out]
                    n2083 = call "OAExecute.vi"("script"=w3535, "Error IO"=w3545, "Origin.IOApplication"=w3547) -> ()  [unwired: 1 in, 3 out]
                  }
                  frame #1 {
                    n2084 = local read "X Axis Display Type"() -> (w3553:string)
                    n2085 = local read "Opj X Axis"() -> (w3558:string)
                    n2086 = Concatenate Strings("window -a MOBSGraph;\nlayer.x.type=", w3558, "; layer.x.label.numFormat = ", w3553, "; Y3 = 1; X3 = 1;", "window -a MOBSTable;\nwindow -s TV;") -> (w3556:string)
                    n2087 = call "Param_Analysis_7_24b_JW.vi"("Independant Variable"=w3561, "error in (no error)"=w3569, "Data Folder"=w3571, "Parameter String"="Mobility-Sat (cm^2/Vs):", "Parameter Name"="Mobility-Sat", "Stats Folder"=w3570) -> ("error out"=w3564:errorcluster, "Output Array"=w3562:string[][], "Variables"=w3560:T20)  [unwired: 2 in, 1 out]
                    n2088 = call "Origin_Export_7_27a_JW.vi"("Input Conditions"=w3560, "Analysis Array"=w3562, "error in (no error)"=w3564, "Parameter Worksheet Name"="[MOBSTable]Mobilities", "Parameter Folder Script"="pe_cd \"Mobility-Sat\";", "Origin.IOApplication"=w3568) -> ("error out"=w3563:errorcluster, "reference out"=w3565:refnum<k7>)  [unwired: 3 in, 1 out]
                    n2089 = call "OAExecute.vi"("script"=w3556, "Error IO"=w3563, "Origin.IOApplication"=w3565) -> ()  [unwired: 1 in, 3 out]
                  }
                  frame #2 {
                    n2090 = local read "X Axis Display Type"() -> (w3574:string)
                    n2091 = local read "Opj X Axis"() -> (w3579:string)
                    n2092 = Concatenate Strings("window -a NSTSGraph;\nlayer.x.type=", w3579, "; layer.x.label.numFormat = ", w3574, "; Y3 = 1; X3 = 1;", "window -a NSTSTable;\nwindow -s TV;") -> (w3577:string)
                    n2093 = call "Param_Analysis_7_24b_JW.vi"("Independant Variable"=w3582, "error in (no error)"=w3585, "Data Folder"=w3583, "Parameter String"="Trap Density-STS (Traps/Vcm^2):", "Parameter Name"="Trap Density-STS", "Stats Folder"=w3584) -> ("error out"=w3589:errorcluster, "Output Array"=w3587:string[][], "Variables"=w3581:T20)  [unwired: 2 in, 1 out]
                    n2094 = call "Origin_Export_7_27a_JW.vi"("Input Conditions"=w3581, "Analysis Array"=w3587, "error in (no error)"=w3589, "Parameter Worksheet Name"="[NSTSTable]Trap Densities", "Parameter Folder Script"="pe_cd \"N-STS\";", "Origin.IOApplication"=w3586) -> ("error out"=w3588:errorcluster, "reference out"=w3590:refnum<k7>)  [unwired: 3 in, 1 out]
                    n2095 = call "OAExecute.vi"("script"=w3577, "Error IO"=w3588, "Origin.IOApplication"=w3590) -> ()  [unwired: 1 in, 3 out]
                  }
                  frame #3 {
                    n2096 = local read "X Axis Display Type"() -> (w3595:string)
                    n2097 = local read "Opj X Axis"() -> (w3600:string)
                    n2098 = call "Param_Analysis_7_24b_JW.vi"("Independant Variable"=w3603, "error in (no error)"=w3606, "Data Folder"=w3605, "Parameter String"="Trap Density-VT (Traps/Vcm^2):", "Parameter Name"="Trap Density-Vt", "Stats Folder"=w3604) -> ("error out"=w3610:errorcluster, "Output Array"=w3608:string[][], "Variables"=w3602:T20)  [unwired: 2 in, 1 out]
                    n2099 = Concatenate Strings("window -a NVtGraph;\nlayer.x.type=", w3600, "; layer.x.label.numFormat = ", w3595, "; Y3 = 1; X3 = 1;", "window -a NVtTable;\nwindow -s TV;") -> (w3598:string)
                    n2100 = call "Origin_Export_7_27a_JW.vi"("Input Conditions"=w3602, "Analysis Array"=w3608, "error in (no error)"=w3610, "Parameter Worksheet Name"="[NVTTable]Trap Densities", "Parameter Folder Script"="pe_cd \"N-Vt\";", "Origin.IOApplication"=w3607) -> ("error out"=w3609:errorcluster, "reference out"=w3611:refnum<k7>)  [unwired: 3 in, 1 out]
                    n2101 = call "OAExecute.vi"("script"=w3598, "Error IO"=w3609, "Origin.IOApplication"=w3611) -> ()  [unwired: 1 in, 3 out]
                  }
                  frame #4 {
                    n2102 = local read "X Axis Display Type"() -> (w3616:string)
                    n2103 = local read "Opj X Axis"() -> (w3621:string)
                    n2104 = Concatenate Strings("window -a OffIGraph;\nlayer.x.type=", w3621, "; layer.x.label.numFormat = ", w3616, "; Y3 = 1; X3 = 1;", "window -a OffITable;\nwindow -s TV;") -> (w3619:string)
                    n2105 = call "Param_Analysis_7_24b_JW.vi"("Independant Variable"=w3624, "error in (no error)"=w3627, "Data Folder"=w3625, "Parameter String"="Off I-Sat (A):", "Parameter Name"="Off I-Sat", "Stats Folder"=w3626) -> ("error out"=w3631:errorcluster, "Output Array"=w3629:string[][], "Variables"=w3623:T20)  [unwired: 2 in, 1 out]
                    n2106 = call "Origin_Export_7_27a_JW.vi"("Input Conditions"=w3623, "Analysis Array"=w3629, "error in (no error)"=w3631, "Parameter Worksheet Name"="[OffItable]OffCurrents", "Parameter Folder Script"="pe_cd \"OffI-Sat\";", "Origin.IOApplication"=w3628) -> ("error out"=w3630:errorcluster, "reference out"=w3632:refnum<k7>)  [unwired: 3 in, 1 out]
                    n2107 = call "OAExecute.vi"("script"=w3619, "Error IO"=w3630, "Origin.IOApplication"=w3632) -> ()  [unwired: 1 in, 3 out]
                  }
                  frame #5 {
                    n2108 = local read "X Axis Display Type"() -> (w3637:string)
                    n2109 = local read "Opj X Axis"() -> (w3642:string)
                    n2110 = Concatenate Strings("window -a OnOffGraph;\nlayer.x.type=", w3642, "; layer.x.label.numFormat = ", w3637, "; Y3 = 1; X3 = 1;", "window -a OnOffTable;\nwindow -s TV;") -> (w3640:string)
                    n2111 = call "Param_Analysis_7_24b_JW.vi"("Independant Variable"=w3645, "error in (no error)"=w3648, "Data Folder"=w3646, "Parameter String"="On/Off I-Sat:", "Parameter Name"="OnOff Ratio", "Stats Folder"=w3647) -> ("error out"=w3652:errorcluster, "Output Array"=w3650:string[][], "Variables"=w3644:T20)  [unwired: 2 in, 1 out]
                    n2112 = call "Origin_Export_7_27a_JW.vi"("Input Conditions"=w3644, "Analysis Array"=w3650, "error in (no error)"=w3652, "Parameter Worksheet Name"="[OnOffTable]On/Off Ratios", "Parameter Folder Script"="pe_cd \"OnOff-Ratio\";", "Origin.IOApplication"=w3649) -> ("error out"=w3651:errorcluster, "reference out"=w3653:refnum<k7>)  [unwired: 3 in, 1 out]
                    n2113 = call "OAExecute.vi"("script"=w3640, "Error IO"=w3651, "Origin.IOApplication"=w3653) -> ()  [unwired: 1 in, 3 out]
                  }
                  frame #6 {
                    n2114 = local read "X Axis Display Type"() -> (w3658:string)
                    n2115 = local read "Opj X Axis"() -> (w3663:string)
                    n2116 = call "Param_Analysis_7_24b_JW.vi"("Independant Variable"=w3666, "error in (no error)"=w3669, "Data Folder"=w3667, "Parameter String"="STS-Sat (V/decade):", "Parameter Name"="STS-Sat", "Stats Folder"=w3668) -> ("error out"=w3673:errorcluster, "Output Array"=w3671:string[][], "Variables"=w3665:T20)  [unwired: 2 in, 1 out]
                    n2117 = Concatenate Strings("window -a SGraph;\nlayer.x.type=", w3663, "; layer.x.label.numFormat = ", w3658, "; Y3 = 1; X3 = 1;", "window -a STable;\nwindow -s TV;") -> (w3661:string)
                    n2118 = call "Origin_Export_7_27a_JW.vi"("Input Conditions"=w3665, "Analysis Array"=w3671, "error in (no error)"=w3673, "Parameter Worksheet Name"="[STable]Threshold Swing", "Parameter Folder Script"="pe_cd \"STS-Sat\";", "Origin.IOApplication"=w3670) -> ("error out"=w3672:errorcluster, "reference out"=w3674:refnum<k7>)  [unwired: 3 in, 1 out]
                    n2119 = call "OAExecute.vi"("script"=w3661, "Error IO"=w3672, "Origin.IOApplication"=w3674) -> ()  [unwired: 1 in, 3 out]
                  }
                  frame #7 {
                    n2120 = local read "X Axis Display Type"() -> (w3679:string)
                    n2121 = local read "Opj X Axis"() -> (w3684:string)
                    n2122 = Concatenate Strings("window -a VtGraph;\nlayer.x.type=", w3684, "; layer.x.label.numFormat = ", w3679, "; Y3 = 1; X3 = 1;", "window -a VtTable;\nwindow -s TV;") -> (w3682:string)
                    n2123 = call "Param_Analysis_7_24b_JW.vi"("Independant Variable"=w3687, "error in (no error)"=w3692, "Data Folder"=w3690, "Parameter String"="Vt-Sat (V):", "Parameter Name"="Vt-Sat", "Stats Folder"=w3691) -> ("error out"=w3696:errorcluster, "Output Array"=w3694:string[][], "Variables"=w3686:T20)  [unwired: 2 in, 1 out]
                    n2124 = call "Origin_Export_7_27a_JW.vi"("Input Conditions"=w3686, "Analysis Array"=w3694, "error in (no error)"=w3696, "Parameter Worksheet Name"="[VtTable]Threshold Voltages", "Parameter Folder Script"="pe_cd \"Vt-Sat\";", "Origin.IOApplication"=w3693) -> ("error out"=w3695:errorcluster, "reference out"=w3697:refnum<k7>)  [unwired: 3 in, 1 out]
                    n2125 = call "OAExecute.vi"("script"=w3682, "Error IO"=w3695, "Origin.IOApplication"=w3697) -> ("Error IO Out"=w3688:errorcluster, "Origin.IOApplication"=w3689:refnum<k7>)  [unwired: 1 in, 1 out]
                  }
                }
                n2126 = Path To String(path=w3517) -> (string=w3516:string)
                n2127 = call "OAExecute.vi"("script"="pe_cd /; ", "Error IO"=w3512, "Origin.IOApplication"=w3511) -> ("Error IO Out"=w3518:errorcluster, "Origin.IOApplication"=w3519:refnum<k7>)  [unwired: 1 in, 1 out]
                n2128 = call <userlib>:"OASaveProject.vi"("path"=w3516, "Error IO"=w3518, "Origin.IOApplication"=w3519) -> ()  [unwired: 3 out]
              }
            }
          }
          event "Blank Button": Mouse Down {
            n2129 = event-data() -> ()  [unwired: 1 in, 7 out]
            n2130 = local read "Transfer File"() -> (w3712:path)
            n2131 = disable-structure shown="Disabled" {
              frame Disabled {
                n2132 = local read "Folder Index"() -> (w3713:dbl)
                n2133 = Decrement(x=w3713) -> (x-1=w3714:dbl)
                n2134 = local write "Folder Index"(w3714) -> ()
              }
              frame Enabled {
              }
            }
            n2135 = Strip Path(path=w3712) -> (stripped path=w3708:path, name=w3710:string)
            n2136 = Path To String(path=w3708) -> (string=w3707:string)
            n2137 = Concatenate Strings(w3707, "\\", "X_", w3710) -> (w3706:string)
            n2138 = String To Path(string=w3706) -> (path=w3705:path)
            n2139 = Move(source path=w3712, 10:w3705) -> ()  [unwired: 3 in, 3 out]
            n2140 = local write "Transfer File"(w3705) -> ()
          }
          event "Cancel Button": Mouse Down {
            (unwired) 6
            n2141 = event-data() -> ()  [unwired: 1 in, 7 out]
            n2142 = call "Simulate_Keyboard.vi"("Action"=2, "Virtual Key"=162) -> ()  [unwired: 7 in, 1 out]
          }
        }
        n2143 = Multiply(x=w495, y=10) -> (x*y=w497:sgl)
        n2144 = case shown="\"0\"" w536 {
          tunnel: w510 -> [w675 w681 w685 w687 w691 w693 w695 w697 w699 w701 w703 w705 w707 w709 w711 w713 w715 w717 w719 w721 w723 w725 w727 w729 w731 w733 w735 w737 w739 w741 w743 w745 w747 w749 w751 w753 w755 w757 w759 w761 w763 w765 w767 w769 w771 w773 w775 w777 w779 w781 w783 w785 w787 w789 w791 w793 w795 w797 w799 w801 w803 w805 w807 w809 w811 w813 w815 w817 w819 w821 w823 w825 w827 w829 w831 w833 w835 w837 w839 w841 w843 w845 w847 w849 w851 w853 w855 w857 w859 w861 w863 w865 w867 w869 w871 w873 w875 w877 w879 w881 w883 w885 w887 w889 w891]
          tunnel: [w675 w680 w684 w687 w691 w693 w695 w697 w699 w701 w703 w705 w707 w709 w711 w713 w715 w717 w719 w721 w723 w725 w727 w729 w731 w733 w735 w737 w739 w741 w743 w745 w747 w749 w751 w753 w755 w757 w759 w761 w763 w765 w767 w769 w771 w773 w775 w777 w779 w781 w783 w785 w787 w789 w791 w793 w795 w797 w799 w801 w803 w805 w807 w809 w811 w813 w815 w817 w819 w821 w823 w825 w827 w829 w831 w833 w835 w837 w839 w841 w843 w845 w847 w849 w851 w853 w855 w857 w859 w861 w863 w865 w867 w869 w871 w873 w875 w877 w879 w881 w883 w885 w887 w889 w891] -> w535
          tunnel: w511 -> [w677 w679 w683 w689 w690 w692 w694 w696 w698 w700 w702 w704 w706 w708 w710 w712 w714 w716 w718 w720 w722 w724 w726 w728 w730 w732 w734 w736 w738 w740 w742 w744 w746 w748 w750 w752 w754 w756 w758 w760 w762 w764 w766 w768 w770 w772 w774 w776 w778 w780 w782 w784 w786 w788 w790 w792 w794 w796 w798 w800 w802 w804 w806 w808 w810 w812 w814 w816 w818 w820 w822 w824 w826 w828 w830 w832 w834 w836 w838 w840 w842 w844 w846 w848 w850 w852 w854 w856 w858 w860 w862 w864 w866 w868 w870 w872 w874 w876 w878 w880 w882 w884 w886 w888 w890]
          tunnel: [w676 w679 w683 w688 w690 w692 w694 w696 w698 w700 w702 w704 w706 w708 w710 w712 w714 w716 w718 w720 w722 w724 w726 w728 w730 w732 w734 w736 w738 w740 w742 w744 w746 w748 w750 w752 w754 w756 w758 w760 w762 w764 w766 w768 w770 w772 w774 w776 w778 w780 w782 w784 w786 w788 w790 w792 w794 w796 w798 w800 w802 w804 w806 w808 w810 w812 w814 w816 w818 w820 w822 w824 w826 w828 w830 w832 w834 w836 w838 w840 w842 w844 w846 w848 w850 w852 w854 w856 w858 w860 w862 w864 w866 w868 w870 w872 w874 w876 w878 w880 w882 w884 w886 w888 w890] -> w534
          tunnel: w497 -> [w674 w678 w682 w686 _ _ _ _ _ _ _ _ _ _ _ _ _ _ _ _ _ _ _ _ _ _ _ _ _ _ _ _ _ _ _ _ _ _ _ _ _ _ _ _ _ _ _ _ _ _ _ _ _ _ _ _ _ _ _ _ _ _ _ _ _ _ _ _ _ _ _ _ _ _ _ _ _ _ _ _ _ _ _ _ _ _ _ _ _ _ _ _ _ _ _ _ _ _ _ _ _ _ _ _ _]
          frame "DOWN" {
            n2145 = Add(x=w677, y=w674) -> (x+y=w676:sgl)
          }
          frame "LEFT" {
            n2146 = Subtract(x=w681, y=w678) -> (x-y=w680:sgl)
          }
          frame "RIGHT" {
            n2147 = Add(x=w685, y=w682) -> (x+y=w684:sgl)
          }
          frame "UP" {
            n2148 = Subtract(x=w689, y=w686) -> (x-y=w688:sgl)
          }
          frame "ENTER (num pad)" {
          }
          frame "' (quote)" {
          }
          frame "END" {
          }
          frame "EQUALS" {
          }
          frame "ESCAPE" {
          }
          frame "GRAVE (`)" {
          }
          frame "HOME" {
          }
          frame "INSERT" {
          }
          frame "LBRACKET" {
          }
          frame "LCONTROL" {
          }
          frame "L ALT" {
          }
          frame "LSHIFT" {
          }
          frame "LWIN" {
          }
          frame "MINUS" {
          }
          frame "MULTIPLY" {
          }
          frame "NEXT" {
          }
          frame "NUMLOCK" {
          }
          frame "NUMPAD_0" {
          }
          frame "NUMPAD_1" {
          }
          frame "NUMPAD_2" {
          }
          frame "NUMPAD_3" {
          }
          frame "NUMPAD_4" {
          }
          frame "NUMPAD_5" {
          }
          frame "NUMPAD_6" {
          }
          frame "NUMPAD_7" {
          }
          frame "NUMPAD_8" {
          }
          frame "NUMPAD_9" {
          }
          frame "PAUSE" {
          }
          frame "PERIOD" {
          }
          frame "PRIOR (PG UP)" {
          }
          frame "RBRACKET" {
          }
          frame "RCONTROL" {
          }
          frame "RETURN" {
          }
          frame "R ALT" {
          }
          frame "RSHIFT" {
          }
          frame "RWIN" {
          }
          frame "SCROLL" {
          }
          frame "SEMICOLON" {
          }
          frame "SLASH" {
          }
          frame "SPACE" {
          }
          frame "SUBTRACT" {
          }
          frame "TAB" {
          }
          frame "DIVIDE" {
          }
          frame "DELETE" {
          }
          frame "DECIMAL" {
          }
          frame "COMMA" {
          }
          frame "CAPITAL" {
          }
          frame "BACKSLASH" {
          }
          frame "BACK" {
          }
          frame "ADD" {
          }
          frame "F15" {
          }
          frame "F14" {
          }
          frame "F13" {
          }
          frame "F12" {
          }
          frame "F11" {
          }
          frame "F10" {
          }
          frame "F9" {
          }
          frame "F8" {
          }
          frame "F7" {
          }
          frame "F6" {
          }
          frame "F5" {
          }
          frame "F4" {
          }
          frame "F3" {
          }
          frame "F2" {
          }
          frame "F1" {
          }
          frame "Z" {
          }
          frame "Y" {
          }
          frame "X" {
          }
          frame "W" {
          }
          frame "V" {
          }
          frame "U" {
          }
          frame "T" {
          }
          frame "S" {
          }
          frame "R" {
          }
          frame "Q" {
          }
          frame "P" {
          }
          frame "O" {
          }
          frame "N" {
          }
          frame "M" {
          }
          frame "L" {
          }
          frame "K" {
          }
          frame "J" {
          }
          frame "I" {
          }
          frame "H" {
          }
          frame "G" {
          }
          frame "F" {
          }
          frame "E" {
          }
          frame "D" {
          }
          frame "C" {
          }
          frame "B" {
          }
          frame "A" {
          }
          frame "9" {
          }
          frame "8" {
          }
          frame "7" {
          }
          frame "6" {
          }
          frame "5" {
          }
          frame "4" {
          }
          frame "3" {
          }
          frame "2" {
          }
          frame "1" {
          }
          frame "0" {
          }
        }
        n2149 = Bundle(w513, w512, w527, w526, 0.0) -> (w525:cluster{dbl, dbl, dbl, dbl, dbl})  [unwired: 1 in]
        n2150 = Bundle("X"=w535, "Y"=w534) -> (w529:cluster{"X":sgl, "Y":sgl})  [unwired: 1 in]
        n2151 = Divide(x=20, y=w496) -> (x/y=w499:sgl)
        n2152 = property on="Image Out" class="ImageControl"("Image Center Position"=w529) -> ()  [unwired: 2 in, 2 out]
        n2153 = call "IMAQ Convert Rectangle to ROI (Polygon)"("Rectangle"=w525) -> ("ROI Descriptor"=w523:T4)  [unwired: 7 in, 2 out]
        n2154 = Bundle("Application Font", w499, w503, w503, w503, w503, w503, TRUE, w501) -> (w505:T21)  [unwired: 1 in]
        n2155 = property on="Image Out 2" class="ImageControl"("ROI"=w523) -> ()  [unwired: 2 in, 2 out]
        n2156 = Bundle(w501, w505, w501, w501) -> (w504:T22)  [unwired: 1 in]
        n2157 = property on="Image Out" class="ImageControl"() -> ("ROI"=w488:T14)  [unwired: 2 in, 2 out]
        n2158 = Unbundle By Name(w488) -> ("Contours"=w552:T18)
        n2159 = local read "Image Out"() -> (w507:T2)
        n2160 = call "IMAQ Clear Overlay"("Image"=w507) -> ("Image Out"=w506:T2)  [unwired: 9 in, 1 out]
        n2161 = Initialize Array(0) -> (w550:i32[])  [unwired: 1 in]
        n2162 = local read "Magnification"() -> (w541:u16)
        n2163 = Array Size(array=w552) -> (size(s)=w551:i32)
        n2164 = Build Array(0.505025, 0.252522, 0.127742, 0.050345, 0.031129) -> (w542:dbl[])
        n2165 = Array Subset(array=w542, index=w541, length=1) -> (w539:dbl[])
        n2166 = property on="Image Out" class="ImageControl"() -> ("ZoomInteger"=w531:cluster{"X":i32, "Y":i32})  [unwired: 2 in, 2 out]
        n2167 = To Double Precision Float(number=w539) -> (double precision float=w538:dbl[])
        n2168 = for {
          N: w551 -> [_]
          shift-right: [w914] -> _
          shift-left: w552 -> [w914]
          shift-right: [w912] -> w537
          shift-left: w550 -> [w911]
          tunnel: w538 -> [w910]
          shift-right: [w907] -> _
          shift-left: w506 -> [w909]
          tunnel: w504 -> [w902]
          i -> [w906]
          n2169 = Index Array(array=w914, index=w906) -> (element=w923:T23)
          n2170 = Unbundle(w923) -> ("Points"=w922:i32[])  [unwired: 2 out]
          n2171 = Array To Cluster(array=w922) -> (cluster=w921:T24)
          n2172 = Unbundle(w921) -> ("Points[0]"=w901:i32, "Points[1]"=w898:i32, "Points[2]"=w913:i32, "Points[3]"=w919:i32)  [unwired: 5 out]
          n2173 = Add(x=w901, y=10) -> (x+y=w899:i32)
          n2174 = Subtract(x=w898, y=w919) -> (x-y=w918:i32)
          n2175 = Subtract(x=w901, y=w913) -> (x-y=w920:i32)
          n2176 = Square(x=w918) -> (x^2=w916:i32)
          n2177 = Square(x=w920) -> (x^2=w917:i32)
          n2178 = Add(x=w917, y=w916) -> (x+y=w915:i32)
          n2179 = Square Root(x=w915) -> (sqrt(x)=w892:dbl)
          n2180 = Multiply(x=w892, y=0.5) -> (x*y=w895:dbl)
          n2181 = Add(x=w895, y=w898) -> (x+y=w897:dbl)
          n2182 = Bundle(w899, w897) -> (w908:cluster{i32, dbl})  [unwired: 1 in]
          n2183 = Multiply(x=w892, y=w910) -> (x*y=w905:dbl[])
          n2184 = Index Array(array=w905) -> (element=w904:dbl)  [unwired: 1 in]
          n2185 = Number To Fractional String(number=w904) -> (F-format string=w903:string)  [unwired: 3 in]
          n2186 = call "IMAQ Overlay Text"("BG Color (Transparent)"=u32 0, "Text Color (black)"=u32 16448250, "Font, Size & Style"=w902, "String"=w903, "Origin"=w908, "Image"=w909) -> ("Image Out"=w907:T2)  [unwired: 4 in, 1 out]
          n2187 = Build Array (concatenate)(w911, w905) -> (w912:dbl[])
          n2188 = local write "Numeric 3"(w892) -> ()
        }
        n2189 = local write "ROI Descriptor"(w488) -> ()
        n2190 = Unbundle(w531) -> ("X"=w530:i32)  [unwired: 1 out]
        n2191 = Add Array Elements(numeric array=w537) -> (sum=w548:dbl)
        n2192 = local write "Distances"(w537) -> ()
        n2193 = local write "Total Width"(w548) -> ()
        n2194 = local write "Zoom"(w530) -> ()
        n2195 = local read "Manual-Width"() -> (w454:bool)
        n2196 = local read "Total Width"() -> (w491:dbl)
        n2197 = local read "Rec: Width"() -> (w489:dbl)
        n2198 = case shown="False" w454 {
          frame False {
            n2199 = property on="New: Width" class="DigNum (strict)"("DisabledEnum"=1) -> ()  [unwired: 2 in, 2 out]
          }
          frame True {
            n2200 = property on="New: Width" class="DigNum (strict)"("DisabledEnum"=0) -> ()  [unwired: 2 in, 2 out]
          }
        }
        n2201 = Not(x=w454) -> (.not. x?=w486:bool)
        n2202 = Equal To 0?(x=w491) -> (x = 0?=w487:bool)
        n2203 = Or(x=w487, y=w454) -> (x .or. y?=w490:bool)
        n2204 = And(x=w487, y=w486) -> (x .and. y?=w485:bool)
        n2205 = case shown="True" w485 {
          tunnel: w489 -> [_ w650]
          frame False {
          }
          frame True {
            n2206 = local write "New: Width"(w650) -> ()
          }
        }
        n2207 = case shown="False" w490 {
          tunnel: w491 -> [w652 _]
          frame False {
            n2208 = local write "New: Width"(w652) -> ()
            n2209 = property on="New: Width" class="DigNum (strict)"("DisabledEnum"=1) -> ()  [unwired: 2 in, 2 out]
          }
          frame True {
            n2210 = property on="New: Width" class="DigNum (strict)"("DisabledEnum"=0) -> ()  [unwired: 2 in, 2 out]
          }
        }
        n2211 = local read "Manual Comments"() -> (w455:bool)
        n2212 = local read "Rec: Comments"() -> (w456:string)
        n2213 = local read "Manuel-Dielectric"() -> (w482:bool)
        n2214 = local read "Rec: Dielectric (d)"() -> (w481:dbl)
        n2215 = local read "Manuel-Length"() -> (w483:bool)
        n2216 = local read "Rec: Length"() -> (w484:dbl)
        n2217 = case shown="True" w455 {
          tunnel: w456 -> [w633 _]
          frame False {
            n2218 = local write "Comments:"(w633) -> ()
            n2219 = property on="Comments:" class="Str"("DisabledEnum"=1) -> ()  [unwired: 2 in, 2 out]
          }
          frame True {
            n2220 = property on="Comments:" class="Str"("DisabledEnum"=0) -> ()  [unwired: 2 in, 2 out]
          }
        }
        n2221 = case shown="True" w483 {
          tunnel: w484 -> [w648 _]
          frame False {
            n2222 = local write "New: Length"(w648) -> ()
            n2223 = property on="New: Length" class="DigNum (strict)"("DisabledEnum"=1) -> ()  [unwired: 2 in, 2 out]
          }
          frame True {
            n2224 = property on="New: Length" class="DigNum (strict)"("DisabledEnum"=0) -> ()  [unwired: 2 in, 2 out]
          }
        }
        n2225 = case shown="True" w482 {
          tunnel: w481 -> [w645 _]
          frame False {
            n2226 = local write "New: Dielectric"(w645) -> ()
            n2227 = property on="New: Dielectric" class="DigNum (strict)"("DisabledEnum"=1) -> ()  [unwired: 2 in, 2 out]
          }
          frame True {
            n2228 = property on="New: Dielectric" class="DigNum (strict)"("DisabledEnum"=0) -> ()  [unwired: 2 in, 2 out]
          }
        }
      }
    }
  }
  n2229 = disable-structure shown="Disabled" {
    frame Disabled {
      # "Transformer Work"
      n2230 = Build Array("DeviceID", "Fabricator", "Deposition", "Date", "Sample", "Row", "Column", "L (um)", "W (um)", "Material", "Treatment", "TC (mM)", "Solvent", "C (%)", "ST (C)", "Drops", "Wait (s)", "RT (F)", "RH (%)", "Ramp (s)", "RPM", "Accel (RPM/s)", "Time (s)", "Mobility", "On/Off", "Vt", "S.T.S") -> (→"Transformer \nHeaders":string[])
    }
    frame Enabled {
    }
  }
